vi "mainAuto.vi"() -> ()   [LabVIEW 2018]
uses:
  <vilib>/Analysis/baseanly.llb/Mean (DBL).vi
  #include/Global_1259.vi
  <userlib>/_OpenG.lib/array/array.llb/Filter 1D Array with Scalar (String)__ogtk.vi
  <userlib>/_OpenG.lib/array/array.llb/Filter 1D Array with Scalar (Boolean)__ogtk.vi
  <vilib>/Analysis/NI_AALBase.lvlib
panel:
  out "index 2":i32
  out "random 2":i32
  out "random":i32
  out "index":i32
  out "appended array":i16[](array[numeric])
  out "min(x,y)":i16
  out "max(x,y)":i16
  out "valueResistance":dbl
  out "resLower":dbl
  out "resUpper":dbl
  out "resistanceArray":dbl[](array[numeric])
  out "speedArray":dbl[](array[numeric])
  out "inclineArray":dbl[](array[numeric])
  out "negative incline":dbl
  out "FAN":string
  out "fanType":string
  out "refnum out":refnum<file>
  in  "Tab Control":T1(tab)
  out "Welcome to Console Test":picture
  out "Version":string[](array[string])
  in  "Inspection Point":string(combo)
  in  "PO Line Number":string
  in  "PO Number":string
  in  "Inspector Name":string
  in  "Work Station":string
  in  "Vendor Name":string
  in  "Vendor Number":string
  out "Initialize Test":string
  out "Config and Fixture Setup":string
  out "Firmware Reference":string
  in  "EQF1259 com port":refnum<visa-resource-name>
  out "Console Number":string
  out "Console Name":string
  in  "scanSerial":string
  out "resultSerial":bool
  out "PartNumber":string
  in  "Cos0":bool
  in  "Cos1":bool
  out "COSMETIC-3, 4":string
  in  "Con1":bool
  out "FIXTURE_SETUP-1":string
  out "Connection":picture
  out "Voltage":string
  out "Power On":cluster{dbl, dbl}(graph)
  out "Current":string
  out "POWER_UP-5, 6":string
  in  "Pow0":bool
  in  "Pow1":bool
  out "PowerOn":bool
  out "CurrentOn":bool
  out "CurrentPeak":string
  out "limitON":bool
  out "CurrentMax":string
  out "PowerMode":string="Battery"
  out "BLE_SETUP-2":string
  out "BLE_CONNECT-7":string
  out "BLE PASS":bool
  out "Cal1":bool
  in  "Dis1":bool
  in  "Dis0":bool
  out "MAINTENANCE MODE-8, 9, 10, 11":string
  in  "Enter Firmware":string
  out "Firmware":bool
  in  "Key0":bool
  in  "Key1":bool
  out "SPM AEROBIC":dbl(knob) scale=0.0..200.0
  in  "stopP":bool
  out "SPEED":dbl(knob) scale=0.0..10.1 scale format="%.1g"
  out "MAX":string
  out "PWM_RPM":string
  out "SPEED AEROBIC":dbl(knob) scale=0.0..25.0
  out "RPM AEROBIC":dbl(knob) scale=0.0..200.0
  in  "Tac0":bool
  in  "Tac1":bool
  out "Quickspeed":bool
  out "Minus\nButton":bool
  out "Plus\nButton":bool
  out "ONE\nButton":bool
  out "PWM PASS":bool
  out "PWM hz":string
  out "PWM %":string
  out "Elapsed Time (s)":dbl
  out "Press Next":dbl format="%#_13g"
  out "Decrease":bool
  out "Increase":bool
  out "Least":bool
  out "RESISTANCE-15":string
  out "QuickResistance":bool
  out "RESISTANCE/CURRENT":cluster{dbl, dbl}(graph)
  out "IRun":string
  out "IPeak":string
  out "Press Next":dbl
  out "RESISTANCE PASS":bool
  out "overCurrent":bool
  in  "stopR":bool
  out "currentMaxResistance":string
  out "BLE PULSE":u32(graph)
  out "BLE_BPM":u32
  out "PULSE-17":string
  out "Hand/Thumb Pass":bool
  out "BLE_HRM Pass":bool
  in  "E-stopHRM":bool
  in  "PUL0":bool
  in  "PUL1":bool
  out "BLE Status":u32
  out "FanCurrent":dbl(graph)
  in  "FAN0":bool
  in  "FAN1":bool
  out "Ifan":string
  out "limitFan":bool
  out "currentMaxFan":string
  out "FAN-18":string
  out "fanIPeak":string
  in  "AUD0 2":bool
  in  "AUD1 2":bool
  out "Iaudio":string
  out "AudioCurrent":dbl(graph)
  in  "AUD0":bool
  out "currentMaxAudio":string
  out "AUDIO-19":string
  out "audioIPeak":string
  in  "AUD1":bool
  out "limitAudio":bool
  in  "TV1":bool
  in  "TV0":bool
  out "TVCurrent":dbl(graph)
  out "Itv":string
  out "limitTV":bool
  out "currentMaxTV":string
  out "TV-20":string
  out "tvIPeak":string
  out "limitUSB":bool
  out "Iusb":string
  in  "USB1":bool
  in  "USB0":bool
  out "currentMaxUSB":string
  out "USBCurrent":dbl(graph)
  out "USB-16":string
  out "usbIPeak":string
  in  "stopI":bool
  out "incline":dbl(graph)
  out "INCLINE PASS":bool
  out "INCLINE-14":string
  out "Quickincline":bool
  out "Down":bool
  out "Up":bool
  out "ZERO":bool
  out "MAX":dbl
  out "MIN":dbl
  out "Press Next":dbl
  out "limitCSafe":bool
  out "Icsafe":string
  in  "CSA1":bool
  in  "CSA0":bool
  out "currentMaxCSafe":string
  out "CSafeCurrent":dbl(graph)
  out "CSAFE-21":string
  out "csafeIPeak":string
  out "limitWahoo":bool
  out "Iwahoo":string
  in  "WAH1":bool
  in  "WAH0":bool
  out "currentMaxWahoo":string
  out "WahooCurrent":dbl(graph)
  out "WAHOO-22":string
  out "wahooIPeak":string
  in  "ANO0":bool
  in  "ANO1":bool
  out "Another":picture
  out "# of Samples":i32
  out "# of Failed Samples":i32
  out "# of Passed Samples":i32
  out "Failed":picture
  out "Test Log":string
  out "Goodbye!":picture
  out "standard notepad":string
  out "standard labviewdbupload":string
  in  "FIN0":bool
  out "FINISH-25":string
  # "Does Cosmetic Pass Inspection?"
  # "Scan Console Serial Number"
  # "Is The Harness Connected Correctly?"
  # "Did Console Power ON?"
  # "Calibrate?"
  # "Display?"
  # "Key Code?"
  # "Did The Hand/Thumb Pulse Pass?"
  # "Did The Fan Function Well?"
  # "BLE Audio"
  # "Aux Audio"
  # "NOT USED. SEE BLE CONNECT AND PULSE FOR DATA."
  # "Would You Like To Test Another Console?"
  # "Console Failed Test!"
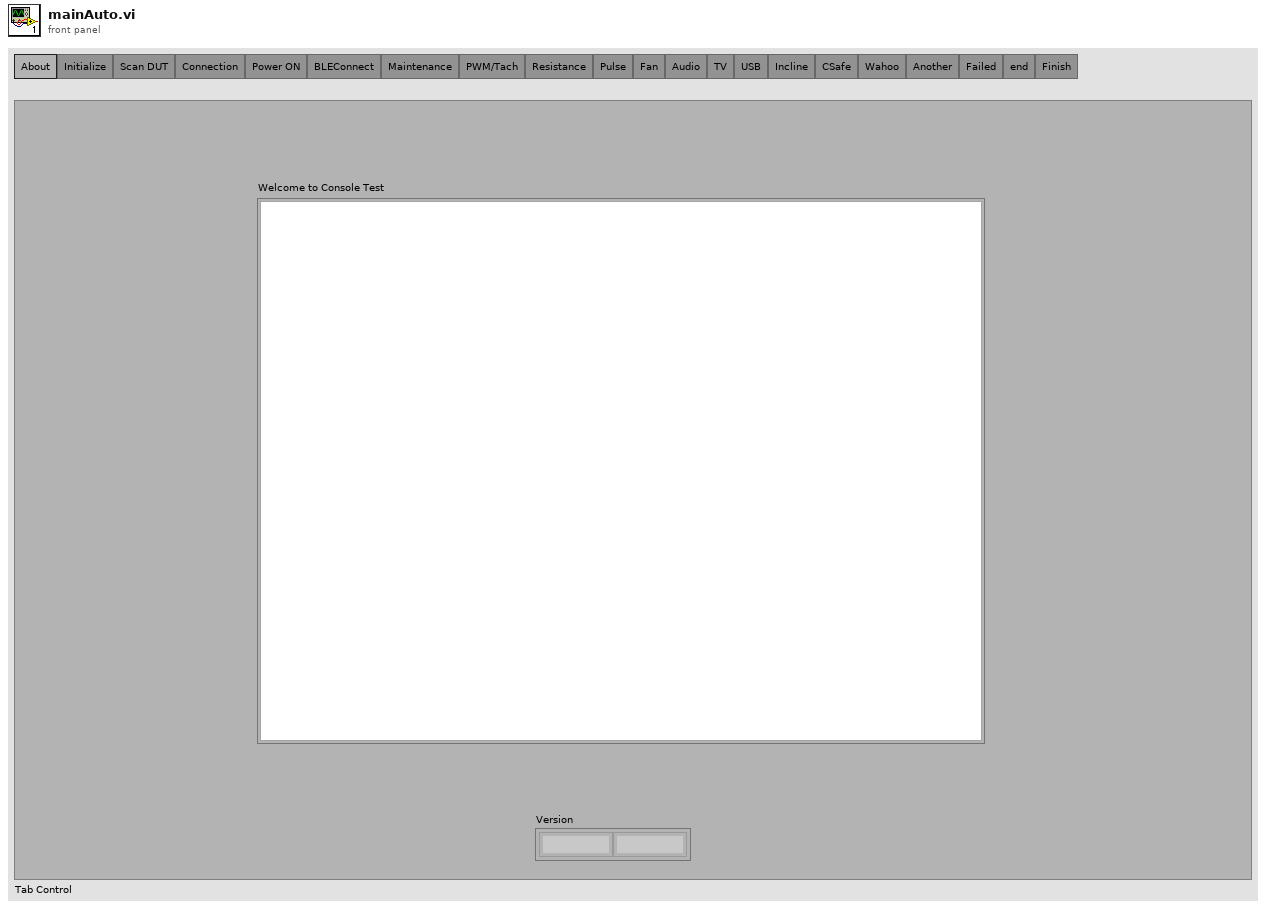
[diagram p1: front panel]
types:
  T1 = enum32{"About", "Initialize", "Scan DUT", "Connection", "Power ON", "BLEConnect", "Maintenance", "PWM/Tach", "Resistance", "Pulse", "Fan", "Audio", "TV", "USB", "Incline", "CSafe", "Wahoo", "Another", "Failed", "end", "Finish"}
  T2 = enum32{"Interactive applications", "Built-in command line utilities", "Executable command line utilities"}
  T3 = enum32{"About", "Initialize", "Scan DUT", "Connection", "Power ON", "BLEConnect", "Maintenance", "PWM/Tach", "Resistance", "Pulse", "Fan", "Audio", "TV", "USB", "Incline", "CSafe", "Wahoo", "Another", "Failed", "end"}
  T4 = enum16{"Flow", "User", "Station", "Vendor", "Number", "PO #", "PO Line#", "Record"}
  T5 = enum16{"name", "number", "device", "firmware", "mcu", "display", "grade", "resistance", "distance", "pulse"}
  T6 = enum16{"verifyHand_Thumb", "startBLE_HRM", "readBLE_HRM", "statusBLE_HRM"}
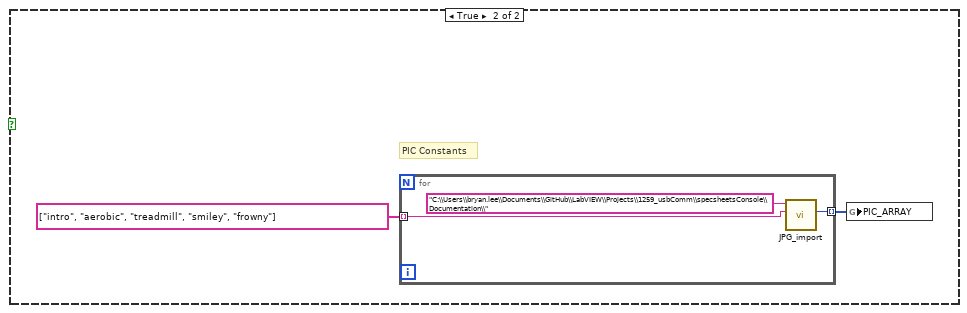
[diagram p3: hidden frame]
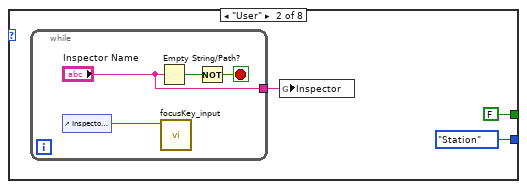
[diagram p5: hidden frame]
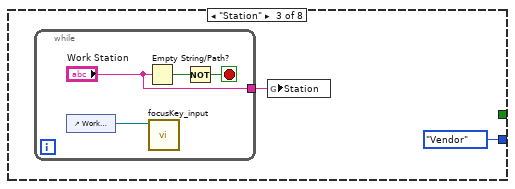
[diagram p6: hidden frame]
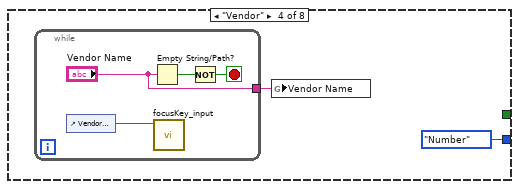
[diagram p7: hidden frame]
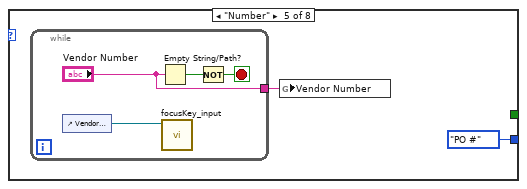
[diagram p8: hidden frame]
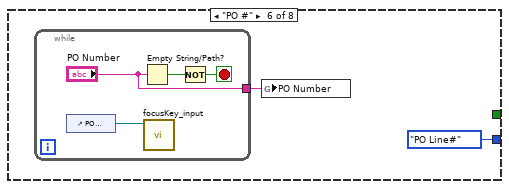
[diagram p9: hidden frame]
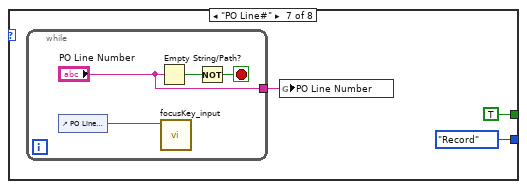
[diagram p10: hidden frame]
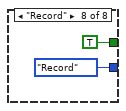
[diagram p11: hidden frame]
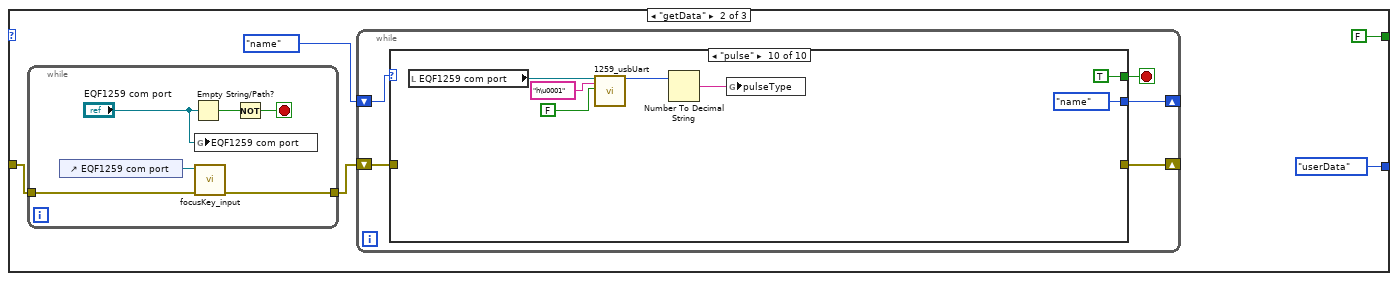
[diagram p12: hidden frame]
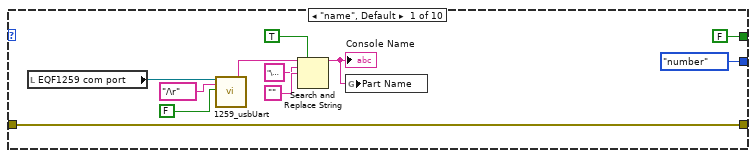
[diagram p13: hidden frame]
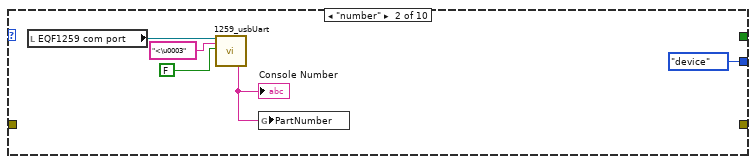
[diagram p14: hidden frame]
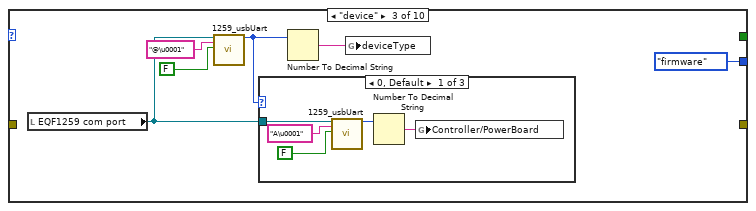
[diagram p15: hidden frame]
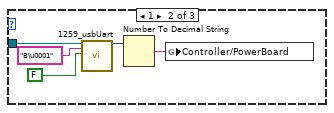
[diagram p16: hidden frame]
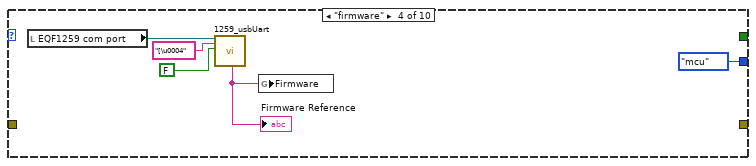
[diagram p18: hidden frame]
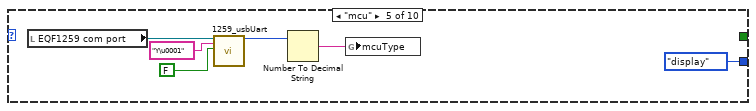
[diagram p19: hidden frame]
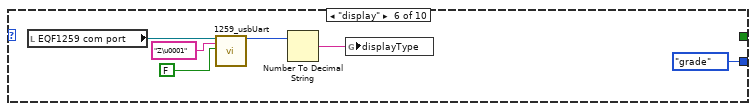
[diagram p20: hidden frame]
diagram:
  w1 = 0
  # "About\nInitialize\nScan DUT\nConnection\nPower On\nMaintenance\nSpeed/Distance\nIncline\nResistance\nFeatures\nExtra Features\nAnother\nFailed\nend"
  n1 = while {
    shift-right: [w3] -> _
    shift-left: "Tab Control" -> [w9]
    shift-right: [w5] -> _
    shift-left: w1 -> [w7]
    shift-right: [w4] -> _
    shift-left: w1 -> [w6]
    stop <- w10 stop-if-true
    n2 = property on="Tab Control" class="TabCtl (strict)"("Value"=w9) -> ("Value"=w8:T1)  [unwired: 2 in, 2 out]
    n3 = case shown="\"PWM/Tach\"" w8 {
      tunnel: [FALSE _ _ _ _ _ _ w533 w914 _ _ _ _ _ _ _ _ _ _ TRUE _] -> w10
      tunnel: [w13 T3."Connection" ("Tab Control") w225 w270 w301 w356 w422 w534 w916 w1357 w2246 w2365 w2473 w2657 w2719 w2764 w2805 w2842 T1."Finish" ("Tab Control") T3."end" ("Tab Control") w2903] -> w3
      tunnel: w7 -> [w12 w50 w218 w273 w296 w353 w419 w530 w911 w1353 w2240 w2352 w2470 w2650 w2713 w2753 w2798 w2833 w2854 w2863 w2905]
      tunnel: w6 -> [w11 w49 w223 w272 w295 w352 w418 w529 w905 w1352 w2239 w2351 w2469 w2649 w2712 w2760 w2797 w2832 w2856 w2862 w2904]
      tunnel: [w12 w50 w224 w273 w296 w353 w419 w530 w911 w1353 w2240 w2352 w2470 w2650 w2713 w2753 w2798 w2833 w2854 w2863 w2905] -> w5
      tunnel: [w11 w49 w223 w272 w295 w352 w418 w529 w905 w1352 w2239 w2351 w2469 w2649 w2712 w2760 w2797 w2832 w2855 w2862 w2904] -> w4
      frame "About", Default {
        n4 = for {
          N: 1 -> [_]
          w17 = FALSE ("Visible")
          w18 = 0
          n5 = global write "Global_1259.vi" "tempNumeric"(0.0 ("tempNumeric")) -> ()
          n6 = global write "Global_1259.vi" "tempBoolean"(FALSE) -> ()
          n7 = global write "Global_1259.vi" "tempString"("" ("tempString")) -> ()
          n8 = local write "# of Samples"(w18) -> ()
          n9 = local write "# of Failed Samples"(w18) -> ()
          n10 = case shown="False" FALSE {
            frame False {
              w32 = "\""
              # "Opens procedure"
              n11 = global read "Global_1259.vi" "PIC_ARRAY"() -> (w29:picture[])
              n12 = global read "Global_1259.vi" "Version"() -> (w22:string[][])
              n13 = Index Array(array=w29, index=0) -> (element=→"Welcome to Console Test":picture)
              n14 = for {
                N: 3 -> [_]
                tunnel: w22 -> [w39]
                tunnel: [w38] -> w25 mode=indexing
                i -> [w37]
                n15 = Index Array(array=w39, index (row)=21 ("disabled index (row)"), index (col)=w37) -> (element=w38:string)
              }
              n16 = Reshape Array(w25, 2 ("dimension size")) -> (→"Version":string[])
              n17 = call <vilib>:"Space Constant.vi"() -> ("String"=w34:string)
              n18 = Concatenate Strings("C:\\Windows\\System32\\notepad.exe" ("Command"), w34, w32, "C:\\specsheetsConsole\\Documentation\\Console(Chinese).txt" ("string"), w32) -> (w35:string)
              n19 = call "exeCLI.vi"("Tab Control"=T2."Interactive applications", "command line (interactive)"=w35) -> ()  [unwired: 11 in, 3 out]
            }
            frame True {
              # "PIC Constants"
              n20 = for {
                tunnel: [w43] -> w41 mode=indexing
                tunnel: string[] ["intro", "aerobic", "treadmill", "smiley", "frowny"] -> [w42] mode=indexing
                n21 = call "JPG_import.vi"("File name"=w42, "File path"="C:\\Users\\bryan.lee\\Documents\\GitHub\\LabVIEW\\Projects\\1259_usbComm\\specsheetsConsole\\Documentation\\") -> ("new picture"=w43:picture)  [unwired: 7 in, 2 out]
              }
              n22 = global write "Global_1259.vi" "PIC_ARRAY"(w41) -> ()
            }
          }
          n23 = property on="speedArray" class="Arr (strict)"("Visible"=w17) -> ()  [unwired: 2 in, 2 out]
          n24 = property on="resistanceArray" class="Arr (strict)"("Visible"=w17) -> ()  [unwired: 2 in, 2 out]
          n25 = property on="inclineArray" class="Arr (strict)"("Visible"=w17) -> ()  [unwired: 2 in, 2 out]
        }
        n26 = while {
          tunnel: [T3."Initialize" ("Tab Control")] -> w13
          stop <- TRUE stop-if-true
          n27 = Wait (ms)(milliseconds to wait=u32 1500) -> ()  [unwired: 1 out]
        }
      }
      frame "Initialize" {
        # "used for debugging"
        n28 = for {
          N: 2 -> [_]
          tunnel: [w56] -> w52
          w54 = ""
          n29 = local write "Work Station"(w54) -> ()
          n30 = global write "Global_1259.vi" "mcuType"(w54) -> ()
          n31 = global write "Global_1259.vi" "Controller/PowerBoard"(w54) -> ()
          n32 = global write "Global_1259.vi" "Firmware"(w54) -> ()
          n33 = global write "Global_1259.vi" "PartNumber"(w54) -> ()
          n34 = local write "Vendor Name"(w54) -> ()
          n35 = local write "Vendor Number"(w54) -> ()
          n36 = local write "PO Number"(w54) -> ()
          n37 = local write "PO Line Number"(w54) -> ()
          n38 = local write "Console Name"(w54) -> ()
          n39 = local write "Console Number"(w54) -> ()
          n40 = local write "Firmware Reference"(w54) -> ()
          n41 = global write "Global_1259.vi" "Part Name"(w54) -> ()
          n42 = global write "Global_1259.vi" "deviceType"(w54) -> ()
          n43 = local write "Inspector Name"(w54) -> ()
          n44 = local write "Inspection Point"(w54) -> ()
          n45 = local write "EQF1259 com port"(refnum<visa-resource-name> refnum ("VISA resource name")) -> ()
          n46 = call <vilib>:"Simple Error Handler.vi"() -> ("error out"=w56:errorcluster)  [unwired: 5 in, 4 out]
          "Initialize Test" <- "\u0006\\&^\tgMneöNvm\u0000i\u0000c\u0000r\u0000o\u0000S\u0000D\u0000ÒceQE\u0000Q\u0000F\u00001\u00002\u00005\u00009\u0000\u00020\n\u0000\u0000_/TE\u0000Q\u0000F\u00001\u00002\u00005\u00009\u0000\u00020\n\u0000(WE\u0000Q\u0000F\u00001\u00002\u00005\u00009\u0000\nN\fÿ\tébv^ R}cknxvMneöN\u00020\n\u0000(W\u000bNbvh<h\nNkXQáOo`\u00020\n\u0000\tébE\u0000Q\u0000F\u00001\u00002\u00005\u00009\u0000\u001a¯ïzãS\u00020\n\u0000I\u0000n\u0000s\u0000e\u0000r\u0000t\u0000 \u0000m\u0000i\u0000c\u0000r\u0000o\u0000S\u0000D\u0000 \u0000w\u0000i\u0000t\u0000h\u0000 \u0000p\u0000r\u0000o\u0000f\u0000i\u0000l\u0000e\u0000 \u0000i\u0000n\u0000t\u0000o\u0000 \u0000E\u0000Q\u0000F\u00001\u00002\u00005\u00009\u0000.\u0000\n\u0000T\u0000u\u0000r\u0000n\u0000 \u0000o\u0000n\u0000 \u0000E\u0000Q\u0000F\u00001\u00002\u00005\u00009\u0000.\u0000\n\u0000O\u0000n\u0000 \u0000t\u0000h\u0000e\u0000 \u0000E\u0000Q\u0000F\u00001\u00002\u00005\u00009\u0000,\u0000 \u0000s\u0000e\u0000l\u0000e\u0000c\u0000t\u0000 \u0000a\u0000n\u0000d\u0000 \u0000l\u0000o\u0000a\u0000d\u0000 \u0000t\u0000h\u0000e\u0000 \u0000c\u0000o\u0000r\u0000r\u0000e\u0000c\u0000t\u0000 \u0000c\u0000o\u0000n\u0000f\u0000i\u0000g\u0000u\u0000r\u0000a\u0000t\u0000i\u0000o\u0000n\u0000 \u0000f\u0000i\u0000l\u0000e\u0000.\u0000\n\u0000F\u0000i\u0000l\u0000l\u0000 \u0000o\u0000u\u0000t\u0000 \u0000t\u0000h\u0000e\u0000 \u0000i\u0000n\u0000f\u0000o\u0000r\u0000m\u0000a\u0000t\u0000i\u0000o\u0000n\u0000 \u0000o\u0000n\u0000 \u0000t\u0000h\u0000e\u0000 \u0000f\u0000o\u0000r\u0000m\u0000 \u0000b\u0000e\u0000l\u0000o\u0000w\u0000.\u0000\n\u0000S\u0000e\u0000l\u0000e\u0000c\u0000t\u0000 \u0000t\u0000h\u0000e\u0000 \u0000E\u0000Q\u0000F\u00001\u00002\u00005\u00009\u0000 \u0000c\u0000o\u0000m\u0000m\u0000u\u0000n\u0000i\u0000c\u0000a\u0000t\u0000i\u0000o\u0000n\u0000 \u0000p\u0000o\u0000r\u0000t\u0000.\u0000"
          "Config and Fixture Setup" <- "\u0006\\5un¿~Þ¥c0RE\u0000Q\u0000F\u00001\u00002\u00005\u00009\u0000\u00020\n\u0000¾nopwQMn\u001aÿ\n\u0000O(uP\u0000C\u0000\u0006\\.\u0000x\u0000m\u0000l\u0000MneöN R}0Rm\u0000i\u0000c\u0000r\u0000o\u0000S\u0000D\u0000aS-N\fÿåeöN(WR\u0000N\u0000D\u0000f\u0000t\u0000p\u0000-Nv§c6RðS\rTðy\u000bN~b0R\bÿOY\u001aÿ& R\u0000N\u0000D\u0000F\u0000t\u0000p\u0000 \u0000\\\u0000 \u0000E\u0000B\u0000N\u0000T\u00000\u00002\u00001\u00001\u00007\u0000 \u0000\\\u0000 \u0000P\u0000r\u0000o\u0000c\u0000e\u0000d\u0000u\u0000r\u0000e\u0000\tÿ\u00020\n\u0000\u0006\\m\u0000i\u0000c\u0000r\u0000o\u0000S\u0000D\u0000aSb\u001dg\nNÒceQm\u0000i\u0000c\u0000r\u0000o\u0000S\u0000D\u0000aSÒcýi-N\u00020\n\u0000Sb\u0000_opwQÌbvR\u0000E\u0000S\u0000E\u0000T\u0000\tc®\u00020\n\u0000O(u\u0011T\nNT\u0011T\u000bN\tc®~b0RcknxvMneöN\u00020\n\u0000\tcE\u0000N\u0000T\u0000E\u0000R\u0000\tébMneöN\bÿO\\U^1\u0000\tÿ\u00020\n\u0000S_O\\U^3z[öe\fÿ÷I{_5\u0000Òy\fÿY\u000bN@b:y\u00020\n\u0000¾n9YwQ\t²Q\u001aÿ\n\u0000\tcE\u0000Q\u0000F\u00001\u00002\u00005\u00009\u0000 \u00002\u0000x\u0000\nNvD\u0000i\u0000s\u0000p\u0000l\u0000a\u0000y\u0000\u00020\n\u0000(WdkopwQ\nN\tc\u0000_ËY\n\u0000O(u\u0011T\nNT\u0011T\u000bN\tc®¾n:g\t²Q\u00020\n\u0000(WopwQ\nN\tc\u0000_ËY\u00020\n\u0000\tc\u0000N!k>f:y\u00020\n\u0000C\u0000o\u0000n\u0000n\u0000e\u0000c\u0000t\u0000 \u0000t\u0000h\u0000e\u0000 \u0000p\u0000o\u0000w\u0000e\u0000r\u0000 \u0000..."
        }
        n47 = while {
          shift-right: [w60] -> _
          shift-left: enum16{"getData", "userData", "recordData"}."getData" -> [w62]
          tunnel: w52 -> [w59]
          stop <- w61 stop-if-true
          n48 = case shown="\"userData\", Default" w62 {
            tunnel: [FALSE FALSE TRUE] -> w61
            tunnel: [enum16{"getData", "userData", "recordData"}."recordData" enum16{"getData", "userData", "recordData"}."userData" enum16{"getData", "userData", "recordData"}."recordData"] -> w60
            tunnel: w59 -> [_ w117 _]
            frame "userData", Default {
              n49 = while {
                shift-right: [w66] -> _
                shift-left: T4."Flow" -> [w67]
                stop <- w68 stop-if-true
                n50 = case shown="\"Flow\", Default" w67 {
                  tunnel: [_ FALSE _ _ _ _ TRUE TRUE] -> w68
                  tunnel: [T4."User" T4."Station" T4."Vendor" T4."Number" T4."PO #" T4."PO Line#" T4."Record" T4."Record"] -> w66
                  frame "Flow", Default {
                    n51 = while {
                      tunnel: ["Inspection Point"] -> w70
                      stop <- w72 stop-if-true
                      n52 = control-ref of="Inspection Point"() -> (w74:refnum<vi>)
                      n53 = Empty String/Path?(string/path="Inspection Point") -> (empty?=w73:bool)
                      n54 = call "focusKey_input.vi"("reference"=w74) -> ()  [unwired: 10 in, 1 out]
                      n55 = Not(x=w73) -> (.not. x?=w72:bool)
                    }
                    n56 = global write "Global_1259.vi" "Inspection Point"(w70) -> ()
                  }
                  frame "User" {
                    n57 = while {
                      tunnel: ["Inspector Name"] -> w76
                      stop <- w80 stop-if-true
                      n58 = control-ref of="Inspector Name"() -> (w79:refnum<vi>)
                      n59 = Empty String/Path?(string/path="Inspector Name") -> (empty?=w81:bool)
                      n60 = call "focusKey_input.vi"("reference"=w79) -> ()  [unwired: 10 in, 1 out]
                      n61 = Not(x=w81) -> (.not. x?=w80:bool)
                    }
                    n62 = global write "Global_1259.vi" "Inspector"(w76) -> ()
                  }
                  frame "Station" {
                    n63 = while {
                      tunnel: ["Work Station"] -> w83
                      stop <- w86 stop-if-true
                      n64 = control-ref of="Work Station"() -> (w85:refnum<vi>)
                      n65 = Empty String/Path?(string/path="Work Station") -> (empty?=w87:bool)
                      n66 = call "focusKey_input.vi"("reference"=w85) -> ()  [unwired: 10 in, 1 out]
                      n67 = Not(x=w87) -> (.not. x?=w86:bool)
                    }
                    n68 = global write "Global_1259.vi" "Station"(w83) -> ()
                  }
                  frame "Vendor" {
                    n69 = while {
                      tunnel: ["Vendor Name"] -> w89
                      stop <- w92 stop-if-true
                      n70 = control-ref of="Vendor Name"() -> (w91:refnum<vi>)
                      n71 = Empty String/Path?(string/path="Vendor Name") -> (empty?=w93:bool)
                      n72 = call "focusKey_input.vi"("reference"=w91) -> ()  [unwired: 10 in, 1 out]
                      n73 = Not(x=w93) -> (.not. x?=w92:bool)
                    }
                    n74 = global write "Global_1259.vi" "Vendor Name"(w89) -> ()
                  }
                  frame "Number" {
                    n75 = while {
                      tunnel: ["Vendor Number"] -> w95
                      stop <- w98 stop-if-true
                      n76 = control-ref of="Vendor Number"() -> (w97:refnum<vi>)
                      n77 = Empty String/Path?(string/path="Vendor Number") -> (empty?=w99:bool)
                      n78 = call "focusKey_input.vi"("reference"=w97) -> ()  [unwired: 10 in, 1 out]
                      n79 = Not(x=w99) -> (.not. x?=w98:bool)
                    }
                    n80 = global write "Global_1259.vi" "Vendor Number"(w95) -> ()
                  }
                  frame "PO #" {
                    n81 = while {
                      tunnel: ["PO Number"] -> w101
                      stop <- w104 stop-if-true
                      n82 = control-ref of="PO Number"() -> (w103:refnum<vi>)
                      n83 = Empty String/Path?(string/path="PO Number") -> (empty?=w105:bool)
                      n84 = call "focusKey_input.vi"("reference"=w103) -> ()  [unwired: 10 in, 1 out]
                      n85 = Not(x=w105) -> (.not. x?=w104:bool)
                    }
                    n86 = global write "Global_1259.vi" "PO Number"(w101) -> ()
                  }
                  frame "PO Line#" {
                    n87 = while {
                      tunnel: ["PO Line Number"] -> w107
                      stop <- w110 stop-if-true
                      n88 = control-ref of="PO Line Number"() -> (w112:refnum<vi>)
                      n89 = Empty String/Path?(string/path="PO Line Number") -> (empty?=w111:bool)
                      n90 = call "focusKey_input.vi"("reference"=w112) -> ()  [unwired: 10 in, 1 out]
                      n91 = Not(x=w111) -> (.not. x?=w110:bool)
                    }
                    n92 = global write "Global_1259.vi" "PO Line Number"(w107) -> ()
                  }
                  frame "Record" {
                  }
                }
              }
            }
            frame "getData" {
              n93 = while {
                tunnel: [w122] -> w118
                tunnel: w117 -> [w121]
                stop <- w123 stop-if-true
                n94 = control-ref of="EQF1259 com port"() -> (w125:refnum<vi>)
                n95 = Empty String/Path?(string/path="EQF1259 com port") -> (empty?=w124:bool)
                n96 = global write "Global_1259.vi" "EQF1259 com port"("EQF1259 com port") -> ()
                n97 = call "focusKey_input.vi"("error in (no error)"=w121, "reference"=w125) -> ("error out"=w122:errorcluster)  [unwired: 9 in]
                n98 = Not(x=w124) -> (.not. x?=w123:bool)
              }
              n99 = while {
                shift-right: [w126] -> _
                shift-left: T5."name" -> [w127]
                shift-right: [w128] -> _
                shift-left: w118 -> [w129]
                stop <- w130 stop-if-true
                n100 = case shown="\"pulse\"" w127 {
                  tunnel: [FALSE _ _ _ _ _ _ _ _ TRUE] -> w130
                  tunnel: w129 -> [w138 _ _ _ _ _ _ _ _ _]
                  tunnel: [T5."number" T5."device" T5."firmware" T5."mcu" T5."display" T5."grade" T5."resistance" T5."distance" T5."pulse" T5."name"] -> w126
                  tunnel: [w138 _ _ _ _ _ _ _ _ _] -> w128
                  frame "name", Default {
                    n101 = local read "EQF1259 com port"() -> (w139:refnum<visa-resource-name>)
                    n102 = call "1259_usbUart.vi"("VISA resource name"=w139, "write buffer"="/\r" ("write buffer buffer"), "sdFeature"=FALSE) -> ("valid byte"=w137:string)  [unwired: 1 in, 15 out]
                    n103 = Search and Replace String(replace all?=TRUE ("replace all? (F)"), input string=w137, search string="\u0000", replace string="") -> (result string=w134:string)  [unwired: 4 in, 3 out]
                    "Console Name" <- w134
                    n104 = global write "Global_1259.vi" "Part Name"(w134) -> ()
                  }
                  frame "number" {
                    n105 = local read "EQF1259 com port"() -> (w145:refnum<visa-resource-name>)
                    n106 = call "1259_usbUart.vi"("VISA resource name"=w145, "write buffer"="<\u0003" ("write buffer buffer"), "sdFeature"=FALSE) -> ("PartNumber"=w144:string)  [unwired: 1 in, 15 out]
                    "Console Number" <- w144
                    n107 = global write "Global_1259.vi" "PartNumber"(w144) -> ()
                  }
                  frame "device" {
                    n108 = local read "EQF1259 com port"() -> (w148:refnum<visa-resource-name>)
                    n109 = call "1259_usbUart.vi"("VISA resource name"=w148, "write buffer"="@\u0001" ("write buffer buffer"), "sdFeature"=FALSE) -> ("number[0]"=w149:u32)  [unwired: 1 in, 15 out]
                    n110 = case shown="0, Default" w149 {
                      tunnel: w148 -> [w154 w161 _]
                      frame 0, Default {
                        n111 = call "1259_usbUart.vi"("VISA resource name"=w154, "write buffer"="A\u0001" ("write buffer buffer"), "sdFeature"=FALSE) -> ("number[0]"=w157:u32)  [unwired: 1 in, 15 out]
                        n112 = Number To Decimal String(number=w157) -> (decimal integer string=w156:string)  [unwired: 1 in]
                        n113 = global write "Global_1259.vi" "Controller/PowerBoard"(w156) -> ()
                      }
                      frame 1 {
                        n114 = call "1259_usbUart.vi"("VISA resource name"=w161, "write buffer"="B\u0001", "sdFeature"=FALSE) -> ("number[0]"=w159:u32)  [unwired: 1 in, 15 out]
                        n115 = Number To Decimal String(number=w159) -> (decimal integer string=w160:string)  [unwired: 1 in]
                        n116 = global write "Global_1259.vi" "Controller/PowerBoard"(w160) -> ()
                      }
                      frame 3 {
                        # "Rower_Basic"
                      }
                    }
                    n117 = Number To Decimal String(number=w149) -> (decimal integer string=w152:string)  [unwired: 1 in]
                    n118 = global write "Global_1259.vi" "deviceType"(w152) -> ()
                  }
                  frame "firmware" {
                    n119 = local read "EQF1259 com port"() -> (w167:refnum<visa-resource-name>)
                    n120 = call "1259_usbUart.vi"("VISA resource name"=w167, "write buffer"="[\u0004", "sdFeature"=FALSE) -> ("BB FW"=w163:string)  [unwired: 1 in, 15 out]
                    "Firmware Reference" <- w163
                    n121 = global write "Global_1259.vi" "Firmware"(w163) -> ()
                  }
                  frame "mcu" {
                    n122 = local read "EQF1259 com port"() -> (w171:refnum<visa-resource-name>)
                    n123 = call "1259_usbUart.vi"("VISA resource name"=w171, "write buffer"="Y\u0001", "sdFeature"=FALSE) -> ("number[0]"=w173:u32)  [unwired: 1 in, 15 out]
                    n124 = Number To Decimal String(number=w173) -> (decimal integer string=w170:string)  [unwired: 1 in]
                    n125 = global write "Global_1259.vi" "mcuType"(w170) -> ()
                  }
                  frame "display" {
                    n126 = local read "EQF1259 com port"() -> (w176:refnum<visa-resource-name>)
                    n127 = call "1259_usbUart.vi"("VISA resource name"=w176, "write buffer"="Z\u0001", "sdFeature"=FALSE) -> ("number[0]"=w179:u32)  [unwired: 1 in, 15 out]
                    n128 = Number To Decimal String(number=w179) -> (decimal integer string=w177:string)  [unwired: 1 in]
                    n129 = global write "Global_1259.vi" "displayType"(w177) -> ()
                  }
                  frame "grade" {
                    n130 = local read "EQF1259 com port"() -> (w181:refnum<visa-resource-name>)
                    n131 = call "1259_usbUart.vi"("VISA resource name"=w181, "write buffer"=" \u0001", "sdFeature"=FALSE) -> ("number[0]"=w185:u32)  [unwired: 1 in, 15 out]
                    n132 = Number To Decimal String(number=w185) -> (decimal integer string=w183:string)  [unwired: 1 in]
                    n133 = global write "Global_1259.vi" "gradeType"(w183) -> ()
                  }
                  frame "resistance" {
                    n134 = local read "EQF1259 com port"() -> (w187:refnum<visa-resource-name>)
                    n135 = call "1259_usbUart.vi"("VISA resource name"=w187, "write buffer"="¡\u0001", "sdFeature"=FALSE) -> ("number[0]"=w190:u32)  [unwired: 1 in, 15 out]
                    n136 = Number To Decimal String(number=w190) -> (decimal integer string=w191:string)  [unwired: 1 in]
                    n137 = global write "Global_1259.vi" "resistanceType"(w191) -> ()
                  }
                  frame "distance" {
                    n138 = local read "EQF1259 com port"() -> (w193:refnum<visa-resource-name>)
                    n139 = call "1259_usbUart.vi"("VISA resource name"=w193, "write buffer"="›\u0001", "sdFeature"=FALSE) -> ("number[0]"=w197:u32)  [unwired: 1 in, 15 out]
                    n140 = Number To Decimal String(number=w197) -> (decimal integer string=w195:string)  [unwired: 1 in]
                    n141 = global write "Global_1259.vi" "distanceType"(w195) -> ()
                  }
                  frame "pulse" {
                    n142 = local read "EQF1259 com port"() -> (w200:refnum<visa-resource-name>)
                    n143 = call "1259_usbUart.vi"("VISA resource name"=w200, "write buffer"="h\u0001", "sdFeature"=FALSE) -> ("number[0]"=w204:u32)  [unwired: 1 in, 15 out]
                    n144 = Number To Decimal String(number=w204) -> (decimal integer string=w202:string)  [unwired: 1 in]
                    n145 = global write "Global_1259.vi" "pulseType"(w202) -> ()
                  }
                }
              }
            }
            frame "recordData" {
              # "loads the feature array"
              n146 = local read "EQF1259 com port"() -> (w212:refnum<visa-resource-name>)
              n147 = call "1259_usbUart.vi"("VISA resource name"=w212, "write buffer"="P\u0002", "sdFeature"=TRUE) -> ("error out"=w206:errorcluster)  [unwired: 1 in, 15 out]
              n148 = global read "Global_1259.vi" "Part Name"() -> (w208:string)
              n149 = call "Header data_Cnsl.vi"("base path"=path "C:/", "prompt (Create Folder)"="logsConsole", "file name"=w208, "Error In"=w206) -> ("refnum out"=→"refnum out":refnum<file>)  [unwired: 10 in, 1 out]
            }
          }
        }
      }
      frame "Scan DUT" {
        w221 = FALSE
        w228 = ""
        n150 = Increment(x=w218) -> (x+1=w224:i32)
        "# of Samples" <- w224
        n151 = local write "scanSerial"(w228) -> ()
        n152 = local write "PartNumber"(w228) -> ()
        n153 = local write "Cos0"(w221) -> ()
        n154 = local write "Cos1"(w221) -> ()
        n155 = local write "resultSerial"(w221) -> ()
        n156 = local read "refnum out"() -> (w219:refnum<file>)
        n157 = call "User data_Cnsl.vi"("refnum in"=w219) -> ("error out"=w220:errorcluster)  [unwired: 7 in, 1 out]
        n158 = call "cosmeticPIP.vi"("error in (no error)"=w220) -> ("error out"=w216:errorcluster)  [unwired: 9 in, 1 out]
        n159 = flat-sequence {
          tunnel: w216 -> [w233]
          tunnel: [w233] -> w215
          frame #0 {
            n160 = global read "Global_1259.vi" "COSMETIC-3, 4"() -> (w230:string)
            n161 = Concatenate Strings(w230, "kbÏcïSeRagb_\u0001x\u0007h~{\u00020\n\u0000S\u0000c\u0000a\u0000n\u0000 \u0000t\u0000h\u0000e\u0000 \u0000p\u0000e\u0000e\u0000l\u0000a\u0000b\u0000l\u0000e\u0000 \u0000b\u0000a\u0000r\u0000c\u0000o\u0000d\u0000e\u0000 \u0000l\u0000a\u0000b\u0000e\u0000l\u0000.\u0000\n\u0000") -> (→"COSMETIC-3, 4":string)
          }
        }
        n162 = while {
          tunnel: [w267] -> w229
          tunnel: [w261] -> w222
          tunnel: w215 -> [w260]
          stop <- w268 stop-if-true
          n163 = control-ref of="scanSerial"() -> (w266:refnum<vi>)
          n164 = Empty String/Path?(string/path="scanSerial") -> (empty?=w269:bool)
          n165 = Search/Split String(string="scanSerial", offset (0)=6) -> (substring before match=w265:string)  [unwired: 1 in, 2 out]
          n166 = call "focusKey_input.vi"("error in (no error)"=w260, "reference"=w266) -> ("error out"=w267:errorcluster)  [unwired: 9 in]
          n167 = global read "Global_1259.vi" "PartNumber"() -> (w264:string)
          "PartNumber" <- w264
          n168 = Not(x=w269) -> (.not. x?=w268:bool)
          n169 = Equal?(x=w265, y=w264) -> (x = y?=w261:bool)
          "resultSerial" <- w261
        }
        n170 = case shown="True" w222 {
          tunnel: w229 -> [_ w240]
          tunnel: [FALSE w237] -> w217
          frame False {
          }
          frame True {
            n171 = flat-sequence {
              tunnel: w240 -> [w243]
              tunnel: [w242] -> w239
              tunnel: [w241] -> w238
              tunnel: w239 -> [_]
              tunnel: w238 -> [w251]
              tunnel: [w249] -> w235
              frame #0 {
                n172 = local read "scanSerial"() -> (w245:string)
                n173 = Reverse String(1:w245) -> (0:w247:string)
                n174 = Search/Split String(string=w247, offset (0)=11) -> (substring before match=w248:string)  [unwired: 1 in, 2 out]
                n175 = local read "refnum out"() -> (w241:refnum<file>)
                n176 = Reverse String(1:w248) -> (0:w244:string)
                n177 = call "Serial data.vi"("error in"=w243, "Serial Number"=w244, "refnum in"=w241) -> ("error out"=w242:errorcluster)  [unwired: 7 in, 1 out]
              }
              frame #1 {
                n178 = while {
                  tunnel: [w255] -> w250
                  stop <- w258 stop-if-true
                  n179 = Not(x="Cos0") -> (.not. x?=w259:bool)
                  n180 = Or(x="Cos1", y="Cos0") -> (x .or. y?=w258:bool)
                  n181 = And(x="Cos1", y=w259) -> (x .and. y?=w255:bool)
                }
                n182 = case shown="True" w250 {
                  selector: w250 -> [w252 w253]
                  tunnel: w251 -> [_ w254]
                  tunnel: [w252 w253] -> w249
                  frame False {
                  }
                  frame True {
                    n183 = call "Pass_Fail.vi"("OK"=w253, "Byte Stream File in"=w254) -> ()  [unwired: 8 in, 2 out]
                  }
                }
              }
            }
            n184 = And(x=TRUE, y=w235) -> (x .and. y?=w237:bool)
          }
        }
        n185 = Select(t=T3."Power ON" ("Tab Control"), s=w217, f=T3."Failed" ("Tab Control")) -> (s? t:f=w225:T3)
      }
      frame "Connection" {
        n186 = call "controllerVoltage.vi"() -> ("error out"=w271:errorcluster)  [unwired: 11 in]
        n187 = local write "Con1"(FALSE) -> ()
        n188 = call "controllerPIP.vi"("error in (no error)"=w271) -> ("error out"=w274:errorcluster)  [unwired: 10 in, 4 out]
        n189 = global read "Global_1259.vi" "deviceType"() -> (w275:string)
        n190 = case shown="\"1\"" w275 {
          tunnel: w274 -> [_ _ _]
          frame "0", Default {
            n191 = global read "Global_1259.vi" "PIC_ARRAY"() -> (w277:picture[])
            n192 = global read "Global_1259.vi" "FIXTURE_SETUP-1"() -> (→"FIXTURE_SETUP-1":string)
            n193 = Index Array(array=w277, index=2) -> (element=→"Connection":picture)
          }
          frame "1" {
            n194 = global read "Global_1259.vi" "PIC_ARRAY"() -> (w283:picture[])
            n195 = global read "Global_1259.vi" "FIXTURE_SETUP-1"() -> (w284:string)
            n196 = Index Array(array=w283, index=1) -> (element=w281:picture)
            n197 = local write "FIXTURE_SETUP-1"(w284) -> ()
            n198 = local write "Connection"(w281) -> ()
          }
          frame "2" {
            n199 = global read "Global_1259.vi" "PIC_ARRAY"() -> (w287:picture[])
            n200 = global read "Global_1259.vi" "FIXTURE_SETUP-1"() -> (w288:string)
            n201 = Index Array(array=w287, index=1) -> (element=w285:picture)
            n202 = local write "FIXTURE_SETUP-1"(w288) -> ()
            n203 = local write "Connection"(w285) -> ()
          }
        }
        n204 = while {
          tunnel: [T3."Scan DUT" ("Tab Control")] -> w270
          stop <- "Con1" stop-if-true
        }
      }
      frame "Power ON" {
        w293 = "0.00" ("Voltage")
        w294 = FALSE
        # "current cannot be used as a stop due to battery option"
        n205 = local write "Voltage"(w293) -> ()
        n206 = local write "Current"(w293) -> ()
        n207 = local write "CurrentPeak"(w293) -> ()
        n208 = global write "Global_1259.vi" "runCurrent"(w293) -> ()
        n209 = local write "CurrentMax"(w293) -> ()
        n210 = local write "Pow1"(w294) -> ()
        n211 = local write "Pow0"(w294) -> ()
        n212 = property on="Power On" class="WFChart (strict)"("History Data"=cluster{dbl, dbl}[] []) -> ()  [unwired: 2 in, 2 out]
        n213 = local write "PowerMode"("Off" ("runCurrent")) -> ()
        n214 = global read "Global_1259.vi" "POWER_UP-5, 6"() -> (→"POWER_UP-5, 6":string)
        n215 = local write "CurrentOn"(w294) -> ()
        n216 = local write "limitON"(w294) -> ()
        n217 = local write "PowerOn"(w294) -> ()
        n218 = stacked-sequence {
          tunnel: [_ w309] -> w291
          frame #0 {
            n219 = global read "Global_1259.vi" "EQF1259 com port"() -> (w302:refnum<visa-resource-name>)
            n220 = call "currentMax.vi"("VISA Refnum in"=w302) -> ("stringCurrentMax"=w303:string)  [unwired: 8 in, 2 out]
            n221 = global write "Global_1259.vi" "maxCurrent"(w303) -> ()
          }
          frame #1 {
            n222 = while {
              tunnel: [w336] -> w309
              tunnel: [w335] -> w306
              tunnel: [w334] -> w305
              stop <- w337 stop-if-true
              n223 = global read "Global_1259.vi" "EQF1259 com port"() -> (w312:refnum<visa-resource-name>)
              n224 = call "1259_usbUart.vi"("VISA resource name"=w312, "write buffer"="j\u0001", "sdFeature"=FALSE) -> ("number[0]"=w313:u32)  [unwired: 1 in, 15 out]
              n225 = case shown="1" w313 {
                frame 0, Default {
                  w338 = "Off" ("USB")
                  n226 = local write "PowerMode"(w338) -> ()
                  n227 = global write "Global_1259.vi" "PowerMode"(w338) -> ()
                }
                frame 1 {
                  w339 = "On" ("USB")
                  # "On"
                  n228 = local read "limitON"() -> (w344:bool)
                  n229 = local read "CurrentOn"() -> (w343:bool)
                  n230 = local read "PowerOn"() -> (w342:bool)
                  n231 = Not(x=w344) -> (.not. x?=w345:bool)
                  n232 = Compound Arithmetic op=OR(TRUE, w342, w343, w345) -> (w340:bool)
                  n233 = local write "PowerMode"(w339) -> ()
                  n234 = global write "Global_1259.vi" "PowerMode"(w339) -> ()
                  n235 = local write "Pow1"(w340) -> ()
                }
                frame 2 {
                  w346 = "Battery" ("USB")
                  # "Battery"
                  n236 = global write "Global_1259.vi" "PowerMode"(w346) -> ()
                  "PowerMode" <- w346
                }
              }
              n237 = global read "Global_1259.vi" "EQF1259 com port"() -> (w315:refnum<visa-resource-name>)
              n238 = global read "Global_1259.vi" "ConsoleVoltage"() -> (w317:string)
              n239 = global read "Global_1259.vi" "maxCurrent"() -> (w314:string)
              "CurrentMax" <- w314
              n240 = Fract/Exp String To Number(string=w317) -> (number=w316:dbl)  [unwired: 3 in, 1 out]
              n241 = call "voltageScan.vi"("VISA Refnum in"=w315) -> ("error out"=w329:errorcluster, "stringVoltage"=w334:string, "numberVoltage"=w324:dbl)  [unwired: 8 in]
              "Voltage" <- w334
              n242 = Greater?(x=w324, y=w316) -> (0:→"PowerOn":bool)
              n243 = call "currentScan.vi"("error in (no error)"=w329, "Imax"=w314, "VISA resource name"=w315) -> ("error out"=w328:errorcluster, "max"=w325:bool, "Istring"=w319:string, "Ichart"=w322:dbl)  [unwired: 5 in]
              "limitON" <- w325
              n244 = Compound Arithmetic op=OR("Pow1", "Pow0", w325) -> (w337:bool)
              n245 = Not(x="Pow0") -> (.not. x?=w332:bool)
              n246 = Not(x=w325) -> (.not. x?=w326:bool)
              n247 = call "currentPeak.vi"("error in (no error)"=w328, "Istring# change"=w319, "Istring# scan"=w319) -> ("Ipeak"=w335:string, "Irun"=→"Current":string)  [unwired: 6 in, 1 out]
              "CurrentPeak" <- w335
              n248 = Bundle("numberVoltage"=w324, "Ichart"=w322) -> (→"Power On":cluster{"\nnumberVoltage":dbl, "Ichart":dbl})  [unwired: 1 in]
              n249 = Greater?(x=w322, y=0.0) -> (0:→"CurrentOn":bool)
              n250 = Compound Arithmetic op=AND(TRUE ("value"), w326, "Pow1", w332) -> (w336:bool)
            }
            n251 = local read "refnum out"() -> (w307:refnum<file>)
            n252 = call "dataSampled.vi"("Data"=w305, "refnum in"=w307) -> ("error out"=w304:errorcluster, "refnum out"=w308:refnum<file>)  [unwired: 8 in]
            n253 = call "dataSampled.vi"("Error In"=w304, "Data"=w306, "refnum in"=w308) -> ()  [unwired: 7 in, 2 out]
          }
        }
        n254 = Select(t=T3."Maintenance" ("Tab Control"), s=w291, f=T3."Failed" ("Tab Control")) -> (s? t:f=w301:T3)
      }
      frame "BLEConnect" {
        n255 = local write "BLE PASS"(FALSE ("BLE PASS")) -> ()
        n256 = global read "Global_1259.vi" "Inspection Point"() -> (w349:string)
        n257 = Equal?(x=w349, y="SubAssembly") -> (x = y?=w347:bool)
        n258 = case shown="False" w347 {
          tunnel: [TRUE w362] -> w351
          frame True {
            n259 = local read "refnum out"() -> (w357:refnum<file>)
            n260 = call "dataSampled.vi"("refnum in"=w357) -> ()  [unwired: 9 in, 2 out]
          }
          frame False {
            n261 = global read "Global_1259.vi" "WAHOO"() -> (w361:string)
            n262 = Not Equal?(x=w361, y="1") -> (x != y?=w359:bool)
            n263 = case shown="True" w359 {
              tunnel: [w363 w388] -> w362
              frame False {
                w367 = 2 ("index (row)")
                # "ANT+ SamplerApp"
                n264 = global read "Global_1259.vi" "PIP_Instruction"() -> (w370:string[][])
                n265 = global write "Global_1259.vi" "pulseType"("16" ("pulseType")) -> ()
                n266 = Index Array(array=w370, index (row) #1=w367, index (col) #1=w367, index (row) #2=w367, index (col) #2=7 ("disabled index (col)")) -> (element #1=w365:string, element #2=w366:string)
                n267 = global write "Global_1259.vi" "BLE_SETUP-2"(w365) -> ()
                n268 = local write "BLE_SETUP-2"(w365) -> ()
                n269 = global write "Global_1259.vi" "BLE_CONNECT-7"(w366) -> ()
                n270 = local write "BLE_CONNECT-7"(w366) -> ()
                n271 = while {
                  tunnel: [w382] -> w364
                  stop <- w380 stop-if-true
                  n272 = local read "EQF1259 com port"() -> (w375:refnum<visa-resource-name>)
                  n273 = call "1259_usbUart.vi"("VISA resource name"=w375, "write buffer"="†\u0001") -> ("number[0]"=w377:u32)  [unwired: 2 in, 15 out]
                  n274 = Number To Decimal String(number=w377, width (-)=i16 0) -> (decimal integer string=w374:string)
                  n275 = Not Equal?(x=w374, y="0") -> (x != y?=w382:bool)
                  n276 = feedback #1() -> (w379:bool)  [unwired: 1 in]
                  n277 = call "Elapsed Time3"("Reset"=w379) -> ("Time has Elapsed"=w381:bool)  [unwired: 11 in, 7 out]
                  n278 = Or(x=w382, y=w381) -> (x .or. y?=w380:bool)
                  n279 = feedback-in #1(w380) -> ()
                }
                n280 = local write "BLE PASS"(w364) -> ()
                n281 = case shown="True" w364 {
                  selector: w364 -> [w371 w372]
                  tunnel: [w371 w372] -> w363
                  frame False {
                  }
                  frame True {
                    n282 = local read "refnum out"() -> (w373:refnum<file>)
                    n283 = call "Pass_Fail.vi"("OK"=w372, "Byte Stream File in"=w373) -> ()  [unwired: 8 in, 2 out]
                  }
                }
              }
              frame True {
                n284 = global read "Global_1259.vi" "TABLET"() -> (w386:string)
                n285 = Equal?(x=w386, y="0") -> (x = y?=w384:bool)
                n286 = case shown="True" w384 {
                  tunnel: [FALSE w390] -> w387
                  frame False {
                  }
                  frame True {
                    n287 = global read "Global_1259.vi" "BLE"() -> (w392:string)
                    n288 = Equal?(x=w392, y="1") -> (x = y?=w390:bool)
                  }
                }
                n289 = case shown="True" w387 {
                  tunnel: [TRUE w395] -> w388
                  frame False {
                    n290 = local read "refnum out"() -> (w394:refnum<file>)
                    n291 = call "dataSampled.vi"("refnum in"=w394) -> ()  [unwired: 9 in, 2 out]
                  }
                  frame True {
                    w397 = 1 ("index (row)")
                    # "BLE_CardioApp"
                    n292 = global read "Global_1259.vi" "PIP_Instruction"() -> (w402:string[][])
                    n293 = while {
                      tunnel: [w411] -> w396
                      stop <- w412 stop-if-true
                      n294 = local read "EQF1259 com port"() -> (w408:refnum<visa-resource-name>)
                      n295 = call "1259_usbUart.vi"("VISA resource name"=w408, "write buffer"="†\u0001") -> ("binary[0] String"=w406:string)  [unwired: 2 in, 15 out]
                      n296 = Not Equal?(x="0" ("y"), y=w406) -> (x != y?=w411:bool)
                      n297 = feedback #2() -> (w410:bool)  [unwired: 1 in]
                      n298 = call "Elapsed Time2"("Reset"=w410) -> ("Time has Elapsed"=w413:bool)  [unwired: 11 in, 7 out]
                      n299 = Or(x=w411, y=w413) -> (x .or. y?=w412:bool)
                      n300 = feedback-in #2(w412) -> ()
                    }
                    "BLE PASS" <- w396
                    n301 = Index Array(array=w402, index (row) #1=w397, index (col) #1=2 ("disabled index (col)"), index (row) #2=w397, index (col) #2=7 ("disabled index (col)")) -> (element #1=w401:string, element #2=w400:string)
                    "BLE_SETUP-2" <- w401
                    "BLE_CONNECT-7" <- w400
                    n302 = global write "Global_1259.vi" "BLE_SETUP-2"(w401) -> ()
                    n303 = global write "Global_1259.vi" "BLE_CONNECT-7"(w400) -> ()
                    n304 = case shown="True" w396 {
                      selector: w396 -> [w403 w404]
                      tunnel: [w403 w404] -> w395
                      frame False {
                      }
                      frame True {
                        n305 = local read "refnum out"() -> (w405:refnum<file>)
                        n306 = call "Pass_Fail.vi"("OK"=w404, "Byte Stream File in"=w405) -> ()  [unwired: 8 in, 2 out]
                      }
                    }
                  }
                }
              }
            }
          }
        }
        n307 = Select(t=T3."PWM/Tach" ("Tab Control"), s=w351, f=T3."Failed" ("Tab Control")) -> (s? t:f=w356:T3)
      }
      frame "Maintenance" {
        w414 = ""
        w417 = FALSE
        (unwired) FALSE
        n308 = local write "Enter Firmware"(w414) -> ()
        n309 = global write "Global_1259.vi" "BaseCurrent"(w414) -> ()
        n310 = local write "Cal1"(w417) -> ()
        n311 = local write "Dis1"(w417) -> ()
        n312 = local write "Key0"(w417) -> ()
        n313 = local write "Key1"(w417) -> ()
        n314 = local write "Dis0"(w417) -> ()
        n315 = local write "Firmware"(w417) -> ()
        n316 = while {
          shift-right: [w425] -> _
          shift-left: 0 -> [w426]
          tunnel: [w423] -> w420
          stop <- w424 stop-if-true
          n317 = case shown="3" w426 {
            tunnel: [1 2 3 4 5 6 _] -> w425
            tunnel: [FALSE FALSE FALSE w455 w484 w498 w512] -> w424
            tunnel: [FALSE FALSE FALSE w456 w485 w499 w513] -> w423
            frame 0, Default {
              n318 = local read "EQF1259 com port"() -> (w428:refnum<visa-resource-name>)
              n319 = call "1259_usbUart.vi"("VISA resource name"=w428, "write buffer"="\u0001", "sdFeature"=FALSE) -> ("PartNumber"=w437:string, "error out"=w427:errorcluster)  [unwired: 1 in, 14 out]
              n320 = global write "Global_1259.vi" "buttonType"(w437) -> ()
              n321 = call "1259_usbUart.vi"("VISA resource name"=w428, "write buffer"="š\u0001", "sdFeature"=FALSE, "error in (no error)"=w427) -> ("PartNumber"=w431:string)  [unwired: 15 out]
              n322 = global write "Global_1259.vi" "tabletType"(w431) -> ()
            }
            frame 1 {
              n323 = global read "Global_1259.vi" "GRADE"() -> (w441:string)
              n324 = case shown="\"0\"" w441 {
                frame "1", Default {
                  n325 = property on="Cal1" class="Bool (strict)"("Visible"=TRUE) -> ()  [unwired: 2 in, 2 out]
                }
                frame "0" {
                  n326 = local write "Cal1"(TRUE) -> ()
                  n327 = property on="Cal1" class="Bool (strict)"("Visible"=FALSE) -> ()  [unwired: 2 in, 2 out]
                }
              }
              n328 = call "maintenancePIP.vi"() -> ("MAINTENANCE MODE-8, 9, 10, 11"=→"MAINTENANCE MODE-8, 9, 10, 11":string)  [unwired: 10 in, 1 out]
            }
            frame 2 {
              n329 = while {
                tunnel: ["Enter Firmware"] -> w448
                stop <- w453 stop-if-true
                n330 = control-ref of="Enter Firmware"() -> (w452:refnum<vi>)
                n331 = Empty String/Path?(string/path="Enter Firmware") -> (empty?=w454:bool)
                n332 = call "focusKey_input.vi"("reference"=w452) -> ()  [unwired: 10 in, 1 out]
                n333 = Not(x=w454) -> (.not. x?=w453:bool)
                "Firmware" <- w453
              }
              n334 = local read "refnum out"() -> (w449:refnum<file>)
              n335 = call "dataSampled.vi"("Data"=w448, "refnum in"=w449) -> ()  [unwired: 8 in, 2 out]
            }
            frame 3 {
              n336 = local read "Cal1"() -> (w457:bool)
              n337 = case shown="False" w457 {
                tunnel: [FALSE w472] -> w456
                tunnel: [FALSE w471] -> w455
                frame True {
                  # "This is 1 second / per 10 samples"
                  n338 = while {
                    tunnel: [w470] -> w462 mode=indexing
                    i -> [w468]
                    stop <- w469 stop-if-true
                    n339 = local read "EQF1259 com port"() -> (w466:refnum<visa-resource-name>)
                    n340 = Equal?(x=25, y=w468) -> (x = y?=w469:bool)
                    n341 = call "currentScan.vi"("VISA resource name"=w466) -> ("Ichart"=w470:dbl)  [unwired: 7 in, 3 out]
                  }
                  n342 = local read "refnum out"() -> (w465:refnum<file>)
                  n343 = call-poly <vilib>:"Mean.vi"("X"=w462) -> ("mean"=w461:dbl)  [unwired: 1 out]
                  n344 = call "dataSampled.vi"("refnum in"=w465) -> ()  [unwired: 9 in, 2 out]
                  n345 = Number To Fractional String(number=w461, precision (6)=i16 2) -> (F-format string=w460:string)  [unwired: 2 in]
                  n346 = global write "Global_1259.vi" "BaseCurrent"(w460) -> ()
                }
                frame False {
                  n347 = flat-sequence {
                    tunnel: [w474] -> w473
                    tunnel: w473 -> [w478]
                    tunnel: [w477] -> w472
                    tunnel: [w476] -> w471
                    frame #0 {
                      # "engineer mode on fixture"
                      n348 = local read "EQF1259 com port"() -> (w475:refnum<visa-resource-name>)
                      n349 = call "inclineCalibrate.vi"("VISA Refnum in"=w475) -> ("Complete"=w474:bool)  [unwired: 8 in, 2 out]
                    }
                    frame #1 {
                      n350 = case shown="False" w478 {
                        selector: w478 -> [w480 w482]
                        tunnel: [w480 w482] -> w477
                        tunnel: [w479 w481] -> w476
                        frame False {
                          n351 = Not(x=w480) -> (.not. x?=w479:bool)
                        }
                        frame True {
                          n352 = Not(x=w482) -> (.not. x?=w481:bool)
                          n353 = local read "refnum out"() -> (w483:refnum<file>)
                          n354 = call "Pass_Fail.vi"("OK"=w482, "Byte Stream File in"=w483) -> ()  [unwired: 8 in, 2 out]
                        }
                      }
                      "Cal1" <- w478
                    }
                  }
                }
              }
            }
            frame 4 {
              n355 = while {
                tunnel: [w496] -> w486
                stop <- w495 stop-if-true
                n356 = Not(x="Dis0") -> (.not. x?=w497:bool)
                n357 = Or(x="Dis1", y="Dis0") -> (x .or. y?=w495:bool)
                n358 = And(x="Dis1", y=w497) -> (x .and. y?=w496:bool)
              }
              n359 = case shown="True" w486 {
                selector: w486 -> [w488 w491]
                tunnel: [w488 w491] -> w485
                tunnel: [w489 w490] -> w484
                frame False {
                  n360 = Not(x=w488) -> (.not. x?=w489:bool)
                }
                frame True {
                  n361 = Not(x=w491) -> (.not. x?=w490:bool)
                  n362 = local read "refnum out"() -> (w492:refnum<file>)
                  n363 = call "Pass_Fail.vi"("OK"=w491, "Byte Stream File in"=w492) -> ()  [unwired: 8 in, 2 out]
                }
              }
            }
            frame 5 {
              n364 = while {
                tunnel: [w510] -> w500
                stop <- w509 stop-if-true
                n365 = Not(x="Key0") -> (.not. x?=w511:bool)
                n366 = Or(x="Key1", y="Key0") -> (x .or. y?=w509:bool)
                n367 = And(x="Key1", y=w511) -> (x .and. y?=w510:bool)
              }
              n368 = case shown="True" w500 {
                selector: w500 -> [w503 w505]
                tunnel: [w503 w505] -> w499
                tunnel: [w502 w504] -> w498
                frame False {
                  n369 = Not(x=w503) -> (.not. x?=w502:bool)
                }
                frame True {
                  n370 = Not(x=w505) -> (.not. x?=w504:bool)
                  n371 = local read "refnum out"() -> (w506:refnum<file>)
                  n372 = call "Pass_Fail.vi"("OK"=w505, "Byte Stream File in"=w506) -> ()  [unwired: 8 in, 2 out]
                }
              }
            }
            frame 6 {
              n373 = while {
                tunnel: [w518] -> w513
                tunnel: [w517] -> w512
                stop <- w517 stop-if-true
                n374 = local read "Key1"() -> (w516:bool)
                n375 = local read "Cal1"() -> (w515:bool)
                n376 = local read "Dis1"() -> (w520:bool)
                n377 = Compound Arithmetic op=AND(TRUE ("value"), w515, w520, w516) -> (w518:bool)
                n378 = Not(x=w518) -> (.not. x?=w519:bool)
                n379 = Or(x=w518, y=w519) -> (x .or. y?=w517:bool)
              }
            }
          }
        }
        n380 = Select(t=T3."BLEConnect" ("Tab Control"), s=w420, f=T3."Failed" ("Tab Control")) -> (s? t:f=w422:T3)
      }
      frame "PWM/Tach" {
        w525 = 0.0 ("Press Next")
        w527 = FALSE ("stop")
        n381 = local write "SPEED"(w525) -> ()
        n382 = local write "Plus\nButton"(w527) -> ()
        n383 = local write "Minus\nButton"(w527) -> ()
        n384 = local write "Quickspeed"(w527) -> ()
        n385 = local write "ONE\nButton"(w527) -> ()
        n386 = local write "PWM PASS"(w527) -> ()
        n387 = local write "speedArray"(dbl[] [0.0] ("Array")) -> ()
        n388 = local write "Press Next"(w525) -> ()
        n389 = global read "Global_1259.vi" "deviceType"() -> (w523:string)
        n390 = Decimal String To Number(string=w523) -> (number=w524:i32)  [unwired: 2 in, 1 out]
        n391 = Not Equal To 0?(x=w524) -> (x != 0?=w522:bool)
        n392 = case shown="True" w522 {
          tunnel: ["0" "1"] -> w521
          frame False {
            # "Treadmill"
          }
          frame True {
            # "Aerobic"
          }
        }
        n393 = case shown="\"0\", Default" w521 {
          tunnel: [w552 w610] -> w528
          tunnel: [w551 FALSE ("E-Stop")] -> w533
          frame "1" {
            w546 = 0.0 ("SPEED AEROBIC")
            w547 = FALSE ("Visible")
            w545 = TRUE
            w553 = FALSE ("Visible")
            # "Aerobic"
            # "Quick_Keys"
            n394 = property on="MAX" class="Str"("Visible"=w547) -> ()  [unwired: 2 in, 2 out]
            n395 = property on="speedArray" class="Arr (strict)"("Visible"=w547) -> ()  [unwired: 2 in, 2 out]
            n396 = property on="Quickspeed" class="Bool (strict)"("Visible"=w547) -> ()  [unwired: 2 in, 2 out]
            n397 = property on="ONE\nButton" class="Bool (strict)"("Visible"=w547) -> ()  [unwired: 2 in, 2 out]
            n398 = property on="PWM PASS" class="Bool (strict)"("Visible"=w547) -> ()  [unwired: 2 in, 2 out]
            n399 = property on="Plus\nButton" class="Bool (strict)"("Visible"=w547) -> ()  [unwired: 2 in, 2 out]
            n400 = property on="Press Next" class="DigNum (strict)"("Visible"=w547) -> ()  [unwired: 2 in, 2 out]
            n401 = property on="Minus\nButton" class="Bool (strict)"("Visible"=w547) -> ()  [unwired: 2 in, 2 out]
            n402 = property on="PWM hz" class="Str"("Visible"=w547) -> ()  [unwired: 2 in, 2 out]
            n403 = property on="PWM %" class="Str"("Visible"=w547) -> ()  [unwired: 2 in, 2 out]
            n404 = property on="SPEED" class="Knob (strict)"("Visible"=FALSE) -> ()  [unwired: 2 in, 2 out]
            n405 = property on="RPM AEROBIC" class="Knob (strict)"("Visible"=w545) -> ()  [unwired: 2 in, 2 out]
            n406 = property on="SPEED AEROBIC" class="Knob (strict)"("Visible"=w545) -> ()  [unwired: 2 in, 2 out]
            n407 = property on="Tac1" class="Bool (strict)"("Visible"=w545) -> ()  [unwired: 2 in, 2 out]
            n408 = property on="Tac0" class="Bool (strict)"("Visible"=w545) -> ()  [unwired: 2 in, 2 out]
            n409 = local write "Tac1"(w553) -> ()
            n410 = local write "Tac0"(w553) -> ()
            n411 = for {
              N: 1 -> [_]
              tunnel: [w562] -> w539
              tunnel: [w559] -> w538
              n412 = call "pwm_rpmPIP.vi"() -> ("error out"=w560:errorcluster, "PWM_RPM"=w563:string)  [unwired: 10 in]
              n413 = local read "EQF1259 com port"() -> (w561:refnum<visa-resource-name>)
              n414 = local write "PWM_RPM"(w563) -> ()
              n415 = Wait (ms)(milliseconds to wait=u32 250) -> ()  [unwired: 1 out]
              n416 = call "speedSet.vi"("error in (no error)"=w560, "VISA resource name"=w561) -> ("error out (no error)"=w559:errorcluster, "Running"=w562:bool)  [unwired: 2 in, 6 out]
            }
            n417 = property on="SPM AEROBIC" class="Knob (strict)"("Visible"=w545) -> ()  [unwired: 2 in, 2 out]
            n418 = local write "RPM AEROBIC"(w546) -> ()
            n419 = local write "SPEED AEROBIC"(w546) -> ()
            n420 = local write "SPM AEROBIC"(w546) -> ()
            n421 = while {
              tunnel: [w572] -> w549
              tunnel: [w571] -> w550
              tunnel: [w568] -> w552
              tunnel: [w567] -> w551
              shift-right: [w565] -> _
              shift-left: w539 -> [w566]
              tunnel: w538 -> [_]
              tunnel: [w564] -> w540
              stop <- w570 stop-if-true
              n422 = feedback #3() -> (w569:bool)  [unwired: 1 in]
              n423 = case shown="True" w566 {
                tunnel: [w575 w590] -> w570
                tunnel: [w573 w593] -> w572
                tunnel: [w573 w592] -> w571
                tunnel: w569 -> [_ w591]
                tunnel: [w575 w585] -> w568
                tunnel: [w575 FALSE ("E-Stop")] -> w567
                tunnel: [TRUE TRUE] -> w565
                tunnel: [w573 w579] -> w564
                frame False {
                  w573 = ""
                  w575 = FALSE
                  n424 = local read "EQF1259 com port"() -> (w578:refnum<visa-resource-name>)
                  n425 = call "1259_usbCommand.vi"("write buffer"="\u0005\u0004", "VISA resource name in"=w578) -> ()  [unwired: 8 in, 2 out]
                  n426 = Wait (ms)(milliseconds to wait=u32 250) -> ()  [unwired: 1 out]
                }
                frame True {
                  n427 = call "Elapsed Time"("Reset"=w591) -> ("Elapsed Time (s)"=→"Elapsed Time (s)":dbl, "Time has Elapsed"=w584:bool)  [unwired: 11 in, 6 out]
                  n428 = local read "EQF1259 com port"() -> (w596:refnum<visa-resource-name>)
                  n429 = call "speedSet.vi"("VISA resource name"=w596) -> ("spm"=w579:string, "rpm"=w592:string, "speed"=w593:string, "RPM"=→"RPM AEROBIC":dbl, "SPEED"=→"SPEED AEROBIC":dbl, "SPM"=→"SPM AEROBIC":dbl)  [unwired: 3 in, 2 out]
                  n430 = Or(x="Tac1", y="Tac0") -> (x .or. y?=w586:bool)
                  n431 = Not(x="Tac0") -> (.not. x?=w589:bool)
                  n432 = And(x="Tac1", y=w589) -> (x .and. y?=w585:bool)
                  n433 = Compound Arithmetic op=OR(w586, w584) -> (w590:bool)
                }
              }
              n434 = feedback-in #3(w570) -> ()
            }
            n435 = local read "refnum out"() -> (w556:refnum<file>)
            n436 = call "dataSampled.vi"("Data"=w549, "refnum in"=w556) -> ("error out"=w555:errorcluster, "refnum out"=w557:refnum<file>)  [unwired: 8 in]
            n437 = call "dataSampled.vi"("Error In"=w555, "Data"=w550, "refnum in"=w557) -> ("error out"=w542:errorcluster, "refnum out"=w541:refnum<file>)  [unwired: 7 in]
            n438 = call "dataSampled.vi"("Error In"=w542, "Data"=w540, "refnum in"=w541) -> ("error out"=w543:errorcluster, "refnum out"=w544:refnum<file>)  [unwired: 7 in]
            n439 = for {
              N: 7 -> [_]
              tunnel: w544 -> [w598]
              tunnel: w543 -> [w597]
              n440 = call "dataSampled.vi"("Error In"=w597, "refnum in"=w598) -> ()  [unwired: 8 in, 2 out]
            }
          }
          frame "0", Default {
            w600 = FALSE
            w606 = TRUE ("Visible")
            # "Treadmill"
            # "No E-STOP"
            n441 = property on="RPM AEROBIC" class="Knob (strict)"("Visible"=w600) -> ()  [unwired: 2 in, 2 out]
            n442 = property on="Tac1" class="Bool (strict)"("Visible"=w600) -> ()  [unwired: 2 in, 2 out]
            n443 = property on="Tac0" class="Bool (strict)"("Visible"=w600) -> ()  [unwired: 2 in, 2 out]
            n444 = property on="Elapsed Time (s)" class="DigNum (strict)"("Visible"=w600) -> ()  [unwired: 2 in, 2 out]
            n445 = property on="SPEED AEROBIC" class="Knob (strict)"("Visible"=w600) -> ()  [unwired: 2 in, 2 out]
            n446 = property on="MAX" class="Str"("Visible"=w606) -> ()  [unwired: 2 in, 2 out]
            n447 = property on="PWM PASS" class="Bool (strict)"("Visible"=w606) -> ()  [unwired: 2 in, 2 out]
            n448 = property on="Press Next" class="DigNum (strict)"("Visible"=w606) -> ()  [unwired: 2 in, 2 out]
            n449 = property on="Plus\nButton" class="Bool (strict)"("Visible"=w606) -> ()  [unwired: 2 in, 2 out]
            n450 = property on="Quickspeed" class="Bool (strict)"("Visible"=w606) -> ()  [unwired: 2 in, 2 out]
            n451 = property on="ONE\nButton" class="Bool (strict)"("Visible"=w606) -> ()  [unwired: 2 in, 2 out]
            n452 = property on="SPEED" class="Knob (strict)"("Visible"=w606) -> ()  [unwired: 2 in, 2 out]
            n453 = property on="Minus\nButton" class="Bool (strict)"("Visible"=w606) -> ()  [unwired: 2 in, 2 out]
            n454 = property on="PWM hz" class="Str"("Visible"=w606) -> ()  [unwired: 2 in, 2 out]
            n455 = property on="PWM %" class="Str"("Visible"=w606) -> ()  [unwired: 2 in, 2 out]
            n456 = property on="SPM AEROBIC" class="Knob (strict)"("Visible"=w600) -> ()  [unwired: 2 in, 2 out]
            n457 = for {
              N: 2 -> [_]
              tunnel: [w856] -> w608
              tunnel: [w855] -> w609
              tunnel: [w852] -> w601
              n458 = flat-sequence {
                tunnel: [w859] -> w850
                tunnel: [w858] -> w849
                tunnel: [w866] -> w851
                tunnel: w850 -> [w867]
                tunnel: w849 -> [w866]
                tunnel: [w863] -> w848
                tunnel: [w862] -> w847
                tunnel: [w874] -> w854
                tunnel: [w873] -> w853
                tunnel: w851 -> [w872]
                tunnel: w848 -> [w871]
                tunnel: w847 -> [w870]
                tunnel: [w898] -> w856
                tunnel: [w894] -> w855
                tunnel: w854 -> [w894]
                tunnel: w853 -> [w893]
                tunnel: [w893] -> w852
                frame #0 {
                  n459 = local read "EQF1259 com port"() -> (w859:refnum<visa-resource-name>)
                  n460 = call "1259_usbUart.vi"("VISA resource name"=w859, "write buffer"="E\u0001", "sdFeature"=FALSE) -> ("PartNumber"=w858:string)  [unwired: 1 in, 15 out]
                  n461 = global write "Global_1259.vi" "unitType"(w858) -> ()
                  n462 = Wait (ms)(milliseconds to wait=u32 250) -> ()  [unwired: 1 out]
                }
                frame #1 {
                  n463 = call "1259_usbUart.vi"("VISA resource name"=w867, "write buffer"="v\u0002", "sdFeature"=FALSE) -> ("maxSpeed"=w862:string)  [unwired: 1 in, 15 out]
                  n464 = Fract/Exp String To Number(string=w862) -> (number=w863:dbl)  [unwired: 3 in, 1 out]
                  n465 = Wait (ms)(milliseconds to wait=u32 250) -> ()  [unwired: 1 out]
                }
                frame #2 {
                  n466 = case shown="\"1\", Default" w872 {
                    tunnel: w871 -> [w884 _]
                    tunnel: w870 -> [_ w892]
                    tunnel: [w878 w889] -> w874
                    tunnel: [w877 w888] -> w873
                    frame "1", Default {
                      # "euro"
                      n467 = local read "EQF1259 com port"() -> (w880:refnum<visa-resource-name>)
                      n468 = Multiply(x=w884, y=1.60934) -> (x*y=w882:dbl)
                      n469 = Number To Fractional String(number=w882, precision (6)=i16 1) -> (F-format string=w881:string)  [unwired: 2 in]
                      "MAX" <- w881
                      n470 = global write "Global_1259.vi" "MaxSpeed"(w881) -> ()
                      n471 = call "parseQuickKey.vi"("VISA resource name"=w880, "write buffer"="«\u0003", "y"=1, "x"=0) -> ("lengthString"=w878:i32, "KeyCodeName"=w877:string[])  [unwired: 11 in, 3 out]
                    }
                    frame "2" {
                      # "dom"
                      n472 = global write "Global_1259.vi" "MaxSpeed"(w892) -> ()
                      n473 = local write "MAX"(w892) -> ()
                      n474 = local read "EQF1259 com port"() -> (w891:refnum<visa-resource-name>)
                      n475 = call "parseQuickKey.vi"("VISA resource name"=w891, "write buffer"="©\u0002", "y"=0, "x"=0) -> ("lengthString"=w889:i32, "KeyCodeName"=w888:string[])  [unwired: 11 in, 3 out]
                    }
                  }
                  n476 = Wait (ms)(milliseconds to wait=u32 250) -> ()  [unwired: 1 out]
                }
                frame #3 {
                  n477 = global read "Global_1259.vi" "MaxSpeed"() -> (w896:string)
                  n478 = Fract/Exp String To Number(string=w896) -> (number=w895:dbl)  [unwired: 3 in, 1 out]
                  n479 = property on="SPEED" class="Knob (strict)"("Scale.Maximum"=w895) -> ()  [unwired: 2 in, 2 out]
                  n480 = call "pwm_rpmPIP.vi"() -> ("error out"=w898:errorcluster, "PWM_RPM"=→"PWM_RPM":string)  [unwired: 10 in]
                }
              }
            }
            n481 = for {
              N: 3 -> [_]
              tunnel: w608 -> [w846]
              tunnel: [w845] -> w599
              # "Speed, RPM, and SPM"
              n482 = local read "refnum out"() -> (w844:refnum<file>)
              n483 = call "dataSampled.vi"("Error In"=w846, "refnum in"=w844) -> ("error out"=w845:errorcluster)  [unwired: 8 in, 1 out]
            }
            n484 = global read "Global_1259.vi" "Inspection Point"() -> (w605:string)
            n485 = Equal?(x=w605, y="SubAssembly") -> (x = y?=w602:bool)
            n486 = case shown="False" w602 {
              tunnel: w599 -> [_ w739]
              tunnel: [w616 w738] -> w610
              tunnel: w609 -> [_ w737]
              tunnel: w601 -> [w614 w736]
              frame True {
                # "sub assembly"
                n487 = local write "PWM_RPM"("(W§c6RðS\nN\fÿYg*gÐL\fÿ÷\tcS\u0000T\u0000A\u0000R\u0000T\u0000\n\u0000(W§c6RðS\nN\fÿ\tc\tN\u000bN\u0000N*NvQ\u0000u\u0000i\u0000c\u0000k\u0000 \u0000s\u0000p\u0000e\u0000e\u0000d\u0000\bÿë_\u001f\u001f¦^\tÿ\tc®\fÿ6q\u000eTI{_Ó~gôv0R\u0007c:yopÝO\u0001c¹p®N\u00020\n\u0000(W§c6RðS\nN\fÿ\tc\u0000gNOv\u001c ë_\u001f\u001f¦^\u001d \tc®\u00020\n\u0000\n\u0000O\u0000n\u0000 \u0000t\u0000h\u0000e\u0000 \u0000c\u0000o\u0000n\u0000s\u0000o\u0000l\u0000e\u0000,\u0000 \u0000p\u0000r\u0000e\u0000s\u0000s\u0000 \u0000S\u0000T\u0000A\u0000R\u0000T\u0000 \u0000i\u0000f\u0000 \u0000n\u0000o\u0000t\u0000 \u0000r\u0000u\u0000n\u0000n\u0000i\u0000n\u0000g\u0000\n\u0000O\u0000n\u0000 \u0000t\u0000h\u0000e\u0000 \u0000c\u0000o\u0000n\u0000s\u0000o\u0000l\u0000e\u0000,\u0000 \u0000p\u0000r\u0000e\u0000s\u0000s\u0000 \u0000n\u0000e\u0000x\u0000t\u0000 \u0000Q\u0000u\u0000i\u0000c\u0000k\u0000 \u0000s\u0000p\u0000e\u0000e\u0000d\u0000 \u0000b\u0000u\u0000t\u0000t\u0000o\u0000n\u0000 \u0000o\u0000f\u0000 \u0000t\u0000h\u0000r\u0000e\u0000e\u0000 \u0000a\u0000n\u0000d\u0000 \u0000w\u0000a\u0000i\u0000t\u0000 \u0000f\u0000o\u0000r\u0000 \u0000r\u0000e\u0000s\u0000u\u0000l\u0000t\u0000s\u0000 \u0000t\u0000i\u0000l\u0000l\u0000 \u0000i\u0000n\u0000d\u0000i\u0000c\u0000a\u0000t\u0000o\u0000r\u0000 \u0000r\u0000e\u0000m\u0000a\u0000i\u0000n\u0000s\u0000 \u0000l\u0000i\u0000t\u0000.\u0000\n\u0000O\u0000n\u0000 \u0000t\u0000h\u0000e\u0000 \u0000c\u0000o\u0000n\u0000s\u0000o\u0000l\u0000e\u0000,\u0000 \u0000p\u0000r\u0000e\u0000s\u0000s\u0000 \u0000t\u0000h\u0000e\u0000 \u0000l\u0000o\u0000w\u0000e\u0000s\u0000t\u0000 \u0000Q\u0000u\u0000i\u0000c\u0000k\u0000 \u0000s\u0000p\u0000e\u0000e\u0000d\u0000 \u0000b\u0000u\u0000t\u0000t\u0000o\u0000n\u0000.\u0000") -> ()
                n488 = call-poly <userlib>:"Filter 1D Array__ogtk.vi"("items to filter"="", "array"=w614) -> ("filtered array"=w612:string[])  [unwired: 4 in, 1 out]
                n489 = flat-sequence {
                  tunnel: w612 -> [w617]
                  tunnel: [w732] -> w616
                  frame #0 {
                    n490 = while {
                      shift-right: [w621] -> _
                      shift-left: 0 -> [w622]
                      tunnel: w617 -> [w619]
                      stop <- w620 stop-if-true
                      n491 = case shown="1" w622 {
                        tunnel: [1 _] -> w621
                        tunnel: [FALSE TRUE] -> w620
                        tunnel: w619 -> [w623 _]
                        frame 0, Default {
                          n492 = while {
                            shift-right: [w628] -> _
                            shift-left: 0 -> [w629]
                            tunnel: w623 -> [w627]
                            stop <- w630 stop-if-true
                            n493 = case shown="0, Default" w629 {
                              tunnel: [FALSE FALSE TRUE] -> w630
                              tunnel: [w631 w655 2 ("f")] -> w628
                              tunnel: w627 -> [_ w654 _]
                              frame 0, Default {
                                n494 = for {
                                N: 2 -> [_]
                                tunnel: [w650] -> w649 mode=indexing
                                n495 = Random Number (0-1)() -> (number: 0 to 1=w653:dbl)
                                n496 = Multiply(x=w653, y=10.0) -> (x*y=w651:dbl)
                                n497 = To Word Integer(number=w651) -> (16bit integer=w650:i16)
                                }
                                n498 = Index Array(array=w649, index #1=0 ("index"), index #2=1 ("index")) -> (element #1=w647:i16, element #2=w648:i16)
                                n499 = Max & Min(x=w647, y=w648) -> (max(x,y)=w637:i16, min(x,y)=w643:i16)
                                "max(x,y)" <- w637
                                "min(x,y)" <- w643
                                n500 = Not Equal?(x=w637, y=w643) -> (x != y?=w641:bool)
                                n501 = Greater Or Equal?(x=i16 8 ("y"), y=w637) -> (x >= y?=w639:bool)
                                n502 = Greater Or Equal?(x=w643, y=i16 3) -> (x >= y?=w640:bool)
                                n503 = Compound Arithmetic op=AND(TRUE ("value"), w639, w641, w640) -> (w632:bool)
                                n504 = Select(t=1, s=w632, f=0) -> (s? t:f=w631:i32)
                              }
                              frame 1 {
                                n505 = for {
                                tunnel: w654 -> [w680] mode=indexing
                                tunnel: [w677] -> w667 mode=indexing
                                n506 = local read "max(x,y)"() -> (w676:i16)
                                n507 = Number To Decimal String(number=w676, width (-)=i16 0) -> (decimal integer string=w678:string)
                                n508 = Equal?(x=w680, y=w678) -> (x = y?=w677:bool)
                                }
                                n509 = for {
                                tunnel: w654 -> [w675] mode=indexing
                                tunnel: [w672] -> w664 mode=indexing
                                n510 = local read "min(x,y)"() -> (w671:i16)
                                n511 = Number To Decimal String(number=w671, width (-)=i16 0) -> (decimal integer string=w673:string)
                                n512 = Equal?(x=w675, y=w673) -> (x = y?=w672:bool)
                                }
                                n513 = call-poly <userlib>:"Filter 1D Array__ogtk.vi"("items to filter"=FALSE, "array"=w667) -> ("filtered array"=w666:bool[])  [unwired: 4 in, 1 out]
                                n514 = call-poly <userlib>:"Filter 1D Array__ogtk.vi"("items to filter"=FALSE, "array"=w664) -> ("filtered array"=w665:bool[])  [unwired: 4 in, 1 out]
                                n515 = Index Array(array=w666, index=0) -> (element=w668:bool)
                                n516 = Index Array(array=w665, index=0) -> (element=w669:bool)
                                n517 = Compound Arithmetic op=AND(TRUE ("value"), w668, w669) -> (w670:bool)
                                n518 = Select(t=2, s=w670, f=0) -> (s? t:f=w655:i32)
                              }
                              frame 2 {
                                n519 = local read "max(x,y)"() -> (w685:i16)
                                n520 = local read "min(x,y)"() -> (w684:i16)
                                n521 = Build Array(w685, w684, i16 1) -> (→"appended array":i16[])
                              }
                            }
                          }
                        }
                        frame 1 {
                          n522 = local read "appended array"() -> (w687:i16[])
                          n523 = for {
                            N: 3 -> [_]
                            tunnel: w687 -> [w692]
                            i -> [w691]
                            n524 = while {
                              tunnel: w692 -> [w708]
                              tunnel: w691 -> [w707]
                              tunnel: [w702] -> w690
                              i -> [w703]
                              stop <- w702 stop-if-true
                              n525 = Index Array(array=w708, index=w707) -> (element=w706:i16)
                              n526 = To Double Precision Float(number=w706) -> (double precision float=w705:dbl)
                              n527 = local write "Press Next"(w705) -> ()
                              n528 = Equal?(x=w703, y=1) -> (x = y?=w702:bool)
                            }
                            n529 = case shown="True" w690 {
                              frame False {
                              }
                              frame True {
                                n530 = while {
                                stop <- w698 stop-if-true
                                w701 = 0.5
                                n531 = local read "EQF1259 com port"() -> (w693:refnum<visa-resource-name>)
                                n532 = local read "Press Next"() -> (w695:dbl)
                                n533 = Add(x=w695, y=w701) -> (x+y=w700:dbl)
                                n534 = Subtract(x=w695, y=w701) -> (x-y=w699:dbl)
                                n535 = call "speedAquire.vi"("VISA resource name"=w693) -> ("SPEED"=w694:dbl)  [unwired: 6 in, 4 out]
                                n536 = local write "SPEED"(w694) -> ()
                                n537 = local read "stopP"() -> (w697:bool)
                                n538 = In Range and Coerce(upper limit=w700, x=w694, lower limit=w699) -> (In Range?=w696:bool)  [unwired: 1 out]
                                n539 = Or(x=w696, y=w697) -> (x .or. y?=w698:bool)
                                n540 = local write "Quickspeed"(w696) -> ()
                                }
                              }
                            }
                          }
                        }
                      }
                      n541 = local write "ONE\nButton"(w620) -> ()
                    }
                  }
                  frame #1 {
                    n542 = local read "refnum out"() -> (w726:refnum<file>)
                    n543 = global read "Global_1259.vi" "MaxSpeed"() -> (w725:string)
                    n544 = local read "EQF1259 com port"() -> (w721:refnum<visa-resource-name>)
                    n545 = call "dataSampled.vi"("Data"=w725, "refnum in"=w726) -> ("error out"=w722:errorcluster, "refnum out"=w727:refnum<file>)  [unwired: 8 in]
                    n546 = call "1259_usbUart.vi"("VISA resource name"=w721, "write buffer"="t\u0002", "sdFeature"=FALSE, "error in (no error)"=w722) -> ("BB FW"=w717:string, "error out"=w719:errorcluster)  [unwired: 14 out]
                    n547 = local read "Quickspeed"() -> (w724:bool)
                    n548 = call "decimalAdd.vi"("Error In"=w719, "Frequency/PWM%"=w717, "refnum in"=w727) -> ("error out"=w718:errorcluster, "concatenated string"=w723:string, "refnum out"=w720:refnum<file>)  [unwired: 6 in]
                    n549 = local write "PWM hz"(w723) -> ()
                    n550 = call "Pass_Fail.vi"("error in (no error)"=w718, "OK"=w724, "Byte Stream File in"=w720) -> ("error out"=w716:errorcluster, "Byte Stream File out"=w711:refnum<file>)  [unwired: 7 in]
                    n551 = local read "ONE\nButton"() -> (w709:bool)
                    n552 = for {
                      N: 3 -> [_]
                      tunnel: w716 -> [w731]
                      tunnel: [w730] -> w712
                      tunnel: w711 -> [w729]
                      tunnel: [w728] -> w710
                      n553 = call "dataSampled.vi"("Error In"=w731, "refnum in"=w729) -> ("error out"=w728:errorcluster, "refnum out"=w730:refnum<file>)  [unwired: 8 in]
                    }
                    n554 = call "Pass_Fail.vi"("error in (no error)"=w710, "OK"=w709, "Byte Stream File in"=w712) -> ()  [unwired: 7 in, 2 out]
                  }
                  frame #2 {
                    n555 = local read "Quickspeed"() -> (w733:bool)
                    n556 = local read "ONE\nButton"() -> (w734:bool)
                    n557 = Compound Arithmetic op=AND(w733, w734, TRUE) -> (w732:bool)
                    n558 = local write "PWM PASS"(w732) -> ()
                  }
                }
              }
              frame False {
                # "vendor assembly"
                n559 = flat-sequence {
                  tunnel: w737 -> [w741]
                  tunnel: w739 -> [_]
                  tunnel: w736 -> [w742]
                  tunnel: [w841] -> w738
                  frame #0 {
                    n560 = for {
                      N: w741 -> [_]
                      tunnel: w742 -> [w749]
                      tunnel: [w745] -> w740 mode=indexing
                      i -> [w748]
                      n561 = Index Array(array=w749, index=w748) -> (element=w743:string)
                      n562 = Empty String/Path?(string/path=w743) -> (empty?=w747:bool)
                      n563 = Not(x=w747) -> (.not. x?=w746:bool)
                      n564 = case shown="True" w746 {
                        tunnel: [FALSE TRUE] -> w744
                        tunnel: w743 -> [_ w753]
                        frame False {
                        }
                        frame True {
                          n565 = Fract/Exp String To Number(string=w753) -> (number=→"Press Next":dbl)  [unwired: 3 in, 1 out]
                          n566 = Wait (ms)(milliseconds to wait=u32 1250) -> ()  [unwired: 1 out]
                        }
                      }
                      n567 = case shown="True" w744 {
                        tunnel: [_ w755] -> w745
                        frame False {
                        }
                        frame True {
                          n568 = while {
                            tunnel: [w760] -> w755
                            stop <- w758 stop-if-true
                            w761 = 0.5 ("x")
                            n569 = local read "EQF1259 com port"() -> (w762:refnum<visa-resource-name>)
                            n570 = local read "Press Next"() -> (w759:dbl)
                            n571 = Add(x=w761, y=w759) -> (x+y=w764:dbl)
                            n572 = Subtract(x=w759, y=w761) -> (x-y=w763:dbl)
                            n573 = call "speedAquire.vi"("VISA resource name"=w762) -> ("SPEED"=w760:dbl)  [unwired: 6 in, 4 out]
                            "SPEED" <- w760
                            n574 = In Range and Coerce(upper limit=w764, x=w760, lower limit=w763) -> (In Range?=w756:bool)  [unwired: 1 out]
                            "Quickspeed" <- w756
                            n575 = Or(x=w756, y="stopP") -> (x .or. y?=w758:bool)
                          }
                        }
                      }
                    }
                    "speedArray" <- w740
                  }
                  frame #1 {
                    n576 = flat-sequence {
                      tunnel: [w774] -> w769
                      tunnel: [w775] -> w768
                      tunnel: [w773] -> w765
                      tunnel: [w787] -> w770
                      tunnel: w769 -> [w787]
                      tunnel: w768 -> [w786]
                      tunnel: [w786] -> w767
                      tunnel: [w785] -> w766
                      tunnel: w765 -> [w785]
                      tunnel: w770 -> [w792]
                      tunnel: w767 -> [w791]
                      tunnel: w766 -> [w790]
                      frame #0 {
                        n577 = local read "EQF1259 com port"() -> (w773:refnum<visa-resource-name>)
                        n578 = local read "refnum out"() -> (w780:refnum<file>)
                        n579 = global read "Global_1259.vi" "MaxSpeed"() -> (w779:string)
                        n580 = call "dataSampled.vi"("Data"=w779, "refnum in"=w780) -> ("error out"=w778:errorcluster)  [unwired: 8 in, 1 out]
                        n581 = call "1259_usbUart.vi"("VISA resource name"=w773, "write buffer"="t\u0002", "sdFeature"=FALSE, "error in (no error)"=w778) -> ("BB FW"=w783:string, "error out"=w777:errorcluster)  [unwired: 14 out]
                        n582 = call "decimalAdd.vi"("Error In"=w777, "Frequency/PWM%"=w783, "refnum in"=w780) -> ("error out"=w782:errorcluster, "concatenated string"=→"PWM hz":string, "refnum out"=w776:refnum<file>)  [unwired: 6 in]
                        n583 = local read "Quickspeed"() -> (w772:bool)
                        n584 = call "Pass_Fail.vi"("error in (no error)"=w782, "OK"=w772, "Byte Stream File in"=w776) -> ("error out"=w775:errorcluster, "Byte Stream File out"=w774:refnum<file>)  [unwired: 7 in]
                      }
                      frame #1 {
                        n585 = Wait (ms)(milliseconds to wait=u32 1000) -> ()  [unwired: 1 out]
                      }
                      frame #2 {
                        n586 = call "1259_usbUart.vi"("VISA resource name"=w790, "write buffer"="r\u0002", "sdFeature"=FALSE, "error in (no error)"=w791) -> ("BB FW"=w794:string, "error out"=w796:errorcluster)  [unwired: 14 out]
                        n587 = call "decimalAdd.vi"("Error In"=w796, "Frequency/PWM%"=w794, "refnum in"=w792) -> ("concatenated string"=→"PWM %":string)  [unwired: 6 in, 2 out]
                      }
                    }
                  }
                  frame #2 {
                    n588 = local read "EQF1259 com port"() -> (w797:refnum<visa-resource-name>)
                    n589 = while {
                      tunnel: [w804] -> w798
                      tunnel: w797 -> [w800]
                      stop <- w805 stop-if-true
                      n590 = global read "Global_1259.vi" "MaxSpeed"() -> (w809:string)
                      n591 = call "speedAquire.vi"("VISA resource name"=w800) -> ("KPH/MPH"=w811:string)  [unwired: 6 in, 4 out]
                      n592 = Fract/Exp String To Number(string=w809) -> (number=w808:dbl)  [unwired: 3 in, 1 out]
                      n593 = Fract/Exp String To Number(string=w811) -> (number=w810:dbl)  [unwired: 3 in, 1 out]
                      n594 = Subtract(x=w808, y=1.0) -> (x-y=w806:dbl)
                      n595 = local write "SPEED"(w810) -> ()
                      n596 = local read "stopP"() -> (w801:bool)
                      n597 = Less?(x=w810, y=w806) -> (x < y?=w803:bool)
                      n598 = Or(x=w801, y=w803) -> (x .or. y?=w805:bool)
                      n599 = Not(x=w801) -> (.not. x?=w802:bool)
                      n600 = And(x=w803, y=w802) -> (x .and. y?=w804:bool)
                    }
                    "Minus\nButton" <- w798
                    n601 = local read "refnum out"() -> (w799:refnum<file>)
                    n602 = call "Pass_Fail.vi"("OK"=w798, "Byte Stream File in"=w799) -> ()  [unwired: 8 in, 2 out]
                  }
                  frame #3 {
                    n603 = local read "EQF1259 com port"() -> (w812:refnum<visa-resource-name>)
                    n604 = while {
                      tunnel: [w818] -> w813
                      tunnel: w812 -> [w815]
                      stop <- w819 stop-if-true
                      n605 = global read "Global_1259.vi" "MaxSpeed"() -> (w824:string)
                      n606 = call "speedAquire.vi"("VISA resource name"=w815) -> ("KPH/MPH"=w826:string)  [unwired: 6 in, 4 out]
                      n607 = Fract/Exp String To Number(string=w824) -> (number=w822:dbl)  [unwired: 3 in, 1 out]
                      n608 = Fract/Exp String To Number(string=w826) -> (number=w825:dbl)  [unwired: 3 in, 1 out]
                      n609 = Subtract(x=w822, y=0.5) -> (x-y=w823:dbl)
                      n610 = local write "SPEED"(w825) -> ()
                      n611 = local read "stopP"() -> (w817:bool)
                      n612 = Greater?(x=w825, y=w823) -> (0:w816:bool)
                      n613 = Or(x=w816, y=w817) -> (x .or. y?=w819:bool)
                      n614 = Not(x=w817) -> (.not. x?=w820:bool)
                      n615 = And(x=w816, y=w820) -> (x .and. y?=w818:bool)
                    }
                    "Plus\nButton" <- w813
                    n616 = local read "refnum out"() -> (w814:refnum<file>)
                    n617 = call "Pass_Fail.vi"("OK"=w813, "Byte Stream File in"=w814) -> ()  [unwired: 8 in, 2 out]
                  }
                  frame #4 {
                    n618 = local read "EQF1259 com port"() -> (w827:refnum<visa-resource-name>)
                    n619 = while {
                      tunnel: [w831] -> w828
                      tunnel: w827 -> [w837]
                      stop <- w832 stop-if-true
                      n620 = call "speedAquire.vi"("VISA resource name"=w837) -> ("KPH/MPH"=w838:string)  [unwired: 6 in, 4 out]
                      n621 = Fract/Exp String To Number(string=w838) -> (number=w835:dbl)  [unwired: 3 in, 1 out]
                      n622 = local write "SPEED"(w835) -> ()
                      n623 = local read "stopP"() -> (w834:bool)
                      n624 = Less?(x=w835, y=2.0) -> (x < y?=w830:bool)
                      n625 = Not(x=w834) -> (.not. x?=w833:bool)
                      n626 = Or(x=w834, y=w830) -> (x .or. y?=w832:bool)
                      n627 = And(x=w830, y=w833) -> (x .and. y?=w831:bool)
                    }
                    "ONE\nButton" <- w828
                    n628 = local read "refnum out"() -> (w829:refnum<file>)
                    n629 = call "Pass_Fail.vi"("OK"=w828, "Byte Stream File in"=w829) -> ()  [unwired: 8 in, 2 out]
                  }
                  frame #5 {
                    n630 = local read "Minus\nButton"() -> (w842:bool)
                    n631 = local read "ONE\nButton"() -> (w839:bool)
                    n632 = local read "Plus\nButton"() -> (w843:bool)
                    n633 = Compound Arithmetic op=AND(w842, w843, w839, TRUE ("value")) -> (w841:bool)
                    "PWM PASS" <- w841
                  }
                }
              }
            }
          }
        }
        n634 = Select(t=T3."Pulse" ("Tab Control"), s=w528, f=T3."Failed" ("Tab Control")) -> (s? t:f=w534:T3)
      }
      frame "Incline" {
        w904 = FALSE ("Visible")
        n635 = local write "negative incline"(0.0 ("negative incline")) -> ()
        n636 = local write "Up"(w904) -> ()
        n637 = local write "Down"(w904) -> ()
        n638 = local write "ZERO"(w904) -> ()
        n639 = local write "stopI"(w904) -> ()
        n640 = local write "inclineArray"(dbl[] []) -> ()
        n641 = property on="incline" class="WFChart (strict)"("History Data"=dbl[] []) -> ()  [unwired: 2 in, 2 out]
        n642 = local write "INCLINE PASS"(w904) -> ()
        n643 = local write "Quickincline"(w904) -> ()
        n644 = global read "Global_1259.vi" "gradeType"() -> (w910:string)
        n645 = Equal?(x=w910, y="0") -> (x = y?=w902:bool)
        n646 = case shown="False" w902 {
          tunnel: [FALSE w1338] -> w903
          frame True {
          }
          frame False {
            n647 = global read "Global_1259.vi" "gradeType"() -> (w1341:string)
            n648 = Decimal String To Number(string=w1341) -> (number=w1340:i32)  [unwired: 2 in, 1 out]
            n649 = Greater Or Equal?(x=w1340, y=2) -> (x >= y?=w1338:bool)
          }
        }
        n650 = global read "Global_1259.vi" "Inspection Point"() -> (w900:string)
        n651 = Equal?(x=w900, y="SubAssembly") -> (x = y?=w899:bool)
        n652 = case shown="False" w899 {
          tunnel: [w918 w1066] -> w915
          tunnel: [FALSE w1065] -> w914
          tunnel: w903 -> [w917 w1064]
          frame True {
            # "Quick"
            n653 = case shown="True" w917 {
              tunnel: [TRUE w939] -> w918
              frame False {
                n654 = local read "refnum out"() -> (w931:refnum<file>)
                n655 = call "dataSampled.vi"("refnum in"=w931) -> ("error out"=w925:errorcluster, "refnum out"=w930:refnum<file>)  [unwired: 9 in]
                n656 = call "dataSampled.vi"("Error In"=w925, "refnum in"=w930) -> ("error out"=w924:errorcluster, "refnum out"=w929:refnum<file>)  [unwired: 8 in]
                n657 = call "dataSampled.vi"("Error In"=w924, "refnum in"=w929) -> ("error out"=w923:errorcluster, "refnum out"=w928:refnum<file>)  [unwired: 8 in]
                n658 = call "dataSampled.vi"("Error In"=w923, "refnum in"=w928) -> ("error out"=w922:errorcluster, "refnum out"=w927:refnum<file>)  [unwired: 8 in]
                n659 = call "dataSampled.vi"("Error In"=w922, "refnum in"=w927) -> ("error out"=w921:errorcluster, "refnum out"=w926:refnum<file>)  [unwired: 8 in]
                n660 = call "dataSampled.vi"("Error In"=w921, "refnum in"=w926) -> ()  [unwired: 8 in, 2 out]
              }
              frame True {
                n661 = local write "INCLINE-14"("(W§c6RðS\nN\fÿ\tc\u000bN\u0000N*N\u001c ë_\u001f>Pe\u001d \tc®\fÿ6q\u000eTI{_Ó~gôv0R\u0007c:yopÝO\u0001c¹p®N\u00020\n\u0000(W§c6RðS\nN\fÿ\tc\u0000gNOv\u001c ë_\u001f>Pe\u001d \tc®\u00020\n\u0000\n\u0000O\u0000n\u0000 \u0000t\u0000h\u0000e\u0000 \u0000c\u0000o\u0000n\u0000s\u0000o\u0000l\u0000e\u0000,\u0000 \u0000p\u0000r\u0000e\u0000s\u0000s\u0000 \u0000n\u0000e\u0000x\u0000t\u0000 \u0000Q\u0000u\u0000i\u0000c\u0000k\u0000 \u0000i\u0000n\u0000c\u0000l\u0000i\u0000n\u0000e\u0000 \u0000b\u0000u\u0000t\u0000t\u0000o\u0000n\u0000 \u0000a\u0000n\u0000d\u0000 \u0000w\u0000a\u0000i\u0000t\u0000 \u0000f\u0000o\u0000r\u0000 \u0000r\u0000e\u0000s\u0000u\u0000l\u0000t\u0000s\u0000 \u0000t\u0000i\u0000l\u0000l\u0000 \u0000i\u0000n\u0000d\u0000i\u0000c\u0000a\u0000t\u0000o\u0000r\u0000 \u0000r\u0000e\u0000m\u0000a\u0000i\u0000n\u0000s\u0000 \u0000l\u0000i\u0000t\u0000.\u0000\n\u0000O\u0000n\u0000 \u0000t\u0000h\u0000e\u0000 \u0000c\u0000o\u0000n\u0000s\u0000o\u0000l\u0000e\u0000,\u0000 \u0000p\u0000r\u0000e\u0000s\u0000s\u0000 \u0000t\u0000h\u0000e\u0000 \u0000l\u0000o\u0000w\u0000e\u0000s\u0000t\u0000 \u0000Q\u0000u\u0000i\u0000c\u0000k\u0000 \u0000i\u0000n\u0000c\u0000l\u0000i\u0000n\u0000e\u0000 \u0000b\u0000u\u0000t\u0000t\u0000o\u0000n\u0000.\u0000\u0000\u0000o\u0000n\u0000.\u0000") -> ()
                n662 = local read "EQF1259 com port"() -> (w938:refnum<visa-resource-name>)
                n663 = call "parseQuickKey.vi"("VISA resource name"=w938, "write buffer"="®\b", "y"=2, "x"=0) -> ("KeyCodeName"=w934:string[])  [unwired: 11 in, 4 out]
                n664 = call-poly <userlib>:"Filter 1D Array__ogtk.vi"("items to filter"="", "array"=w934) -> ("filtered array"=w932:string[])  [unwired: 4 in, 1 out]
                n665 = flat-sequence {
                  tunnel: w932 -> [w941]
                  tunnel: [w1060] -> w939
                  frame #0 {
                    n666 = while {
                      shift-right: [w945] -> _
                      shift-left: 0 -> [w946]
                      tunnel: w941 -> [w944]
                      stop <- w943 stop-if-true
                      n667 = case shown="1" w946 {
                        tunnel: [1 _] -> w945
                        tunnel: [FALSE TRUE] -> w943
                        tunnel: w944 -> [w947 _]
                        frame 0, Default {
                          n668 = while {
                            shift-right: [w953] -> _
                            shift-left: 0 -> [w954]
                            tunnel: w947 -> [w951]
                            stop <- w952 stop-if-true
                            n669 = case shown="0, Default" w954 {
                              tunnel: [w959 w980 2] -> w953
                              tunnel: [FALSE FALSE TRUE] -> w952
                              tunnel: w951 -> [_ w978 _]
                              frame 0, Default {
                                n670 = for {
                                N: 2 -> [_]
                                tunnel: [w974] -> w973 mode=indexing
                                n671 = Random Number (0-1)() -> (number: 0 to 1=w977:dbl)
                                n672 = Multiply(x=w977, y=10.0) -> (x*y=w975:dbl)
                                n673 = To Word Integer(number=w975) -> (16bit integer=w974:i16)
                                }
                                n674 = Index Array(array=w973, index #1=0 ("index"), index #2=1 ("index")) -> (element #1=w971:i16, element #2=w972:i16)
                                n675 = Max & Min(x=w971, y=w972) -> (max(x,y)=w960:i16, min(x,y)=w961:i16)
                                n676 = local write "max(x,y)"(w960) -> ()
                                n677 = local write "min(x,y)"(w961) -> ()
                                n678 = Not Equal?(x=w960, y=w961) -> (x != y?=w966:bool)
                                n679 = Greater Or Equal?(x=i16 8 ("y"), y=w960) -> (x >= y?=w964:bool)
                                n680 = Greater Or Equal?(x=w961, y=i16 3) -> (x >= y?=w965:bool)
                                n681 = Compound Arithmetic op=AND(TRUE ("value"), w964, w966, w965) -> (w956:bool)
                                n682 = Select(t=1, s=w956, f=0) -> (s? t:f=w959:i32)
                              }
                              frame 1 {
                                n683 = for {
                                tunnel: w978 -> [w1004] mode=indexing
                                tunnel: [w1001] -> w991 mode=indexing
                                n684 = local read "max(x,y)"() -> (w1000:i16)
                                n685 = Number To Decimal String(number=w1000, width (-)=i16 0) -> (decimal integer string=w1002:string)
                                n686 = Equal?(x=w1004, y=w1002) -> (x = y?=w1001:bool)
                                }
                                n687 = for {
                                tunnel: w978 -> [w999] mode=indexing
                                tunnel: [w996] -> w988 mode=indexing
                                n688 = local read "min(x,y)"() -> (w995:i16)
                                n689 = Number To Decimal String(number=w995, width (-)=i16 0) -> (decimal integer string=w997:string)
                                n690 = Equal?(x=w999, y=w997) -> (x = y?=w996:bool)
                                }
                                n691 = call-poly <userlib>:"Filter 1D Array__ogtk.vi"("items to filter"=FALSE, "array"=w991) -> ("filtered array"=w990:bool[])  [unwired: 4 in, 1 out]
                                n692 = call-poly <userlib>:"Filter 1D Array__ogtk.vi"("items to filter"=FALSE, "array"=w988) -> ("filtered array"=w989:bool[])  [unwired: 4 in, 1 out]
                                n693 = Index Array(array=w990, index=0) -> (element=w992:bool)
                                n694 = Index Array(array=w989, index=0) -> (element=w993:bool)
                                n695 = Compound Arithmetic op=AND(TRUE ("value"), w992, w993) -> (w994:bool)
                                n696 = Select(t=2, s=w994, f=0) -> (s? t:f=w980:i32)
                              }
                              frame 2 {
                                n697 = local read "max(x,y)"() -> (w1010:i16)
                                n698 = local read "min(x,y)"() -> (w1009:i16)
                                n699 = Build Array(w1010, w1009, i16 0) -> (w1008:i16[])
                                n700 = local write "appended array"(w1008) -> ()
                              }
                            }
                          }
                        }
                        frame 1 {
                          n701 = local read "appended array"() -> (w1013:i16[])
                          n702 = for {
                            N: 3 -> [_]
                            tunnel: w1013 -> [w1016]
                            i -> [w1015]
                            n703 = while {
                              tunnel: w1016 -> [w1033]
                              tunnel: w1015 -> [w1031]
                              tunnel: [w1028] -> w1014
                              i -> [w1030]
                              stop <- w1028 stop-if-true
                              n704 = Index Array(array=w1033, index=w1031) -> (element=w1032:i16)
                              n705 = To Double Precision Float(number=w1032) -> (double precision float=w1027:dbl)
                              n706 = local write "Press Next"(w1027) -> ()
                              n707 = Equal?(x=w1030, y=1) -> (x = y?=w1028:bool)
                            }
                            n708 = case shown="True" w1014 {
                              frame False {
                              }
                              frame True {
                                n709 = while {
                                stop <- w1022 stop-if-true
                                w1026 = 0.3
                                n710 = local read "EQF1259 com port"() -> (w1019:refnum<visa-resource-name>)
                                n711 = local read "Press Next"() -> (w1021:dbl)
                                n712 = Add(x=w1021, y=w1026) -> (x+y=w1025:dbl)
                                n713 = Subtract(x=w1021, y=w1026) -> (x-y=w1024:dbl)
                                n714 = call "inclineAquire.vi"("Negative Incline"=0.0, "VISA Refnum in"=w1019) -> ("Incline Out"=w1020:dbl)  [unwired: 8 in, 1 out]
                                n715 = local write "incline"(w1020) -> ()
                                n716 = local read "stopI"() -> (w1023:bool)
                                n717 = In Range and Coerce(upper limit=w1025, x=w1020, lower limit=w1024) -> (In Range?=w1017:bool)  [unwired: 1 out]
                                n718 = Or(x=w1017, y=w1023) -> (x .or. y?=w1022:bool)
                                n719 = local write "Quickincline"(w1017) -> ()
                                }
                              }
                            }
                          }
                        }
                      }
                      n720 = local write "ZERO"(w943) -> ()
                    }
                  }
                  frame #1 {
                    n721 = for {
                      N: 2 -> [_]
                      tunnel: [w1058] -> w1041
                      tunnel: [w1057] -> w1038
                      n722 = local read "refnum out"() -> (w1059:refnum<file>)
                      n723 = call "dataSampled.vi"("refnum in"=w1059) -> ("error out"=w1058:errorcluster, "refnum out"=w1057:refnum<file>)  [unwired: 9 in]
                    }
                    n724 = case shown="True" TRUE {
                      tunnel: w1041 -> [w1051 w1055]
                      tunnel: [w1050 w1054] -> w1040
                      tunnel: [w1049 w1053] -> w1037
                      tunnel: w1038 -> [w1048 w1052]
                      frame False {
                        n725 = call "dataSampled.vi"("Error In"=w1051, "refnum in"=w1048) -> ("error out"=w1050:errorcluster, "refnum out"=w1049:refnum<file>)  [unwired: 8 in]
                      }
                      frame True {
                        n726 = local read "Quickincline"() -> (w1056:bool)
                        n727 = call "Pass_Fail.vi"("error in (no error)"=w1055, "OK"=w1056, "Byte Stream File in"=w1052) -> ("error out"=w1054:errorcluster, "Byte Stream File out"=w1053:refnum<file>)  [unwired: 7 in]
                      }
                    }
                    n728 = for {
                      N: 2 -> [_]
                      tunnel: [w1047] -> w1034
                      tunnel: w1040 -> [w1046]
                      tunnel: w1037 -> [w1045]
                      tunnel: [w1044] -> w1036
                      n729 = call "dataSampled.vi"("Error In"=w1046, "refnum in"=w1045) -> ("error out"=w1047:errorcluster, "refnum out"=w1044:refnum<file>)  [unwired: 8 in]
                    }
                    n730 = local read "ZERO"() -> (w1035:bool)
                    n731 = call "Pass_Fail.vi"("error in (no error)"=w1034, "OK"=w1035, "Byte Stream File in"=w1036) -> ()  [unwired: 7 in, 2 out]
                  }
                  frame #2 {
                    n732 = local read "Quickincline"() -> (w1062:bool)
                    n733 = local read "ZERO"() -> (w1061:bool)
                    n734 = Compound Arithmetic op=AND(TRUE, w1062, w1061) -> (w1060:bool)
                    n735 = local write "INCLINE PASS"(w1060) -> ()
                  }
                }
              }
            }
          }
          frame False {
            # "Standard"
            n736 = case shown="True" w1064 {
              tunnel: [TRUE w1093] -> w1066
              tunnel: [FALSE ("E-Stop/Incline") FALSE ("E-Stop/Incline")] -> w1065
              frame False {
                n737 = local read "refnum out"() -> (w1078:refnum<file>)
                n738 = call "dataSampled.vi"("refnum in"=w1078) -> ("error out"=w1074:errorcluster, "refnum out"=w1077:refnum<file>)  [unwired: 9 in]
                n739 = call "dataSampled.vi"("Error In"=w1074, "refnum in"=w1077) -> ("error out"=w1073:errorcluster, "refnum out"=w1076:refnum<file>)  [unwired: 8 in]
                n740 = call "dataSampled.vi"("Error In"=w1073, "refnum in"=w1076) -> ("error out"=w1072:errorcluster, "refnum out"=w1067:refnum<file>)  [unwired: 8 in]
                n741 = call "dataSampled.vi"("Error In"=w1072, "refnum in"=w1067) -> ("error out"=w1071:errorcluster, "refnum out"=w1068:refnum<file>)  [unwired: 8 in]
                n742 = call "dataSampled.vi"("Error In"=w1071, "refnum in"=w1068) -> ("error out"=w1070:errorcluster, "refnum out"=w1069:refnum<file>)  [unwired: 8 in]
                n743 = call "dataSampled.vi"("Error In"=w1070, "refnum in"=w1069) -> ()  [unwired: 8 in, 2 out]
              }
              frame True {
                n744 = flat-sequence {
                  tunnel: [w1101] -> w1082
                  tunnel: [w1098] -> w1081
                  tunnel: [w1100] -> w1080
                  tunnel: [w1104] -> w1091
                  tunnel: [w1113] -> w1086
                  tunnel: w1082 -> [w1106]
                  tunnel: w1081 -> [w1104]
                  tunnel: w1080 -> [w1105]
                  tunnel: [w1128] -> w1096
                  tunnel: [w1129] -> w1095
                  tunnel: [w1127] -> w1092
                  tunnel: w1091 -> [w1126]
                  tunnel: w1086 -> [w1124]
                  tunnel: [w1122] -> w1085
                  tunnel: [w1121] -> w1084
                  tunnel: w1096 -> [w1147]
                  tunnel: w1095 -> [w1149]
                  tunnel: w1092 -> [w1148]
                  tunnel: [w1133] -> w1090
                  tunnel: w1085 -> [w1146]
                  tunnel: w1084 -> [w1143]
                  tunnel: w1090 -> [w1244]
                  tunnel: [w1244] -> w1089
                  tunnel: w1089 -> [w1259]
                  tunnel: [w1259] -> w1088
                  tunnel: w1088 -> [w1284]
                  tunnel: [w1284] -> w1087
                  tunnel: w1087 -> [w1309]
                  tunnel: [w1309] -> w1083
                  tunnel: [w1326] -> w1093
                  tunnel: w1083 -> [w1325]
                  frame #0 {
                    w1101 = FALSE ("sdFeature")
                    n745 = global read "Global_1259.vi" "EQF1259 com port"() -> (w1097:refnum<visa-resource-name>)
                    n746 = Wait (ms)(milliseconds to wait=u32 250) -> ()  [unwired: 1 out]
                    n747 = call "1259_usbUart.vi"("VISA resource name"=w1097, "write buffer"="€\u0002", "sdFeature"=w1101) -> ("double precision float"=w1098:dbl, "error out"=w1100:errorcluster)  [unwired: 1 in, 14 out]
                  }
                  frame #1 {
                    n748 = global read "Global_1259.vi" "EQF1259 com port"() -> (w1103:refnum<visa-resource-name>)
                    n749 = Wait (ms)(milliseconds to wait=u32 250) -> ()  [unwired: 1 out]
                    n750 = call "1259_usbUart.vi"("VISA resource name"=w1103, "write buffer"="‚\u0002", "sdFeature"=w1106, "error in (no error)"=w1105) -> ("number[0]"=w1108:u32, "negative incline"=w1107:dbl, "error out"=w1113:errorcluster)  [unwired: 13 out]
                    n751 = Equal?(x=w1108, y=u32 0) -> (x = y?=w1109:bool)
                    n752 = case shown="False" w1109 {
                      tunnel: w1108 -> [_ w1116]
                      tunnel: w1107 -> [w1114 _]
                      frame False {
                        "negative incline" <- w1114
                      }
                      frame True {
                        n753 = To Double Precision Float(number=w1116) -> (double precision float=w1115:dbl)
                        n754 = local write "negative incline"(w1115) -> ()
                      }
                    }
                  }
                  frame #2 {
                    n755 = global read "Global_1259.vi" "EQF1259 com port"() -> (w1117:refnum<visa-resource-name>)
                    n756 = Wait (ms)(milliseconds to wait=u32 250) -> ()  [unwired: 1 out]
                    n757 = local read "negative incline"() -> (w1119:dbl)
                    n758 = local write "Press Next"(w1119) -> ()
                    n759 = call "1259_usbUart.vi"("VISA resource name"=w1117, "write buffer"="Å\u0002", "sdFeature"=FALSE, "error in (no error)"=w1124) -> ("double precision float"=w1122:dbl, "error out"=w1125:errorcluster)  [unwired: 14 out]
                    n760 = call "inclineCount.vi"("error in (no error)"=w1125, "negative incline"=w1119, "max incline"=w1126) -> ("error out"=w1121:errorcluster, "press start"=w1128:dbl, "max incline"=w1127:dbl)  [unwired: 5 in, 1 out]
                    n761 = Not Equal?(x=w1119, y=0.0) -> (x != y?=w1129:bool)
                  }
                  frame #3 {
                    # "Note: changed incline compare from .6 to .1 on negative and from .5 to .1 on positive to eliminate false presses at the low end. need more data. 06-04-20"
                    n762 = global read "Global_1259.vi" "EQF1259 com port"() -> (w1131:refnum<visa-resource-name>)
                    n763 = Increment(x=w1148) -> (x+1=w1137:dbl)
                    n764 = Decrement(x=w1147) -> (x-1=w1136:dbl)
                    n765 = call "parseQuickKey.vi"("VISA resource name"=w1131, "write buffer"="®\b", "y"=2, "x"=0, "error in (no error)"=w1143) -> ("lengthString"=w1138:i32, "KeyCodeName"=w1150:string[], "No Keys"=w1133:bool, "error out"=w1144:errorcluster)  [unwired: 10 in, 1 out]
                    n766 = property on="incline" class="WFChart (strict)"("YScale.Maximum"=w1137) -> ()  [unwired: 2 in, 2 out]
                    n767 = property on="incline" class="WFChart (strict)"("YScale.Minimum"=w1136) -> ()  [unwired: 2 in, 2 out]
                    n768 = Decrement(x=w1138) -> (x-1=w1142:i32)
                    n769 = call "delayTransmax.vi"("error in (no error)"=w1144, "Tmax"=w1146, "Bcount"=w1142) -> ("error out"=w1134:errorcluster, "Tdelay"=w1145:dbl)  [unwired: 7 in]
                    n770 = case shown="True" w1149 {
                      tunnel: w1142 -> [w1154 w1197]
                      tunnel: w1131 -> [w1156 w1199]
                      tunnel: w1150 -> [w1155 w1198]
                      tunnel: w1145 -> [w1153 w1196]
                      tunnel: w1133 -> [w1151 w1194]
                      frame False {
                        n771 = for {
                          N: w1154 -> [_]
                          tunnel: w1156 -> [w1169]
                          tunnel: w1155 -> [w1167]
                          tunnel: w1153 -> [w1158]
                          tunnel: [w1159] -> w1152 mode=indexing
                          tunnel: w1151 -> [w1157]
                          i -> [w1168]
                          n772 = Index Array(array=w1167, index=w1168) -> (element=w1161:string)
                          n773 = Empty String/Path?(string/path=w1161) -> (empty?=w1163:bool)
                          n774 = Equal?(x=w1161, y="0") -> (x = y?=w1162:bool)
                          n775 = Or(x=w1162, y=w1163) -> (x .or. y?=w1164:bool)
                          n776 = Not(x=w1164) -> (.not. x?=w1166:bool)
                          n777 = case shown="True" w1166 {
                            tunnel: [w1172 TRUE] -> w1160
                            tunnel: w1161 -> [_ w1180]
                            tunnel: w1158 -> [_ w1176]
                            frame False {
                              n778 = local read "Press Next"() -> (w1171:dbl)
                              n779 = local read "MAX"() -> (w1170:dbl)
                              n780 = Equal?(x=w1171, y=w1170) -> (x = y?=w1175:bool)
                              n781 = Select(t=TRUE, s=w1175, f=FALSE) -> (s? t:f=w1172:bool)
                            }
                            frame True {
                              n782 = To Unsigned Long Integer(number=w1176) -> (unsigned 32bit integer=w1177:u32)
                              n783 = Fract/Exp String To Number(string=w1180) -> (number=w1179:dbl)  [unwired: 3 in, 1 out]
                              n784 = Wait (ms)(milliseconds to wait=w1177) -> ()  [unwired: 1 out]
                              n785 = local write "Press Next"(w1179) -> ()
                            }
                          }
                          n786 = case shown="True" w1160 {
                            tunnel: w1169 -> [_ w1183]
                            tunnel: [_ w1182] -> w1159
                            tunnel: w1157 -> [w1181 _]
                            frame False {
                              n787 = local write "Quickincline"(w1181) -> ()
                            }
                            frame True {
                              n788 = while {
                                tunnel: w1183 -> [w1192]
                                tunnel: [w1187] -> w1182
                                stop <- w1186 stop-if-true
                                w1189 = 0.5 ("y")
                                n789 = local read "negative incline"() -> (w1193:dbl)
                                n790 = local read "Press Next"() -> (w1188:dbl)
                                n791 = Add(x=w1188, y=w1189) -> (x+y=w1190:dbl)
                                n792 = Subtract(x=w1188, y=w1189) -> (x-y=w1191:dbl)
                                n793 = call "inclineAquire.vi"("Negative Incline"=w1193, "VISA Refnum in"=w1192) -> ("Incline Out"=w1187:dbl)  [unwired: 8 in, 1 out]
                                n794 = local write "incline"(w1187) -> ()
                                n795 = In Range and Coerce(upper limit=w1190, x=w1187, lower limit=w1191) -> (In Range?=w1184:bool)  [unwired: 1 out]
                                n796 = Or(x=w1184, y="stopI") -> (x .or. y?=w1186:bool)
                                n797 = local write "Quickincline"(w1184) -> ()
                              }
                            }
                          }
                        }
                        n798 = local write "inclineArray"(w1152) -> ()
                      }
                      frame True {
                        n799 = for {
                          N: w1197 -> [_]
                          tunnel: w1199 -> [_]
                          tunnel: w1198 -> [w1210]
                          tunnel: w1196 -> [w1201]
                          tunnel: [w1209] -> w1195 mode=indexing
                          tunnel: w1194 -> [w1200]
                          i -> [w1211]
                          n800 = Index Array(array=w1210, index=w1211) -> (element=w1205:string)
                          n801 = Empty String/Path?(string/path=w1205) -> (empty?=w1207:bool)
                          n802 = Equal?(x=w1205, y="0") -> (x = y?=w1206:bool)
                          n803 = Or(x=w1206, y=w1207) -> (x .or. y?=w1208:bool)
                          n804 = Not(x=w1208) -> (.not. x?=w1202:bool)
                          n805 = case shown="True" w1202 {
                            tunnel: w1205 -> [_ w1222]
                            tunnel: [w1212 TRUE] -> w1203
                            tunnel: w1201 -> [_ w1218]
                            frame False {
                              n806 = local read "Press Next"() -> (w1217:dbl)
                              n807 = local read "MAX"() -> (w1216:dbl)
                              n808 = Equal?(x=w1217, y=w1216) -> (x = y?=w1215:bool)
                              n809 = Select(t=TRUE, s=w1215, f=FALSE) -> (s? t:f=w1212:bool)
                            }
                            frame True {
                              n810 = To Unsigned Long Integer(number=w1218) -> (unsigned 32bit integer=w1219:u32)
                              n811 = Fract/Exp String To Number(string=w1222) -> (number=→"Press Next":dbl)  [unwired: 3 in, 1 out]
                              n812 = Wait (ms)(milliseconds to wait=w1219) -> ()  [unwired: 1 out]
                            }
                          }
                          n813 = case shown="True" w1203 {
                            tunnel: [_ w1224] -> w1209
                            tunnel: w1200 -> [w1223 _]
                            frame False {
                              n814 = local write "Quickincline"(w1223) -> ()
                            }
                            frame True {
                              n815 = while {
                                tunnel: [w1226] -> w1224
                                stop <- w1231 stop-if-true
                                n816 = global read "Global_1259.vi" "EQF1259 com port"() -> (w1225:refnum<visa-resource-name>)
                                n817 = local read "negative incline"() -> (w1233:dbl)
                                n818 = call "inclineAquire.vi"("Negative Incline"=w1233, "VISA Refnum in"=w1225) -> ("Incline Out"=w1226:dbl)  [unwired: 8 in, 1 out]
                                "incline" <- w1226
                                n819 = local read "Press Next"() -> (w1232:dbl)
                                n820 = Greater Or Equal?(x=w1226, y=0.0) -> (x >= y?=w1235:bool)
                                n821 = case shown="False" w1235 {
                                tunnel: w1232 -> [w1238 w1243]
                                tunnel: [w1237 w1241] -> w1228
                                tunnel: [w1236 w1240] -> w1227
                                frame False {
                                w1239 = 0.5 ("x")
                                # "Positive"
                                n822 = Subtract(x=w1238, y=w1239) -> (x-y=w1237:dbl)
                                n823 = Add(x=w1239, y=w1238) -> (x+y=w1236:dbl)
                                }
                                frame True {
                                w1242 = 0.6
                                # "negative"
                                n824 = Subtract(x=w1243, y=w1242) -> (x-y=w1241:dbl)
                                n825 = Add(x=w1242, y=w1243) -> (x+y=w1240:dbl)
                                }
                                }
                                n826 = local read "stopI"() -> (w1230:bool)
                                n827 = In Range and Coerce(upper limit=w1227, x=w1226, lower limit=w1228) -> (In Range?=w1229:bool)  [unwired: 1 out]
                                "Quickincline" <- w1229
                                n828 = Or(x=w1229, y=w1230) -> (x .or. y?=w1231:bool)
                              }
                            }
                          }
                        }
                        "inclineArray" <- w1195
                      }
                    }
                    n829 = call "inclinePIP.vi"("error in (no error)"=w1134, "QUICK_KEYS"=w1133, "INCLINE"=TRUE) -> ("INCLINE-14"=→"INCLINE-14":string)  [unwired: 7 in, 1 out]
                    "MAX" <- w1148
                    "MIN" <- w1147
                  }
                  frame #4 {
                    n830 = local read "MIN"() -> (w1252:dbl)
                    n831 = Number To Fractional String(number=w1252) -> (F-format string=w1251:string)  [unwired: 3 in]
                    n832 = local read "refnum out"() -> (w1249:refnum<file>)
                    n833 = local read "MAX"() -> (w1253:dbl)
                    n834 = call "dataSampled.vi"("Data"=w1251, "refnum in"=w1249) -> ("error out"=w1247:errorcluster, "refnum out"=w1248:refnum<file>)  [unwired: 8 in]
                    n835 = Number To Fractional String(number=w1253) -> (F-format string=w1250:string)  [unwired: 3 in]
                    n836 = call "dataSampled.vi"("Error In"=w1247, "Data"=w1250, "refnum in"=w1248) -> ("error out"=w1245:errorcluster, "refnum out"=w1246:refnum<file>)  [unwired: 7 in]
                    n837 = case shown="True" w1244 {
                      tunnel: w1246 -> [w1255 w1258]
                      tunnel: w1245 -> [w1254 w1257]
                      frame False {
                        n838 = local read "Quickincline"() -> (w1256:bool)
                        n839 = call "Pass_Fail.vi"("error in (no error)"=w1254, "OK"=w1256, "Byte Stream File in"=w1255) -> ()  [unwired: 7 in, 2 out]
                      }
                      frame True {
                        n840 = call "dataSampled.vi"("Error In"=w1257, "refnum in"=w1258) -> ()  [unwired: 8 in, 2 out]
                      }
                    }
                  }
                  frame #5 {
                    n841 = case shown="False" w1259 {
                      tunnel: [w1262 w1274] -> w1260
                      frame False {
                        n842 = while {
                          tunnel: [w1266] -> w1262
                          stop <- w1265 stop-if-true
                          n843 = global read "Global_1259.vi" "EQF1259 com port"() -> (w1263:refnum<visa-resource-name>)
                          n844 = local read "negative incline"() -> (w1273:dbl)
                          n845 = local read "MAX"() -> (w1272:dbl)
                          n846 = call "inclineAquire.vi"("Negative Incline"=w1273, "VISA Refnum in"=w1263) -> ("Incline Out"=w1269:dbl)  [unwired: 8 in, 1 out]
                          n847 = Subtract(x=w1272, y=2.0) -> (x-y=w1270:dbl)
                          n848 = local write "incline"(w1269) -> ()
                          n849 = local read "stopI"() -> (w1267:bool)
                          n850 = Equal?(x=w1269, y=w1270) -> (x = y?=w1264:bool)
                          n851 = Or(x=w1267, y=w1264) -> (x .or. y?=w1265:bool)
                          n852 = Not(x=w1267) -> (.not. x?=w1268:bool)
                          n853 = And(x=w1264, y=w1268) -> (x .and. y?=w1266:bool)
                        }
                        "Down" <- w1262
                      }
                      frame True {
                        n854 = while {
                          tunnel: [w1281] -> w1274
                          stop <- w1279 stop-if-true
                          n855 = global read "Global_1259.vi" "EQF1259 com port"() -> (w1275:refnum<visa-resource-name>)
                          n856 = local read "negative incline"() -> (w1283:dbl)
                          n857 = call "inclineAquire.vi"("Negative Incline"=w1283, "VISA Refnum in"=w1275) -> ("Incline Out"=w1276:dbl)  [unwired: 8 in, 1 out]
                          n858 = local write "incline"(w1276) -> ()
                          n859 = local read "stopI"() -> (w1278:bool)
                          n860 = Equal?(x=w1276, y=2.0) -> (x = y?=w1277:bool)
                          n861 = Or(x=w1277, y=w1278) -> (x .or. y?=w1279:bool)
                          n862 = Not(x=w1278) -> (.not. x?=w1280:bool)
                          n863 = And(x=w1277, y=w1280) -> (x .and. y?=w1281:bool)
                        }
                        n864 = local write "Up"(w1274) -> ()
                      }
                    }
                    n865 = local read "refnum out"() -> (w1261:refnum<file>)
                    n866 = call "Pass_Fail.vi"("OK"=w1260, "Byte Stream File in"=w1261) -> ()  [unwired: 8 in, 2 out]
                  }
                  frame #6 {
                    n867 = case shown="False" w1284 {
                      tunnel: [w1287 w1299] -> w1285
                      frame False {
                        n868 = while {
                          tunnel: [w1292] -> w1287
                          stop <- w1293 stop-if-true
                          n869 = global read "Global_1259.vi" "EQF1259 com port"() -> (w1288:refnum<visa-resource-name>)
                          n870 = local read "negative incline"() -> (w1298:dbl)
                          n871 = local read "MAX"() -> (w1297:dbl)
                          n872 = call "inclineAquire.vi"("Negative Incline"=w1298, "VISA Refnum in"=w1288) -> ("Incline Out"=w1294:dbl)  [unwired: 8 in, 1 out]
                          n873 = Subtract(x=w1297, y=1.0) -> (x-y=w1295:dbl)
                          n874 = local write "incline"(w1294) -> ()
                          n875 = local read "stopI"() -> (w1290:bool)
                          n876 = Equal?(x=w1294, y=w1295) -> (x = y?=w1289:bool)
                          n877 = Or(x=w1290, y=w1289) -> (x .or. y?=w1293:bool)
                          n878 = Not(x=w1290) -> (.not. x?=w1291:bool)
                          n879 = And(x=w1289, y=w1291) -> (x .and. y?=w1292:bool)
                        }
                        "Up" <- w1287
                      }
                      frame True {
                        n880 = while {
                          tunnel: [w1306] -> w1299
                          stop <- w1303 stop-if-true
                          n881 = global read "Global_1259.vi" "EQF1259 com port"() -> (w1300:refnum<visa-resource-name>)
                          n882 = local read "negative incline"() -> (w1308:dbl)
                          n883 = call "inclineAquire.vi"("Negative Incline"=w1308, "VISA Refnum in"=w1300) -> ("Incline Out"=w1301:dbl)  [unwired: 8 in, 1 out]
                          n884 = local write "incline"(w1301) -> ()
                          n885 = local read "stopI"() -> (w1304:bool)
                          n886 = Equal?(x=w1301, y=1.0) -> (x = y?=w1302:bool)
                          n887 = Or(x=w1304, y=w1302) -> (x .or. y?=w1303:bool)
                          n888 = Not(x=w1304) -> (.not. x?=w1305:bool)
                          n889 = And(x=w1302, y=w1305) -> (x .and. y?=w1306:bool)
                        }
                        n890 = local write "Down"(w1299) -> ()
                      }
                    }
                    n891 = local read "refnum out"() -> (w1286:refnum<file>)
                    n892 = call "Pass_Fail.vi"("OK"=w1285, "Byte Stream File in"=w1286) -> ()  [unwired: 8 in, 2 out]
                  }
                  frame #7 {
                    n893 = case shown="True" w1309 {
                      tunnel: [w1311 TRUE] -> w1310
                      frame False {
                        n894 = while {
                          tunnel: [w1320] -> w1311
                          stop <- w1319 stop-if-true
                          n895 = global read "Global_1259.vi" "EQF1259 com port"() -> (w1313:refnum<visa-resource-name>)
                          n896 = local read "negative incline"() -> (w1322:dbl)
                          n897 = call "inclineAquire.vi"("Negative Incline"=w1322, "VISA Refnum in"=w1313) -> ("Incline Out"=w1315:dbl)  [unwired: 8 in, 1 out]
                          n898 = local write "incline"(w1315) -> ()
                          n899 = In Range and Coerce(upper limit=1.0, x=w1315, lower limit=-0.1 ("y")) -> (In Range?=w1316:bool)  [unwired: 1 out]
                          n900 = local read "stopI"() -> (w1317:bool)
                          n901 = Or(x=w1317, y=w1316) -> (x .or. y?=w1319:bool)
                          n902 = Not(x=w1317) -> (.not. x?=w1318:bool)
                          n903 = And(x=w1316, y=w1318) -> (x .and. y?=w1320:bool)
                        }
                        n904 = local read "refnum out"() -> (w1312:refnum<file>)
                        n905 = call "Pass_Fail.vi"("OK"=w1311, "Byte Stream File in"=w1312) -> ()  [unwired: 8 in, 2 out]
                      }
                      frame True {
                        n906 = local read "refnum out"() -> (w1323:refnum<file>)
                        n907 = call "dataSampled.vi"("refnum in"=w1323) -> ()  [unwired: 9 in, 2 out]
                      }
                    }
                    "ZERO" <- w1310
                  }
                  frame #8 {
                    n908 = case shown="True" w1325 {
                      tunnel: [w1327 w1333] -> w1326
                      frame False {
                        n909 = local read "Quickincline"() -> (w1332:bool)
                        n910 = local read "Down"() -> (w1331:bool)
                        n911 = local read "ZERO"() -> (w1329:bool)
                        n912 = local read "Up"() -> (w1330:bool)
                        n913 = Compound Arithmetic op=AND(TRUE ("value"), w1329, w1330, w1331, w1332) -> (w1327:bool)
                      }
                      frame True {
                        n914 = local read "Down"() -> (w1334:bool)
                        n915 = local read "Up"() -> (w1335:bool)
                        n916 = Compound Arithmetic op=AND(TRUE, w1335, w1334) -> (w1333:bool)
                      }
                    }
                    "INCLINE PASS" <- w1326
                  }
                }
              }
            }
          }
        }
        n917 = Select(t=T3."CSafe" ("Tab Control"), s=w915, f=T3."Failed" ("Tab Control")) -> (s? t:f=w916:T3)
      }
      frame "Resistance" {
        w1350 = ""
        w1348 = FALSE
        # "#define RESISTNACE_PROTOCOL         0xA1\n//    #define TAG_RESISTANCE_DRIVER_NONE  1\n//    #define TAG_RESISTANCE_DRIVER_ADC   2\n//    #define TAG_RESISTANCE_DRIVER_RS485 3"
        # "protocolResistance"
        n918 = local write "resistanceArray"(dbl[] [0.0] ("resistanceArray")) -> ()
        n919 = local write "Least"(w1348) -> ()
        n920 = property on="resLower" class="DigNum (strict)"("Visible"=w1348) -> ()  [unwired: 2 in, 2 out]
        n921 = local write "stopR"(w1348) -> ()
        n922 = property on="resUpper" class="DigNum (strict)"("Visible"=w1348) -> ()  [unwired: 2 in, 2 out]
        n923 = property on="RESISTANCE/CURRENT" class="WFChart (strict)"("History Data"=cluster{dbl, dbl}[] []) -> ()  [unwired: 2 in, 2 out]
        n924 = local write "IRun"(w1350) -> ()
        n925 = local write "IPeak"(w1350) -> ()
        n926 = local write "Decrease"(w1348) -> ()
        n927 = local write "QuickResistance"(w1348) -> ()
        n928 = local write "RESISTANCE PASS"(w1348) -> ()
        n929 = local write "overCurrent"(w1348) -> ()
        n930 = local write "Increase"(w1348) -> ()
        n931 = global write "Global_1259.vi" "runCurrent"(w1350) -> ()
        n932 = global read "Global_1259.vi" "maxCurrent"() -> (→"currentMaxResistance":string)
        n933 = global read "Global_1259.vi" "resistanceType"() -> (w1343:string)
        n934 = global read "Global_1259.vi" "RESISTANCE"() -> (w1344:string)
        n935 = Decimal String To Number(string=w1343) -> (number=w1346:i32)  [unwired: 2 in, 1 out]
        n936 = Equal?(x=w1344, y="1") -> (x = y?=w1347:bool)
        n937 = case shown="True" w1347 {
          selector: w1347 -> [_ w1370]
          tunnel: [TRUE w1379] -> w1354
          tunnel: w1346 -> [_ w1378]
          frame False {
            n938 = local read "refnum out"() -> (w1369:refnum<file>)
            n939 = call "dataSampled.vi"("refnum in"=w1369) -> ("error out"=w1362:errorcluster, "refnum out"=w1368:refnum<file>)  [unwired: 9 in]
            n940 = call "dataSampled.vi"("Error In"=w1362, "refnum in"=w1368) -> ("error out"=w1361:errorcluster, "refnum out"=w1367:refnum<file>)  [unwired: 8 in]
            n941 = call "dataSampled.vi"("Error In"=w1361, "refnum in"=w1367) -> ("error out"=w1360:errorcluster, "refnum out"=w1365:refnum<file>)  [unwired: 8 in]
            n942 = call "dataSampled.vi"("Error In"=w1360, "refnum in"=w1365) -> ("error out"=w1359:errorcluster, "refnum out"=w1364:refnum<file>)  [unwired: 8 in]
            n943 = call "dataSampled.vi"("Error In"=w1359, "refnum in"=w1364) -> ("error out"=w1358:errorcluster, "refnum out"=w1363:refnum<file>)  [unwired: 8 in]
            n944 = call "dataSampled.vi"("Error In"=w1358, "refnum in"=w1363) -> ()  [unwired: 8 in, 2 out]
          }
          frame True {
            # "have resistance?"
            n945 = local read "EQF1259 com port"() -> (w1376:refnum<visa-resource-name>)
            n946 = local read "refnum out"() -> (w1374:refnum<file>)
            n947 = call "resistanceScan.vi"("VISA Refnum in"=w1376) -> ("error out"=w1377:errorcluster, "Istring#"=w1375:string)  [unwired: 6 in, 3 out]
            n948 = global write "Global_1259.vi" "runCurrent"(w1375) -> ()
            n949 = global read "Global_1259.vi" "Inspection Point"() -> (w1372:string)
            n950 = call "dataSampled.vi"("Data"=w1375, "refnum in"=w1374) -> ()  [unwired: 8 in, 2 out]
            n951 = Equal?(x=w1372, y="SubAssembly") -> (x = y?=w1371:bool)
            n952 = case shown="False" w1371 {
              tunnel: [w1380 w1753] -> w1379
              tunnel: w1378 -> [w1381 w1752]
              tunnel: w1377 -> [_ w1747]
              tunnel: w1376 -> [_ w1750]
              tunnel: w1370 -> [_ w1751]
              frame True {
                # "quick"
                n953 = case shown="3" w1381 {
                  tunnel: [TRUE w1385 w1567] -> w1380
                  frame 1, Default {
                  }
                  frame 2 {
                    n954 = local read "EQF1259 com port"() -> (w1389:refnum<visa-resource-name>)
                    n955 = call "resistanceCalculator.vi"("VISA Refnum in"=w1389) -> ("steps/button Array"=w1387:dbl[][], "cycle"=w1386:dbl, "No Keys"=w1384:bool)  [unwired: 6 in, 6 out]
                    n956 = for {
                      N: w1386 -> [_]
                      tunnel: w1387 -> [w1564]
                      tunnel: [w1563] -> w1388 mode=indexing
                      i -> [w1561]
                      n957 = Index Array(array=w1564, index (row)=w1561, index (col)=0) -> (element=w1563:dbl)
                    }
                    n958 = Not(x=w1384) -> (.not. x?=w1383:bool)
                    n959 = case shown="False" w1383 {
                      tunnel: w1388 -> [_ w1435]
                      tunnel: w1387 -> [_ w1434]
                      tunnel: w1386 -> [_ w1433]
                      tunnel: [TRUE w1432] -> w1385
                      frame False {
                        n960 = flat-sequence {
                          frame #0 {
                            n961 = for {
                              N: 2 -> [_]
                              n962 = local read "refnum out"() -> (w1392:refnum<file>)
                              n963 = call "dataSampled.vi"("refnum in"=w1392) -> ()  [unwired: 9 in, 2 out]
                            }
                          }
                          frame #1 {
                            n964 = while {
                              shift-right: [w1406] -> _
                              shift-left: _ -> [w1405]
                              tunnel: [w1397] -> w1394
                              stop <- w1402 stop-if-true
                              n965 = local read "currentMaxResistance"() -> (w1409:string)
                              n966 = local read "EQF1259 com port"() -> (w1396:refnum<visa-resource-name>)
                              n967 = call "resistanceScan.vi"("Imax"=w1409, "VISA Refnum in"=w1396) -> ("error out"=w1408:errorcluster, "RESISTANCE/CURRENT"=w1395:cluster{dbl, dbl}, "ADC value"=w1399:dbl, "Istring#"=w1404:string)  [unwired: 5 in, 1 out]
                              n968 = local read "overCurrent"() -> (w1400:bool)
                              n969 = local write "IRun"(w1404) -> ()
                              n970 = local read "stopR"() -> (w1401:bool)
                              n971 = call "currentPeak.vi"("error in (no error)"=w1408, "Istring# change"=w1405, "Istring# scan"=w1404) -> ("Ipeak"=w1407:string, "Irun"=w1406:string)  [unwired: 6 in, 1 out]
                              n972 = local write "RESISTANCE/CURRENT"(w1395) -> ()
                              n973 = Equal?(x=w1399, y=1000.0) -> (x = y?=w1398:bool)
                              n974 = local write "IPeak"(w1407) -> ()
                              n975 = Compound Arithmetic op=OR(w1398, w1401, w1400) -> (w1402:bool)
                              n976 = Not(x=w1401) -> (.not. x?=w1410:bool)
                              n977 = Not(x=w1400) -> (.not. x?=w1411:bool)
                              n978 = Compound Arithmetic op=AND(w1398, w1411, w1410) -> (w1397:bool)
                            }
                            n979 = local read "refnum out"() -> (w1393:refnum<file>)
                            n980 = local write "Increase"(w1394) -> ()
                            n981 = call "Pass_Fail.vi"("OK"=w1394, "Byte Stream File in"=w1393) -> ()  [unwired: 8 in, 2 out]
                          }
                          frame #2 {
                            n982 = while {
                              shift-right: [w1425] -> _
                              shift-left: _ -> [w1424]
                              tunnel: [w1416] -> w1412
                              stop <- w1421 stop-if-true
                              n983 = local read "currentMaxResistance"() -> (w1428:string)
                              n984 = local read "EQF1259 com port"() -> (w1415:refnum<visa-resource-name>)
                              n985 = call "resistanceScan.vi"("Imax"=w1428, "VISA Refnum in"=w1415) -> ("error out"=w1427:errorcluster, "RESISTANCE/CURRENT"=w1414:cluster{dbl, dbl}, "ADC value"=w1418:dbl, "Istring#"=w1423:string)  [unwired: 5 in, 1 out]
                              n986 = local read "overCurrent"() -> (w1419:bool)
                              n987 = local write "IRun"(w1423) -> ()
                              n988 = local read "stopR"() -> (w1420:bool)
                              n989 = local write "RESISTANCE/CURRENT"(w1414) -> ()
                              n990 = call "currentPeak.vi"("error in (no error)"=w1427, "Istring# change"=w1424, "Istring# scan"=w1423) -> ("Ipeak"=w1426:string, "Irun"=w1425:string)  [unwired: 6 in, 1 out]
                              n991 = Equal?(x=w1418, y=500.0) -> (x = y?=w1417:bool)
                              n992 = local write "IPeak"(w1426) -> ()
                              n993 = Compound Arithmetic op=OR(w1417, w1420, w1419) -> (w1421:bool)
                              n994 = Not(x=w1420) -> (.not. x?=w1429:bool)
                              n995 = Not(x=w1419) -> (.not. x?=w1430:bool)
                              n996 = Compound Arithmetic op=AND(w1417, w1430, w1429) -> (w1416:bool)
                            }
                            n997 = local read "refnum out"() -> (w1413:refnum<file>)
                            n998 = local write "Decrease"(w1412) -> ()
                            n999 = call "Pass_Fail.vi"("OK"=w1412, "Byte Stream File in"=w1413) -> ()  [unwired: 8 in, 2 out]
                          }
                          frame #3 {
                            n1000 = local read "refnum out"() -> (w1431:refnum<file>)
                            n1001 = call "dataSampled.vi"("refnum in"=w1431) -> ()  [unwired: 9 in, 2 out]
                          }
                        }
                      }
                      frame True {
                        n1002 = flat-sequence {
                          tunnel: w1435 -> [w1439]
                          tunnel: w1434 -> [w1438]
                          tunnel: w1433 -> [w1437]
                          tunnel: [w1557] -> w1432
                          frame #0 {
                            w1436 = 0
                            n1003 = while {
                              tunnel: w1439 -> [w1442]
                              tunnel: w1438 -> [w1441]
                              tunnel: w1437 -> [w1443]
                              shift-right: [w1444] -> _
                              shift-left: w1436 -> [w1447]
                              shift-right: [w1445] -> _
                              shift-left: w1436 -> [w1446]
                              stop <- w1440 stop-if-true
                              n1004 = case shown="0, Default" w1447 {
                                tunnel: w1446 -> [w1458 w1468 w1492 w1500 w1523]
                                tunnel: [w1458 w1468 w1492 w1499 w1523] -> w1445
                                tunnel: [w1451 w1460 3 ("f") w1494 4 ("f")] -> w1444
                                tunnel: w1443 -> [w1450 w1462 _ _ _]
                                tunnel: w1442 -> [_ w1461 _ _ _]
                                tunnel: w1441 -> [_ _ w1487 _ w1516]
                                tunnel: [FALSE FALSE FALSE FALSE w1515] -> w1440
                                frame 0, Default {
                                n1005 = Random Number (0-1)() -> (number: 0 to 1=w1457:dbl)
                                n1006 = Multiply(x=w1457, y=w1450) -> (x*y=w1456:dbl)
                                n1007 = To Long Integer(number=w1456) -> (32bit integer=w1449:i32)
                                "random" <- w1449
                                n1008 = Greater?(x=w1449, y=3) -> (0:w1453:bool)
                                n1009 = Select(t=1, s=w1453, f=0) -> (s? t:f=w1451:i32)
                                }
                                frame 1 {
                                n1010 = Increment(x=w1462) -> (x+1=w1467:dbl)
                                n1011 = while {
                                tunnel: [w1473] -> w1466
                                tunnel: w1461 -> [w1472]
                                tunnel: w1467 -> [w1469]
                                i -> [w1473]
                                stop <- w1474 stop-if-true
                                n1012 = local read "random"() -> (w1471:i32)
                                n1013 = Equal?(x=w1469, y=w1473) -> (x = y?=w1475:bool)
                                n1014 = Index Array(array=w1472, index=w1473) -> (element=w1470:dbl)
                                n1015 = Equal?(x=w1470, y=w1471) -> (x = y?=w1476:bool)
                                n1016 = Or(x=w1476, y=w1475) -> (x .or. y?=w1474:bool)
                                }
                                "index" <- w1466
                                n1017 = Equal?(x=w1466, y=w1467) -> (x = y?=w1463:bool)
                                n1018 = Select(t=0, s=w1463, f=2) -> (s? t:f=w1460:i32)
                                }
                                frame 2 {
                                n1019 = local read "index"() -> (w1486:i32)
                                n1020 = Index Array(array=w1487, index (row)=w1486) -> (element=w1488:dbl[])  [unwired: 1 in]
                                n1021 = Index Array(array=w1488, index #1=0 ("index"), index #2=1 ("index"), index #3=2 ("index")) -> (element #1=w1483:dbl, element #2=w1481:dbl, element #3=w1482:dbl)
                                n1022 = local write "Press Next"(w1483) -> ()
                                n1023 = Subtract(x=w1481, y=40.0) -> (x-y=w1480:dbl)
                                n1024 = Add(x=w1482, y=110.0) -> (x+y=w1479:dbl)
                                n1025 = local write "max(x,y)"(w1479) -> ()
                                n1026 = local write "min(x,y)"(w1480) -> ()
                                }
                                frame 3 {
                                n1027 = while {
                                shift-right: [w1502] -> _
                                shift-left: _ -> [w1503]
                                stop <- w1512 stop-if-true
                                n1028 = local read "currentMaxResistance"() -> (w1505:string)
                                n1029 = local read "EQF1259 com port"() -> (w1511:refnum<visa-resource-name>)
                                n1030 = local read "max(x,y)"() -> (w1510:i16)
                                n1031 = local read "min(x,y)"() -> (w1509:i16)
                                n1032 = call "resistanceScan.vi"("Imax"=w1505, "VISA Refnum in"=w1511) -> ("RESISTANCE/CURRENT"=w1506:cluster{dbl, dbl}, "ADC value"=w1513:dbl, "overCurrent"=w1508:bool, "Istring#"=w1501:string)  [unwired: 5 in, 1 out]
                                n1033 = local write "IRun"(w1501) -> ()
                                n1034 = local write "RESISTANCE/CURRENT"(w1506) -> ()
                                n1035 = local write "overCurrent"(w1508) -> ()
                                n1036 = In Range and Coerce(upper limit=w1510, x=w1513, lower limit=w1509) -> (In Range?=w1507:bool)  [unwired: 1 out]
                                n1037 = call "currentPeak.vi"("Istring# change"=w1503, "Istring# scan"=w1501) -> ("Ipeak"=w1504:string, "Irun"=w1502:string)  [unwired: 7 in, 1 out]
                                n1038 = local write "IPeak"(w1504) -> ()
                                n1039 = local write "QuickResistance"(w1507) -> ()
                                n1040 = Or(x=w1507, y=w1508) -> (x .or. y?=w1512:bool)
                                }
                                n1041 = Increment(x=w1500) -> (x+1=w1499:i32)
                                n1042 = Equal?(x=w1499, y=2) -> (x = y?=w1497:bool)
                                n1043 = Select(t=4, s=w1497, f=0) -> (s? t:f=w1494:i32)
                                }
                                frame 4 {
                                n1044 = Index Array(array=w1516, index (row) #1=1 ("index (row)"), index (col) #1=2 ("disabled index (col)"), index (row) #2=0 ("disabled index (row)"), index (col) #2=1 ("disabled index (col)")) -> (element #1=w1522:dbl, element #2=w1521:dbl)
                                n1045 = while {
                                tunnel: w1522 -> [w1534]
                                tunnel: w1521 -> [w1533]
                                tunnel: [w1527] -> w1515
                                shift-right: [w1525] -> _
                                shift-left: _ -> [w1526]
                                stop <- w1527 stop-if-true
                                n1046 = local read "currentMaxResistance"() -> (w1524:string)
                                n1047 = local read "EQF1259 com port"() -> (w1532:refnum<visa-resource-name>)
                                n1048 = call "resistanceScan.vi"("Imax"=w1524, "VISA Refnum in"=w1532) -> ("RESISTANCE/CURRENT"=w1530:cluster{dbl, dbl}, "ADC value"=w1535:dbl, "overCurrent"=w1531:bool, "Istring#"=w1528:string)  [unwired: 5 in, 1 out]
                                n1049 = local write "IRun"(w1528) -> ()
                                n1050 = local write "RESISTANCE/CURRENT"(w1530) -> ()
                                n1051 = local write "overCurrent"(w1531) -> ()
                                n1052 = call "currentPeak.vi"("Istring# change"=w1526, "Istring# scan"=w1528) -> ("Ipeak"=w1529:string, "Irun"=w1525:string)  [unwired: 7 in, 1 out]
                                n1053 = In Range and Coerce(upper limit=w1534, x=w1535, lower limit=w1533) -> (In Range?=w1527:bool)  [unwired: 1 out]
                                n1054 = local write "IPeak"(w1529) -> ()
                                n1055 = local write "Least"(w1527) -> ()
                                }
                                }
                              }
                            }
                          }
                          frame #1 {
                            # "least"
                            # "current peak"
                            n1056 = local read "IPeak"() -> (w1537:string)
                            n1057 = local read "refnum out"() -> (w1547:refnum<file>)
                            n1058 = call "dataSampled.vi"("Data"=w1537, "refnum in"=w1547) -> ("error out"=w1545:errorcluster, "refnum out"=w1546:refnum<file>)  [unwired: 8 in]
                            n1059 = case shown="False" FALSE {
                              tunnel: w1545 -> [w1551 w1556]
                              tunnel: w1546 -> [w1550 w1555]
                              tunnel: [w1549 w1553] -> w1543
                              tunnel: [w1548 w1552] -> w1540
                              frame True {
                                n1060 = call "dataSampled.vi"("Error In"=w1551, "refnum in"=w1550) -> ("error out"=w1548:errorcluster, "refnum out"=w1549:refnum<file>)  [unwired: 8 in]
                              }
                              frame False {
                                n1061 = local read "QuickResistance"() -> (w1554:bool)
                                n1062 = call "Pass_Fail.vi"("error in (no error)"=w1556, "OK"=w1554, "Byte Stream File in"=w1555) -> ("error out"=w1552:errorcluster, "Byte Stream File out"=w1553:refnum<file>)  [unwired: 7 in]
                              }
                            }
                            n1063 = call "dataSampled.vi"("Error In"=w1540, "refnum in"=w1543) -> ("error out"=w1539:errorcluster, "refnum out"=w1542:refnum<file>)  [unwired: 8 in]
                            n1064 = call "dataSampled.vi"("Error In"=w1539, "refnum in"=w1542) -> ("error out"=w1538:errorcluster, "refnum out"=w1541:refnum<file>)  [unwired: 8 in]
                            n1065 = local read "Least"() -> (w1544:bool)
                            n1066 = call "Pass_Fail.vi"("error in (no error)"=w1538, "OK"=w1544, "Byte Stream File in"=w1541) -> ()  [unwired: 7 in, 2 out]
                          }
                          frame #2 {
                            n1067 = local read "QuickResistance"() -> (w1559:bool)
                            n1068 = local read "Least"() -> (w1560:bool)
                            n1069 = Compound Arithmetic op=AND(w1559, TRUE, w1560) -> (w1557:bool)
                            n1070 = local write "RESISTANCE PASS"(w1557) -> ()
                          }
                        }
                      }
                    }
                  }
                  frame 3 {
                    n1071 = local read "EQF1259 com port"() -> (w1571:refnum<visa-resource-name>)
                    n1072 = call "gearCalculator.vi"("VISA Refnum in"=w1571) -> ("steps/button Array"=w1569:dbl[][], "No Keys"=w1565:bool, "cycle"=w1568:dbl)  [unwired: 10 in, 2 out]
                    n1073 = for {
                      N: w1568 -> [_]
                      tunnel: w1569 -> [w1741]
                      tunnel: [w1740] -> w1570 mode=indexing
                      i -> [w1738]
                      n1074 = Index Array(array=w1741, index (row)=w1738, index (col)=0) -> (element=w1740:dbl)
                    }
                    n1075 = Not(x=w1565) -> (.not. x?=w1566:bool)
                    n1076 = case shown="False" w1566 {
                      tunnel: w1570 -> [_ w1617]
                      tunnel: w1569 -> [_ w1616]
                      tunnel: w1568 -> [_ w1615]
                      tunnel: [TRUE w1614] -> w1567
                      frame False {
                        n1077 = flat-sequence {
                          frame #0 {
                            n1078 = for {
                              N: 2 -> [_]
                              n1079 = local read "refnum out"() -> (w1574:refnum<file>)
                              n1080 = call "dataSampled.vi"("refnum in"=w1574) -> ()  [unwired: 9 in, 2 out]
                            }
                          }
                          frame #1 {
                            n1081 = while {
                              shift-right: [w1588] -> _
                              shift-left: _ -> [w1587]
                              tunnel: [w1579] -> w1576
                              stop <- w1584 stop-if-true
                              n1082 = local read "currentMaxResistance"() -> (w1591:string)
                              n1083 = local read "EQF1259 com port"() -> (w1578:refnum<visa-resource-name>)
                              n1084 = call "resistanceScan.vi"("Imax"=w1591, "VISA Refnum in"=w1578) -> ("error out"=w1590:errorcluster, "RESISTANCE/CURRENT"=w1577:cluster{dbl, dbl}, "ADC value"=w1581:dbl, "Istring#"=w1586:string)  [unwired: 5 in, 1 out]
                              n1085 = local read "overCurrent"() -> (w1582:bool)
                              n1086 = local write "IRun"(w1586) -> ()
                              n1087 = local read "stopR"() -> (w1583:bool)
                              n1088 = call "currentPeak.vi"("error in (no error)"=w1590, "Istring# change"=w1587, "Istring# scan"=w1586) -> ("Ipeak"=w1589:string, "Irun"=w1588:string)  [unwired: 6 in, 1 out]
                              n1089 = local write "RESISTANCE/CURRENT"(w1577) -> ()
                              n1090 = Equal?(x=w1581, y=1000.0) -> (x = y?=w1580:bool)
                              n1091 = local write "IPeak"(w1589) -> ()
                              n1092 = Compound Arithmetic op=OR(w1580, w1583, w1582) -> (w1584:bool)
                              n1093 = Not(x=w1583) -> (.not. x?=w1592:bool)
                              n1094 = Not(x=w1582) -> (.not. x?=w1593:bool)
                              n1095 = Compound Arithmetic op=AND(w1580, w1593, w1592) -> (w1579:bool)
                            }
                            n1096 = local read "refnum out"() -> (w1575:refnum<file>)
                            n1097 = local write "Increase"(w1576) -> ()
                            n1098 = call "Pass_Fail.vi"("OK"=w1576, "Byte Stream File in"=w1575) -> ()  [unwired: 8 in, 2 out]
                          }
                          frame #2 {
                            n1099 = while {
                              shift-right: [w1607] -> _
                              shift-left: _ -> [w1606]
                              tunnel: [w1598] -> w1594
                              stop <- w1603 stop-if-true
                              n1100 = local read "currentMaxResistance"() -> (w1610:string)
                              n1101 = local read "EQF1259 com port"() -> (w1597:refnum<visa-resource-name>)
                              n1102 = call "resistanceScan.vi"("Imax"=w1610, "VISA Refnum in"=w1597) -> ("error out"=w1609:errorcluster, "RESISTANCE/CURRENT"=w1596:cluster{dbl, dbl}, "ADC value"=w1600:dbl, "Istring#"=w1605:string)  [unwired: 5 in, 1 out]
                              n1103 = local read "overCurrent"() -> (w1601:bool)
                              n1104 = local write "IRun"(w1605) -> ()
                              n1105 = local read "stopR"() -> (w1602:bool)
                              n1106 = local write "RESISTANCE/CURRENT"(w1596) -> ()
                              n1107 = call "currentPeak.vi"("error in (no error)"=w1609, "Istring# change"=w1606, "Istring# scan"=w1605) -> ("Ipeak"=w1608:string, "Irun"=w1607:string)  [unwired: 6 in, 1 out]
                              n1108 = Equal?(x=w1600, y=500.0) -> (x = y?=w1599:bool)
                              n1109 = local write "IPeak"(w1608) -> ()
                              n1110 = Compound Arithmetic op=OR(w1599, w1602, w1601) -> (w1603:bool)
                              n1111 = Not(x=w1602) -> (.not. x?=w1611:bool)
                              n1112 = Not(x=w1601) -> (.not. x?=w1612:bool)
                              n1113 = Compound Arithmetic op=AND(w1599, w1612, w1611) -> (w1598:bool)
                            }
                            n1114 = local read "refnum out"() -> (w1595:refnum<file>)
                            n1115 = local write "Decrease"(w1594) -> ()
                            n1116 = call "Pass_Fail.vi"("OK"=w1594, "Byte Stream File in"=w1595) -> ()  [unwired: 8 in, 2 out]
                          }
                          frame #3 {
                            n1117 = local read "refnum out"() -> (w1613:refnum<file>)
                            n1118 = call "dataSampled.vi"("refnum in"=w1613) -> ()  [unwired: 9 in, 2 out]
                          }
                        }
                      }
                      frame True {
                        n1119 = flat-sequence {
                          tunnel: w1617 -> [w1621]
                          tunnel: w1616 -> [w1620]
                          tunnel: w1615 -> [w1619]
                          tunnel: [w1734] -> w1614
                          frame #0 {
                            w1618 = 0
                            n1120 = while {
                              tunnel: w1621 -> [w1624]
                              tunnel: w1620 -> [w1623]
                              tunnel: w1619 -> [w1625]
                              shift-right: [w1626] -> _
                              shift-left: w1618 -> [w1629]
                              shift-right: [w1627] -> _
                              shift-left: w1618 -> [w1628]
                              stop <- w1622 stop-if-true
                              n1121 = case shown="0, Default" w1629 {
                                tunnel: w1628 -> [w1640 w1650 w1674 w1682 w1705]
                                tunnel: [w1640 w1650 w1674 w1681 w1705] -> w1627
                                tunnel: [w1633 w1642 3 ("f") w1676 4 ("f")] -> w1626
                                tunnel: w1625 -> [w1632 w1644 _ _ _]
                                tunnel: w1624 -> [_ w1643 _ _ _]
                                tunnel: w1623 -> [_ _ w1669 _ w1698]
                                tunnel: [FALSE FALSE FALSE FALSE w1697] -> w1622
                                frame 0, Default {
                                n1122 = Random Number (0-1)() -> (number: 0 to 1=w1639:dbl)
                                n1123 = Multiply(x=w1639, y=w1632) -> (x*y=w1638:dbl)
                                n1124 = To Long Integer(number=w1638) -> (32bit integer=w1631:i32)
                                "random 2" <- w1631
                                n1125 = Greater?(x=w1631, y=3) -> (0:w1635:bool)
                                n1126 = Select(t=1, s=w1635, f=0) -> (s? t:f=w1633:i32)
                                }
                                frame 1 {
                                n1127 = Increment(x=w1644) -> (x+1=w1649:dbl)
                                n1128 = while {
                                tunnel: [w1655] -> w1648
                                tunnel: w1643 -> [w1654]
                                tunnel: w1649 -> [w1651]
                                i -> [w1655]
                                stop <- w1656 stop-if-true
                                n1129 = local read "random 2"() -> (w1653:i32)
                                n1130 = Equal?(x=w1651, y=w1655) -> (x = y?=w1657:bool)
                                n1131 = Index Array(array=w1654, index=w1655) -> (element=w1652:dbl)
                                n1132 = Equal?(x=w1652, y=w1653) -> (x = y?=w1658:bool)
                                n1133 = Or(x=w1658, y=w1657) -> (x .or. y?=w1656:bool)
                                }
                                "index 2" <- w1648
                                n1134 = Equal?(x=w1648, y=w1649) -> (x = y?=w1645:bool)
                                n1135 = Select(t=0, s=w1645, f=2) -> (s? t:f=w1642:i32)
                                }
                                frame 2 {
                                n1136 = local read "index 2"() -> (w1668:i32)
                                n1137 = Index Array(array=w1669, index (row)=w1668) -> (element=w1670:dbl[])  [unwired: 1 in]
                                n1138 = Index Array(array=w1670, index #1=0 ("index"), index #2=1 ("index"), index #3=2 ("index")) -> (element #1=w1665:dbl, element #2=w1661:dbl, element #3=w1660:dbl)
                                n1139 = local write "Press Next"(w1665) -> ()
                                n1140 = Subtract(x=w1661, y=40.0) -> (x-y=w1663:dbl)
                                n1141 = Add(x=w1660, y=110.0) -> (x+y=w1662:dbl)
                                n1142 = local write "max(x,y)"(w1662) -> ()
                                n1143 = local write "min(x,y)"(w1663) -> ()
                                }
                                frame 3 {
                                n1144 = while {
                                shift-right: [w1685] -> _
                                shift-left: _ -> [w1686]
                                stop <- w1694 stop-if-true
                                n1145 = local read "currentMaxResistance"() -> (w1683:string)
                                n1146 = local read "EQF1259 com port"() -> (w1693:refnum<visa-resource-name>)
                                n1147 = local read "min(x,y)"() -> (w1691:i16)
                                n1148 = local read "max(x,y)"() -> (w1692:i16)
                                n1149 = call "resistanceScan.vi"("Imax"=w1683, "VISA Refnum in"=w1693) -> ("RESISTANCE/CURRENT"=w1688:cluster{dbl, dbl}, "ADC value"=w1695:dbl, "overCurrent"=w1690:bool, "Istring#"=w1687:string)  [unwired: 5 in, 1 out]
                                n1150 = local write "RESISTANCE/CURRENT"(w1688) -> ()
                                n1151 = call "currentPeak.vi"("Istring# change"=w1686, "Istring# scan"=w1687) -> ("Ipeak"=w1684:string, "Irun"=w1685:string)  [unwired: 7 in, 1 out]
                                n1152 = local write "IRun"(w1687) -> ()
                                n1153 = local write "overCurrent"(w1690) -> ()
                                n1154 = In Range and Coerce(upper limit=w1692, x=w1695, lower limit=w1691) -> (In Range?=w1689:bool)  [unwired: 1 out]
                                n1155 = local write "IPeak"(w1684) -> ()
                                n1156 = Or(x=w1689, y=w1690) -> (x .or. y?=w1694:bool)
                                n1157 = local write "QuickResistance"(w1689) -> ()
                                }
                                n1158 = Increment(x=w1682) -> (x+1=w1681:i32)
                                n1159 = Equal?(x=w1681, y=2) -> (x = y?=w1679:bool)
                                n1160 = Select(t=4, s=w1679, f=0) -> (s? t:f=w1676:i32)
                                }
                                frame 4 {
                                n1161 = Index Array(array=w1698, index (row) #1=1 ("index (row)"), index (col) #1=2 ("disabled index (col)"), index (row) #2=0 ("disabled index (row)"), index (col) #2=1 ("disabled index (col)")) -> (element #1=w1704:dbl, element #2=w1703:dbl)
                                n1162 = while {
                                tunnel: w1704 -> [w1716]
                                tunnel: w1703 -> [w1715]
                                tunnel: [w1706] -> w1697
                                shift-right: [w1708] -> _
                                shift-left: _ -> [w1707]
                                stop <- w1706 stop-if-true
                                n1163 = local read "currentMaxResistance"() -> (w1710:string)
                                n1164 = local read "EQF1259 com port"() -> (w1714:refnum<visa-resource-name>)
                                n1165 = call "resistanceScan.vi"("Imax"=w1710, "VISA Refnum in"=w1714) -> ("RESISTANCE/CURRENT"=w1712:cluster{dbl, dbl}, "ADC value"=w1717:dbl, "overCurrent"=w1713:bool, "Istring#"=w1709:string)  [unwired: 5 in, 1 out]
                                n1166 = local write "IRun"(w1709) -> ()
                                n1167 = local write "RESISTANCE/CURRENT"(w1712) -> ()
                                n1168 = local write "overCurrent"(w1713) -> ()
                                n1169 = In Range and Coerce(upper limit=w1716, x=w1717, lower limit=w1715) -> (In Range?=w1706:bool)  [unwired: 1 out]
                                n1170 = call "currentPeak.vi"("Istring# change"=w1707, "Istring# scan"=w1709) -> ("Ipeak"=w1711:string, "Irun"=w1708:string)  [unwired: 7 in, 1 out]
                                n1171 = local write "IPeak"(w1711) -> ()
                                n1172 = local write "Least"(w1706) -> ()
                                }
                                }
                              }
                            }
                          }
                          frame #1 {
                            # "least"
                            # "current peak"
                            n1173 = local read "IPeak"() -> (w1726:string)
                            n1174 = local read "refnum out"() -> (w1725:refnum<file>)
                            n1175 = call "dataSampled.vi"("Data"=w1726, "refnum in"=w1725) -> ("error out"=w1723:errorcluster, "refnum out"=w1724:refnum<file>)  [unwired: 8 in]
                            n1176 = case shown="False" FALSE {
                              tunnel: w1723 -> [w1729 w1733]
                              tunnel: w1724 -> [w1728 w1732]
                              tunnel: [w1727 w1730] -> w1720
                              frame True {
                                n1177 = call "dataSampled.vi"("Error In"=w1729, "refnum in"=w1728) -> ("refnum out"=w1727:refnum<file>)  [unwired: 8 in, 1 out]
                              }
                              frame False {
                                n1178 = local read "QuickResistance"() -> (w1731:bool)
                                n1179 = call "Pass_Fail.vi"("error in (no error)"=w1733, "OK"=w1731, "Byte Stream File in"=w1732) -> ("Byte Stream File out"=w1730:refnum<file>)  [unwired: 7 in, 1 out]
                              }
                            }
                            n1180 = call "dataSampled.vi"("refnum in"=w1720) -> ("refnum out"=w1719:refnum<file>)  [unwired: 9 in, 1 out]
                            n1181 = call "dataSampled.vi"("refnum in"=w1719) -> ("refnum out"=w1718:refnum<file>)  [unwired: 9 in, 1 out]
                            n1182 = local read "Least"() -> (w1722:bool)
                            n1183 = call "Pass_Fail.vi"("OK"=w1722, "Byte Stream File in"=w1718) -> ()  [unwired: 8 in, 2 out]
                          }
                          frame #2 {
                            n1184 = local read "QuickResistance"() -> (w1737:bool)
                            n1185 = local read "Least"() -> (w1736:bool)
                            n1186 = Compound Arithmetic op=AND(w1737, TRUE, w1736) -> (w1734:bool)
                            n1187 = local write "RESISTANCE PASS"(w1734) -> ()
                          }
                        }
                      }
                    }
                  }
                }
              }
              frame False {
                # "standard"
                n1188 = global read "Global_1259.vi" "PartNumber"() -> (w1745:string)
                n1189 = global read "Global_1259.vi" "deviceType"() -> (w1742:string)
                n1190 = call "resistanceCalculator.vi"("VISA Refnum in"=w1750, "error in (no error)"=w1747) -> ("No Keys"=w1746:bool, "error out"=w1748:errorcluster)  [unwired: 5 in, 7 out]
                n1191 = Not Equal?(x=w1745, y="400659") -> (x != y?=w1743:bool)
                n1192 = case shown="True" w1743 {
                  tunnel: w1751 -> [_ w1760]
                  tunnel: [w1754 w1759] -> w1749
                  tunnel: w1748 -> [w1754 w1758]
                  tunnel: w1746 -> [_ w1757]
                  tunnel: w1742 -> [_ w1756]
                  frame False {
                    n1193 = local write "RESISTANCE-15"("(W§c6RðS\nN\fÿ\u0006\\\u001c >Pe¦^\u001d ¾n:N7\u0000\u0005ÿ\u00020\n\u0000(W§c6RðS\nN\fÿ\tc\u000bN\u0000Nek\tc®ôv0R1\u00008\u0000\u00020\n\u0000(W§c6RðS\nN\fÿ\u0006\\\u001c >Pe¦^\u001d ¾n:N0\u0000\u0005ÿ\u00020\n\u0000(W§c6RðS\nN\fÿ\tcÏQ;\tc®ôvó\u0007c:y\u00020\n\u0000(W§c6RðS\nN\fÿ\tcX R5u;\tc®ôv0R>f:yúQeg\u00020\n\u0000(W§c6RðS\nN\fÿ\tc\u0000gNOvQ\u0000u\u0000i\u0000c\u0000k\u0000 \u0000R\u0000e\u0000s\u0000i\u0000s\u0000t\u0000a\u0000n\u0000c\u0000e\u0000\tc®\u00020\n\u0000O\u0000n\u0000 \u0000t\u0000h\u0000e\u0000 \u0000c\u0000o\u0000n\u0000s\u0000o\u0000l\u0000e\u0000,\u0000 \u0000s\u0000e\u0000t\u0000 \u0000i\u0000n\u0000c\u0000l\u0000i\u0000n\u0000e\u0000 \u0000t\u0000o\u0000 \u00007\u0000%\u0000.\u0000\n\u0000O\u0000n\u0000 \u0000t\u0000h\u0000e\u0000 \u0000c\u0000o\u0000n\u0000s\u0000o\u0000l\u0000e\u0000,\u0000 \u0000p\u0000r\u0000e\u0000s\u0000s\u0000 \u0000t\u0000h\u0000e\u0000 \u0000n\u0000e\u0000x\u0000t\u0000 \u0000b\u0000u\u0000t\u0000t\u0000o\u0000n\u0000s\u0000 \u0000t\u0000i\u0000l\u0000l\u0000 \u00001\u00008\u0000.\u0000\n\u0000O\u0000n\u0000 \u0000t\u0000h\u0000e\u0000 \u0000c\u0000o\u0000n\u0000s\u0000o\u0000l\u0000e\u0000,\u0000 \u0000s\u0000e\u0000t\u0000 \u0000i\u0000n\u0000c\u0000l\u0000i\u0000n\u0000e\u0000 \u0000t\u0000o\u0000 \u00000\u0000%\u0000.\u0000\n\u0000O\u0000n\u0000 \u0000t\u0000h\u0000e\u0000 \u0000c\u0000o\u0000n\u0000s\u0000o\u0000l\u0000e\u0000,\u0000 \u0000p\u0000r\u0000e\u0000s\u0000s\u0000 \u0000d\u0000e\u0000c\u0000r\u0000e\u0000m\u0000e\u0000n\u0000t\u0000 \u0000r\u0000e\u0000s\u0000i\u0000s\u0000t\u0000a\u0000n\u0000c\u0000e\u0000 \u0000b\u0000u\u0000t\u0000t\u0000o\u0000n\u0000 \u0000t\u0000i\u0000l\u0000l\u0000 \u0000i\u0000n\u0000d\u0000...") -> ()
                  }
                  frame True {
                    n1194 = call "resistancePIP.vi"("error in (no error)"=w1758, "DeviceType"=w1756, "QUICK_KEYS"=w1757, "RESISTANCE"=w1760) -> ("error out"=w1759:errorcluster, "RESISTANCE-15"=→"RESISTANCE-15":string)  [unwired: 6 in]
                  }
                }
                n1195 = case shown="2" w1752 {
                  tunnel: [_ w1765 w1979] -> w1753
                  tunnel: w1749 -> [_ w1764 w1989]
                  tunnel: w1750 -> [_ w1763 w1990]
                  frame 1, Default {
                  }
                  frame 2 {
                    n1196 = flat-sequence {
                      tunnel: [w1781] -> w1773
                      tunnel: [w1774] -> w1772
                      tunnel: [w1777] -> w1771
                      tunnel: w1764 -> [w1776]
                      tunnel: w1763 -> [w1775]
                      tunnel: w1773 -> [w1834]
                      tunnel: [w1834] -> w1770
                      tunnel: w1772 -> [w1833]
                      tunnel: w1771 -> [w1831]
                      tunnel: [w1833] -> w1769
                      tunnel: w1770 -> [w1849]
                      tunnel: [w1849] -> w1768
                      tunnel: w1769 -> [w1848]
                      tunnel: [w1848] -> w1767
                      tunnel: w1768 -> [w1898]
                      tunnel: w1767 -> [w1897]
                      tunnel: [w1897] -> w1766
                      tunnel: w1766 -> [w1940]
                      tunnel: [w1940] -> w1762
                      tunnel: [w1966] -> w1765
                      tunnel: w1762 -> [w1965]
                      frame #0 {
                        n1197 = call "resistanceCalculator.vi"("VISA Refnum in"=w1775, "error in (no error)"=w1776) -> ("steps/button Array"=w1779:dbl[][], "cycle"=w1778:dbl, "No Keys"=w1774:bool)  [unwired: 5 in, 6 out]
                        n1198 = To Long Integer(number=w1778) -> (32bit integer=w1780:i32)
                        n1199 = for {
                          N: w1780 -> [_]
                          tunnel: w1779 -> [w1790]
                          tunnel: [w1785] -> w1782 mode=indexing
                          tunnel: [w1784] -> w1777
                          tunnel: w1774 -> [w1783]
                          i -> [w1789]
                          n1200 = Index Array(array=w1790, index (row)=w1789, index (col)=0 ("disabled index (col)")) -> (element=w1791:dbl)
                          n1201 = Not Equal To 0?(x=w1791) -> (x != 0?=w1787:bool)
                          n1202 = case shown="True" w1787 {
                            selector: w1787 -> [w1814 _]
                            tunnel: w1790 -> [_ w1825]
                            tunnel: w1789 -> [_ w1824]
                            tunnel: [w1814 TRUE] -> w1786
                            frame False {
                            }
                            frame True {
                              n1203 = for {
                                N: 3 -> [_]
                                tunnel: w1825 -> [w1830]
                                tunnel: [w1829] -> w1823 mode=indexing
                                tunnel: w1824 -> [w1828]
                                i -> [w1827]
                                n1204 = Index Array(array=w1830, index (row)=w1828, index (col)=w1827) -> (element=w1829:dbl)
                              }
                              n1205 = Wait (ms)(milliseconds to wait=u32 1250) -> ()  [unwired: 1 out]
                              n1206 = Index Array(array=w1823, index #1=0 ("index"), index #2=1 ("index"), index #3=2 ("index")) -> (element #1=→"Press Next":dbl, element #2=→"resLower":dbl, element #3=→"resUpper":dbl)
                            }
                          }
                          n1207 = case shown="True" w1786 {
                            tunnel: [_ w1794] -> w1785
                            tunnel: [_ w1793] -> w1784
                            tunnel: w1783 -> [w1792 _]
                            frame False {
                              n1208 = local write "QuickResistance"(w1792) -> ()
                            }
                            frame True {
                              n1209 = while {
                                shift-right: [w1803] -> _
                                shift-left: _ -> [w1813]
                                tunnel: [w1810] -> w1794
                                tunnel: [w1795] -> w1793
                                stop <- w1802 stop-if-true
                                n1210 = local read "currentMaxResistance"() -> (w1804:string)
                                n1211 = local read "EQF1259 com port"() -> (w1807:refnum<visa-resource-name>)
                                n1212 = local read "resUpper"() -> (w1798:dbl)
                                n1213 = local read "resLower"() -> (w1808:dbl)
                                n1214 = call "resistanceScan.vi"("Imax"=w1804, "VISA Refnum in"=w1807) -> ("RESISTANCE/CURRENT"=→"RESISTANCE/CURRENT":cluster{dbl, dbl}, "ADC value"=w1810:dbl, "overCurrent"=w1800:bool, "Istring#"=w1809:string)  [unwired: 5 in, 1 out]
                                "IRun" <- w1809
                                "overCurrent" <- w1800
                                n1215 = Subtract(x=w1808, y=40.0) -> (x-y=w1812:dbl)
                                n1216 = Add(x=w1798, y=110.0) -> (x+y=w1799:dbl)
                                n1217 = In Range and Coerce(upper limit=w1799, x=w1810, lower limit=w1812) -> (In Range?=w1796:bool)  [unwired: 1 out]
                                "QuickResistance" <- w1796
                                n1218 = call "currentPeak.vi"("Istring# change"=w1813, "Istring# scan"=w1809) -> ("error out"=w1795:errorcluster, "Ipeak"=→"IPeak":string, "Irun"=w1803:string)  [unwired: 7 in]
                                n1219 = Compound Arithmetic op=OR("stopR", w1800, w1796) -> (w1802:bool)
                              }
                            }
                          }
                        }
                        "resistanceArray" <- w1782
                        n1220 = Decrement(x=w1780) -> (x-1=w1781:i32)
                      }
                      frame #1 {
                        n1221 = local read "refnum out"() -> (w1832:refnum<file>)
                        n1222 = case shown="True" w1833 {
                          tunnel: w1832 -> [w1836 w1843]
                          tunnel: w1831 -> [w1835 w1839]
                          frame True {
                            n1223 = call "dataSampled.vi"("Error In"=w1835, "refnum in"=w1836) -> ("error out"=w1837:errorcluster, "refnum out"=w1838:refnum<file>)  [unwired: 8 in]
                            n1224 = call "dataSampled.vi"("Error In"=w1837, "refnum in"=w1838) -> ()  [unwired: 8 in, 2 out]
                          }
                          frame False {
                            n1225 = local read "IPeak"() -> (w1840:string)
                            n1226 = call "dataSampled.vi"("Error In"=w1839, "Data"=w1840, "refnum in"=w1843) -> ("error out"=w1842:errorcluster, "refnum out"=w1841:refnum<file>)  [unwired: 7 in]
                            n1227 = local read "QuickResistance"() -> (w1844:bool)
                            n1228 = call "Pass_Fail.vi"("error in (no error)"=w1842, "OK"=w1844, "Byte Stream File in"=w1841) -> ()  [unwired: 7 in, 2 out]
                          }
                        }
                      }
                      frame #2 {
                        n1229 = local read "EQF1259 com port"() -> (w1845:refnum<visa-resource-name>)
                        n1230 = case shown="True" w1848 {
                          tunnel: w1845 -> [w1852 w1876]
                          tunnel: [w1850 w1875] -> w1847
                          tunnel: w1849 -> [w1851 _]
                          frame False {
                            n1231 = while {
                              tunnel: w1852 -> [w1867]
                              tunnel: w1851 -> [w1866]
                              shift-right: [w1862] -> _
                              shift-left: _ -> [w1861]
                              tunnel: [w1857] -> w1850
                              stop <- w1858 stop-if-true
                              w1870 = 100.0 ("y")
                              n1232 = local read "resistanceArray"() -> (w1874:dbl[])
                              n1233 = local read "currentMaxResistance"() -> (w1864:string)
                              n1234 = Index Array(array=w1874, index=w1866) -> (element=w1871:dbl)
                              n1235 = Subtract(x=w1871, y=w1870) -> (x-y=w1869:dbl)
                              n1236 = call "resistanceScan.vi"("Imax"=w1864, "VISA Refnum in"=w1867) -> ("error out"=w1853:errorcluster, "RESISTANCE/CURRENT"=w1873:cluster{dbl, dbl}, "ADC value"=w1872:dbl, "Istring#"=w1865:string)  [unwired: 5 in, 1 out]
                              n1237 = local write "IRun"(w1865) -> ()
                              n1238 = local write "RESISTANCE/CURRENT"(w1873) -> ()
                              n1239 = Subtract(x=w1869, y=w1870) -> (x-y=w1868:dbl)
                              n1240 = call "currentPeak.vi"("error in (no error)"=w1853, "Istring# change"=w1861, "Istring# scan"=w1865) -> ("Ipeak"=w1863:string, "Irun"=w1862:string)  [unwired: 6 in, 1 out]
                              n1241 = local read "overCurrent"() -> (w1855:bool)
                              n1242 = local read "stopR"() -> (w1859:bool)
                              n1243 = local write "IPeak"(w1863) -> ()
                              n1244 = In Range and Coerce(upper limit=w1869, x=w1872, lower limit=w1868) -> (In Range?=w1856:bool)  [unwired: 1 out]
                              n1245 = Not(x=w1859) -> (.not. x?=w1860:bool)
                              n1246 = Not(x=w1855) -> (.not. x?=w1854:bool)
                              n1247 = Compound Arithmetic op=OR(w1856, w1855, w1859) -> (w1858:bool)
                              n1248 = Compound Arithmetic op=AND(w1856, w1860, w1854) -> (w1857:bool)
                            }
                            "Decrease" <- w1850
                          }
                          frame True {
                            n1249 = while {
                              tunnel: w1876 -> [w1890]
                              tunnel: [w1883] -> w1875
                              shift-right: [w1888] -> _
                              shift-left: _ -> [w1887]
                              stop <- w1889 stop-if-true
                              n1250 = local read "currentMaxResistance"() -> (w1886:string)
                              n1251 = call "resistanceScan.vi"("Imax"=w1886, "VISA Refnum in"=w1890) -> ("error out"=w1877:errorcluster, "RESISTANCE/CURRENT"=w1893:cluster{dbl, dbl}, "ADC value"=w1892:dbl, "Istring#"=w1885:string)  [unwired: 5 in, 1 out]
                              n1252 = local read "overCurrent"() -> (w1881:bool)
                              n1253 = local write "IRun"(w1885) -> ()
                              n1254 = local write "RESISTANCE/CURRENT"(w1893) -> ()
                              n1255 = local read "stopR"() -> (w1879:bool)
                              n1256 = call "currentPeak.vi"("error in (no error)"=w1877, "Istring# change"=w1887, "Istring# scan"=w1885) -> ("Ipeak"=w1884:string, "Irun"=w1888:string)  [unwired: 6 in, 1 out]
                              n1257 = Greater?(x=w1892, y=1500.0) -> (0:w1880:bool)
                              n1258 = local write "IPeak"(w1884) -> ()
                              n1259 = Compound Arithmetic op=OR(w1880, w1881, w1879) -> (w1889:bool)
                              n1260 = Not(x=w1881) -> (.not. x?=w1878:bool)
                              n1261 = Not(x=w1879) -> (.not. x?=w1882:bool)
                              n1262 = Compound Arithmetic op=AND(w1880, w1878, w1882) -> (w1883:bool)
                            }
                            n1263 = local write "Increase"(w1875) -> ()
                          }
                        }
                        n1264 = local read "refnum out"() -> (w1846:refnum<file>)
                        n1265 = call "Pass_Fail.vi"("OK"=w1847, "Byte Stream File in"=w1846) -> ()  [unwired: 8 in, 2 out]
                      }
                      frame #3 {
                        n1266 = local read "EQF1259 com port"() -> (w1895:refnum<visa-resource-name>)
                        n1267 = case shown="True" w1897 {
                          tunnel: w1898 -> [w1901 _]
                          tunnel: w1895 -> [w1900 w1923]
                          tunnel: [w1899 w1922] -> w1894
                          frame False {
                            n1268 = while {
                              tunnel: w1900 -> [w1917]
                              tunnel: [w1905] -> w1899
                              tunnel: w1901 -> [w1916]
                              shift-right: [w1911] -> _
                              shift-left: _ -> [w1910]
                              stop <- w1906 stop-if-true
                              n1269 = local read "resistanceArray"() -> (w1921:dbl[])
                              n1270 = local read "currentMaxResistance"() -> (w1913:string)
                              n1271 = Index Array(array=w1921, index=w1916) -> (element=w1918:dbl)
                              n1272 = call "resistanceScan.vi"("Imax"=w1913, "VISA Refnum in"=w1917) -> ("RESISTANCE/CURRENT"=w1920:cluster{dbl, dbl}, "ADC value"=w1919:dbl, "Istring#"=w1909:string)  [unwired: 5 in, 2 out]
                              n1273 = Subtract(x=w1918, y=100.0) -> (x-y=w1915:dbl)
                              n1274 = local read "overCurrent"() -> (w1904:bool)
                              n1275 = local write "IRun"(w1909) -> ()
                              n1276 = local read "stopR"() -> (w1907:bool)
                              n1277 = local write "RESISTANCE/CURRENT"(w1920) -> ()
                              n1278 = In Range and Coerce(upper limit=w1918, x=w1919, lower limit=w1915) -> (In Range?=w1903:bool)  [unwired: 1 out]
                              n1279 = call "currentPeak.vi"("Istring# change"=w1910, "Istring# scan"=w1909) -> ("Ipeak"=w1912:string, "Irun"=w1911:string)  [unwired: 7 in, 1 out]
                              n1280 = local write "IPeak"(w1912) -> ()
                              n1281 = Compound Arithmetic op=OR(w1904, w1903, w1907) -> (w1906:bool)
                              n1282 = Not(x=w1907) -> (.not. x?=w1908:bool)
                              n1283 = Not(x=w1904) -> (.not. x?=w1902:bool)
                              n1284 = Compound Arithmetic op=AND(w1903, w1908, w1902) -> (w1905:bool)
                            }
                            "Increase" <- w1899
                          }
                          frame True {
                            n1285 = while {
                              tunnel: w1923 -> [w1938]
                              tunnel: [w1929] -> w1922
                              shift-right: [w1935] -> _
                              shift-left: _ -> [w1934]
                              stop <- w1928 stop-if-true
                              n1286 = local read "currentMaxResistance"() -> (w1937:string)
                              n1287 = call "resistanceScan.vi"("Imax"=w1937, "VISA Refnum in"=w1938) -> ("RESISTANCE/CURRENT"=w1939:cluster{dbl, dbl}, "ADC value"=w1924:dbl, "Istring#"=w1936:string)  [unwired: 5 in, 2 out]
                              n1288 = local read "overCurrent"() -> (w1926:bool)
                              n1289 = local write "IRun"(w1936) -> ()
                              n1290 = local write "RESISTANCE/CURRENT"(w1939) -> ()
                              n1291 = local read "stopR"() -> (w1927:bool)
                              n1292 = call "currentPeak.vi"("Istring# change"=w1934, "Istring# scan"=w1936) -> ("Ipeak"=w1933:string, "Irun"=w1935:string)  [unwired: 7 in, 1 out]
                              n1293 = Less?(x=w1924, y=825.0 ("x")) -> (x < y?=w1930:bool)
                              n1294 = local write "IPeak"(w1933) -> ()
                              n1295 = Compound Arithmetic op=OR(w1926, w1930, w1927) -> (w1928:bool)
                              n1296 = Not(x=w1926) -> (.not. x?=w1932:bool)
                              n1297 = Not(x=w1927) -> (.not. x?=w1931:bool)
                              n1298 = Compound Arithmetic op=AND(w1930, w1932, w1931) -> (w1929:bool)
                            }
                            n1299 = local write "Decrease"(w1922) -> ()
                          }
                        }
                        n1300 = local read "refnum out"() -> (w1896:refnum<file>)
                        n1301 = call "Pass_Fail.vi"("OK"=w1894, "Byte Stream File in"=w1896) -> ()  [unwired: 8 in, 2 out]
                      }
                      frame #4 {
                        n1302 = local read "EQF1259 com port"() -> (w1941:refnum<visa-resource-name>)
                        n1303 = case shown="True" w1940 {
                          tunnel: [w1945 TRUE] -> w1942
                          tunnel: w1941 -> [w1944 _]
                          frame False {
                            n1304 = while {
                              tunnel: [w1954] -> w1945
                              tunnel: w1944 -> [w1960]
                              shift-right: [w1957] -> _
                              shift-left: _ -> [w1955]
                              stop <- w1953 stop-if-true
                              n1305 = local read "currentMaxResistance"() -> (w1959:string)
                              n1306 = call "resistanceScan.vi"("Imax"=w1959, "VISA Refnum in"=w1960) -> ("RESISTANCE/CURRENT"=w1962:cluster{dbl, dbl}, "ADC value"=w1961:dbl, "Istring#"=w1958:string)  [unwired: 5 in, 2 out]
                              n1307 = local write "IRun"(w1958) -> ()
                              n1308 = local write "RESISTANCE/CURRENT"(w1962) -> ()
                              n1309 = call "currentPeak.vi"("Istring# change"=w1955, "Istring# scan"=w1958) -> ("Ipeak"=w1956:string, "Irun"=w1957:string)  [unwired: 7 in, 1 out]
                              n1310 = local read "overCurrent"() -> (w1949:bool)
                              n1311 = In Range and Coerce(upper limit=600.0, x=w1961, lower limit=400.0) -> (In Range?=w1950:bool)  [unwired: 1 out]
                              n1312 = local read "stopR"() -> (w1951:bool)
                              n1313 = local write "IPeak"(w1956) -> ()
                              n1314 = Not(x=w1951) -> (.not. x?=w1952:bool)
                              n1315 = Not(x=w1949) -> (.not. x?=w1948:bool)
                              n1316 = Compound Arithmetic op=OR(w1950, w1949, w1951) -> (w1953:bool)
                              n1317 = Compound Arithmetic op=AND(w1950, w1952, w1948) -> (w1954:bool)
                            }
                            n1318 = local read "refnum out"() -> (w1943:refnum<file>)
                            n1319 = call "Pass_Fail.vi"("OK"=w1945, "Byte Stream File in"=w1943) -> ()  [unwired: 8 in, 2 out]
                          }
                          frame True {
                            n1320 = local read "refnum out"() -> (w1963:refnum<file>)
                            n1321 = call "dataSampled.vi"("refnum in"=w1963) -> ()  [unwired: 9 in, 2 out]
                          }
                        }
                        "Least" <- w1942
                      }
                      frame #5 {
                        n1322 = case shown="True" w1965 {
                          tunnel: [w1967 w1973] -> w1966
                          frame False {
                            n1323 = local read "QuickResistance"() -> (w1969:bool)
                            n1324 = local read "Decrease"() -> (w1970:bool)
                            n1325 = local read "Increase"() -> (w1971:bool)
                            n1326 = local read "Least"() -> (w1972:bool)
                            n1327 = Compound Arithmetic op=AND(TRUE, w1969, w1970, w1971, w1972) -> (w1967:bool)
                          }
                          frame True {
                            n1328 = local read "Decrease"() -> (w1975:bool)
                            n1329 = local read "Increase"() -> (w1976:bool)
                            n1330 = Compound Arithmetic op=AND(TRUE, w1975, w1976) -> (w1973:bool)
                          }
                        }
                        "RESISTANCE PASS" <- w1966
                      }
                    }
                  }
                  frame 3 {
                    n1331 = flat-sequence {
                      tunnel: w1990 -> [w1999]
                      tunnel: w1989 -> [w1998]
                      tunnel: [w1994] -> w1988
                      tunnel: [w1993] -> w1987
                      tunnel: [w1991] -> w1982
                      tunnel: w1988 -> [w2048]
                      tunnel: w1987 -> [w2047]
                      tunnel: [w2047] -> w1986
                      tunnel: [w2046] -> w1983
                      tunnel: w1982 -> [w2046]
                      tunnel: [w2043] -> w1978
                      tunnel: w1986 -> [w2060]
                      tunnel: [w2060] -> w1985
                      tunnel: w1983 -> [w2059]
                      tunnel: [w2059] -> w1981
                      tunnel: w1978 -> [w2058]
                      tunnel: [w2058] -> w1977
                      tunnel: w1985 -> [w2133]
                      tunnel: [w2133] -> w1984
                      tunnel: w1981 -> [w2132]
                      tunnel: w1977 -> [w2131]
                      tunnel: w1984 -> [w2200]
                      tunnel: [w2200] -> w1980
                      tunnel: w1980 -> [w2226]
                      tunnel: [w2225] -> w1979
                      frame #0 {
                        n1332 = call "gearCalculator.vi"("VISA Refnum in"=w1999, "error in (no error)"=w1998) -> ("steps/button Array"=w1996:dbl[][], "No Keys"=w1993:bool, "cycle"=w1997:dbl)  [unwired: 9 in, 2 out]
                        n1333 = To Long Integer(number=w1997) -> (32bit integer=w1992:i32)
                        n1334 = for {
                          N: w1992 -> [_]
                          tunnel: w1996 -> [w2003]
                          tunnel: [w2001] -> w1995 mode=indexing
                          tunnel: [w2000] -> w1994
                          i -> [w2004]
                          n1335 = Index Array(array=w2003, index (row)=w2004, index (col)=0 ("disabled index (col)")) -> (element=w2006:dbl)
                          n1336 = Not Equal To 0?(x=w2006) -> (x != 0?=w2005:bool)
                          n1337 = case shown="True" w2005 {
                            selector: w2005 -> [w2027 _]
                            tunnel: w2003 -> [_ w2036]
                            tunnel: w2004 -> [_ w2035]
                            tunnel: [w2027 TRUE] -> w2002
                            frame False {
                            }
                            frame True {
                              n1338 = for {
                                N: 2 -> [_]
                                tunnel: w2036 -> [w2041]
                                tunnel: w2035 -> [w2039]
                                tunnel: [w2038] -> w2034 mode=indexing
                                i -> [w2040]
                                n1339 = Index Array(array=w2041, index (row)=w2039, index (col)=w2040) -> (element=w2038:dbl)
                              }
                              n1340 = Wait (ms)(milliseconds to wait=u32 1250) -> ()  [unwired: 1 out]
                              n1341 = Index Array(array=w2034, index #1=0 ("index"), index #2=1 ("index")) -> (element #1=w2030:dbl, element #2=→"valueResistance":dbl)
                              n1342 = local write "Press Next"(w2030) -> ()
                            }
                          }
                          n1343 = case shown="True" w2002 {
                            tunnel: [_ w2009] -> w2001
                            tunnel: [_ w2008] -> w2000
                            frame False {
                            }
                            frame True {
                              n1344 = while {
                                shift-right: [w2019] -> _
                                shift-left: _ -> [w2018]
                                tunnel: [w2012] -> w2009
                                tunnel: [w2011] -> w2008
                                stop <- w2026 stop-if-true
                                w2023 = 10.0
                                n1345 = local read "currentMaxResistance"() -> (w2015:string)
                                n1346 = local read "EQF1259 com port"() -> (w2014:refnum<visa-resource-name>)
                                n1347 = local read "valueResistance"() -> (w2020:dbl)
                                n1348 = Add(x=w2020, y=w2023) -> (x+y=w2022:dbl)
                                n1349 = Subtract(x=w2020, y=w2023) -> (x-y=w2021:dbl)
                                n1350 = call "resistanceScan.vi"("Imax"=w2015, "VISA Refnum in"=w2014) -> ("error out"=w2011:errorcluster, "RESISTANCE/CURRENT"=w2017:cluster{dbl, dbl}, "ADC value"=w2012:dbl, "overCurrent"=w2016:bool, "Istring#"=w2013:string)  [unwired: 5 in]
                                n1351 = local read "stopR"() -> (w2025:bool)
                                n1352 = local write "IRun"(w2013) -> ()
                                n1353 = local write "RESISTANCE/CURRENT"(w2017) -> ()
                                n1354 = local write "overCurrent"(w2016) -> ()
                                n1355 = In Range and Coerce(upper limit=w2022, x=w2012, lower limit=w2021) -> (In Range?=w2024:bool)  [unwired: 1 out]
                                n1356 = call "currentPeak.vi"("Istring# change"=w2018, "Istring# scan"=w2013) -> ("Ipeak"=w2010:string, "Irun"=w2019:string)  [unwired: 7 in, 1 out]
                                n1357 = local write "QuickResistance"(w2024) -> ()
                                n1358 = local write "IPeak"(w2010) -> ()
                                n1359 = Compound Arithmetic op=OR(w2024, w2016, w2025) -> (w2026:bool)
                              }
                            }
                          }
                        }
                        n1360 = local write "resistanceArray"(w1995) -> ()
                        n1361 = Decrement(x=w1992) -> (x-1=w1991:i32)
                      }
                      frame #1 {
                        n1362 = local read "refnum out"() -> (w2051:refnum<file>)
                        n1363 = local read "IPeak"() -> (w2042:string)
                        n1364 = call "dataSampled.vi"("Error In"=w2048, "Data"=w2042, "refnum in"=w2051) -> ("error out"=w2049:errorcluster, "refnum out"=w2050:refnum<file>)  [unwired: 7 in]
                        n1365 = case shown="False" w2047 {
                          selector: w2047 -> [w2052 _]
                          tunnel: w2049 -> [w2054 w2057]
                          tunnel: w2050 -> [w2053 w2056]
                          frame True {
                            n1366 = call "dataSampled.vi"("Error In"=w2054, "refnum in"=w2053) -> ()  [unwired: 8 in, 2 out]
                            n1367 = local write "QuickResistance"(w2052) -> ()
                          }
                          frame False {
                            n1368 = local read "QuickResistance"() -> (w2055:bool)
                            n1369 = call "Pass_Fail.vi"("error in (no error)"=w2057, "OK"=w2055, "Byte Stream File in"=w2056) -> ()  [unwired: 7 in, 2 out]
                          }
                        }
                        n1370 = global read "Global_1259.vi" "PartNumber"() -> (w2045:string)
                        n1371 = Not Equal?(x=w2045, y="400659") -> (x != y?=w2043:bool)
                      }
                      frame #2 {
                        n1372 = case shown="False" w2058 {
                          tunnel: w2060 -> [_ w2083]
                          tunnel: w2059 -> [_ w2081]
                          frame False {
                            # "for EBNT71017V1 only"
                            n1373 = while {
                              shift-right: [w2074] -> _
                              shift-left: _ -> [w2075]
                              tunnel: [w2064] -> w2062
                              stop <- w2068 stop-if-true
                              n1374 = local read "currentMaxResistance"() -> (w2080:string)
                              n1375 = local read "EQF1259 com port"() -> (w2063:refnum<visa-resource-name>)
                              n1376 = call "resistanceScan.vi"("Imax"=w2080, "VISA Refnum in"=w2063) -> ("error out"=w2078:errorcluster, "RESISTANCE/CURRENT"=w2079:cluster{dbl, dbl}, "ADC value"=w2073:dbl, "Istring#"=w2076:string)  [unwired: 5 in, 1 out]
                              n1377 = local write "IRun"(w2076) -> ()
                              n1378 = local write "RESISTANCE/CURRENT"(w2079) -> ()
                              n1379 = call "currentPeak.vi"("error in (no error)"=w2078, "Istring# change"=w2075, "Istring# scan"=w2076) -> ("Ipeak"=w2077:string, "Irun"=w2074:string)  [unwired: 6 in, 1 out]
                              n1380 = local read "overCurrent"() -> (w2069:bool)
                              n1381 = local write "IPeak"(w2077) -> ()
                              n1382 = In Range and Coerce(upper limit=2070.0, x=w2073, lower limit=1734.0) -> (In Range?=w2065:bool)  [unwired: 1 out]
                              n1383 = local read "stopR"() -> (w2070:bool)
                              n1384 = Not(x=w2070) -> (.not. x?=w2067:bool)
                              n1385 = Not(x=w2069) -> (.not. x?=w2066:bool)
                              n1386 = Compound Arithmetic op=OR(w2065, w2069, w2070) -> (w2068:bool)
                              n1387 = Compound Arithmetic op=AND(w2065, w2067, w2066) -> (w2064:bool)
                            }
                            n1388 = local read "refnum out"() -> (w2061:refnum<file>)
                            n1389 = local write "Decrease"(w2062) -> ()
                            n1390 = call "Pass_Fail.vi"("OK"=w2062, "Byte Stream File in"=w2061) -> ()  [unwired: 8 in, 2 out]
                          }
                          frame True {
                            n1391 = local read "EQF1259 com port"() -> (w2082:refnum<visa-resource-name>)
                            n1392 = case shown="False" w2083 {
                              tunnel: [w2086 w2111] -> w2085
                              tunnel: w2082 -> [w2088 w2112]
                              tunnel: w2081 -> [w2087 w2113]
                              frame False {
                                n1393 = while {
                                tunnel: [w2105] -> w2086
                                shift-right: [w2095] -> _
                                shift-left: _ -> [w2094]
                                tunnel: w2088 -> [w2089]
                                tunnel: w2087 -> [w2090]
                                stop <- w2108 stop-if-true
                                w2099 = 100.0
                                n1394 = local read "resistanceArray"() -> (w2104:dbl[])
                                n1395 = local read "currentMaxResistance"() -> (w2092:string)
                                n1396 = Index Array(array=w2104, index=w2090) -> (element=w2103:dbl)
                                n1397 = Subtract(x=w2103, y=w2099) -> (x-y=w2100:dbl)
                                n1398 = call "resistanceScan.vi"("Imax"=w2092, "VISA Refnum in"=w2089) -> ("error out"=w2093:errorcluster, "RESISTANCE/CURRENT"=w2091:cluster{dbl, dbl}, "ADC value"=w2101:dbl, "Istring#"=w2096:string)  [unwired: 5 in, 1 out]
                                n1399 = local write "IRun"(w2096) -> ()
                                n1400 = local write "RESISTANCE/CURRENT"(w2091) -> ()
                                n1401 = Subtract(x=w2100, y=w2099) -> (x-y=w2102:dbl)
                                n1402 = call "currentPeak.vi"("error in (no error)"=w2093, "Istring# change"=w2094, "Istring# scan"=w2096) -> ("Ipeak"=w2097:string, "Irun"=w2095:string)  [unwired: 6 in, 1 out]
                                n1403 = local read "overCurrent"() -> (w2107:bool)
                                n1404 = local read "stopR"() -> (w2106:bool)
                                n1405 = local write "IPeak"(w2097) -> ()
                                n1406 = In Range and Coerce(upper limit=w2100, x=w2101, lower limit=w2102) -> (In Range?=w2098:bool)  [unwired: 1 out]
                                n1407 = Not(x=w2106) -> (.not. x?=w2109:bool)
                                n1408 = Not(x=w2107) -> (.not. x?=w2110:bool)
                                n1409 = Compound Arithmetic op=OR(w2098, w2107, w2106) -> (w2108:bool)
                                n1410 = Compound Arithmetic op=AND(w2098, w2109, w2110) -> (w2105:bool)
                                }
                                n1411 = local write "Decrease"(w2086) -> ()
                              }
                              frame True {
                                n1412 = while {
                                shift-right: [w2130] -> _
                                shift-left: _ -> [w2129]
                                tunnel: [w2124] -> w2111
                                tunnel: w2113 -> [_]
                                tunnel: w2112 -> [w2114]
                                stop <- w2119 stop-if-true
                                n1413 = local read "currentMaxResistance"() -> (w2115:string)
                                n1414 = call "resistanceScan.vi"("Imax"=w2115, "VISA Refnum in"=w2114) -> ("error out"=w2125:errorcluster, "RESISTANCE/CURRENT"=w2126:cluster{dbl, dbl}, "ADC value"=w2121:dbl, "Istring#"=w2128:string)  [unwired: 5 in, 1 out]
                                n1415 = local read "overCurrent"() -> (w2117:bool)
                                n1416 = local write "IRun"(w2128) -> ()
                                n1417 = local write "RESISTANCE/CURRENT"(w2126) -> ()
                                n1418 = local read "stopR"() -> (w2118:bool)
                                n1419 = call "currentPeak.vi"("error in (no error)"=w2125, "Istring# change"=w2129, "Istring# scan"=w2128) -> ("Ipeak"=w2127:string, "Irun"=w2130:string)  [unwired: 6 in, 1 out]
                                n1420 = Greater?(x=w2121, y=1000.0) -> (0:w2116:bool)
                                n1421 = local write "IPeak"(w2127) -> ()
                                n1422 = Compound Arithmetic op=OR(w2116, w2117, w2118) -> (w2119:bool)
                                n1423 = Not(x=w2117) -> (.not. x?=w2122:bool)
                                n1424 = Not(x=w2118) -> (.not. x?=w2123:bool)
                                n1425 = Compound Arithmetic op=AND(w2116, w2122, w2123) -> (w2124:bool)
                                }
                                n1426 = local write "Increase"(w2111) -> ()
                              }
                            }
                            n1427 = local read "refnum out"() -> (w2084:refnum<file>)
                            n1428 = call "Pass_Fail.vi"("OK"=w2085, "Byte Stream File in"=w2084) -> ()  [unwired: 8 in, 2 out]
                          }
                        }
                      }
                      frame #3 {
                        n1429 = case shown="False" w2131 {
                          tunnel: w2133 -> [_ w2156]
                          tunnel: w2132 -> [_ w2155]
                          frame False {
                            # "for EBNT71017V1 only"
                            n1430 = while {
                              shift-right: [w2147] -> _
                              shift-left: _ -> [w2148]
                              tunnel: [w2137] -> w2135
                              stop <- w2141 stop-if-true
                              n1431 = local read "currentMaxResistance"() -> (w2153:string)
                              n1432 = local read "EQF1259 com port"() -> (w2136:refnum<visa-resource-name>)
                              n1433 = call "resistanceScan.vi"("Imax"=w2153, "VISA Refnum in"=w2136) -> ("error out"=w2151:errorcluster, "RESISTANCE/CURRENT"=w2152:cluster{dbl, dbl}, "ADC value"=w2146:dbl, "Istring#"=w2149:string)  [unwired: 5 in, 1 out]
                              n1434 = local write "IRun"(w2149) -> ()
                              n1435 = local write "RESISTANCE/CURRENT"(w2152) -> ()
                              n1436 = call "currentPeak.vi"("error in (no error)"=w2151, "Istring# change"=w2148, "Istring# scan"=w2149) -> ("Ipeak"=w2150:string, "Irun"=w2147:string)  [unwired: 6 in, 1 out]
                              n1437 = local read "overCurrent"() -> (w2142:bool)
                              n1438 = local write "IPeak"(w2150) -> ()
                              n1439 = In Range and Coerce(upper limit=2458.0, x=w2146, lower limit=2251.0) -> (In Range?=w2138:bool)  [unwired: 1 out]
                              n1440 = local read "stopR"() -> (w2143:bool)
                              n1441 = Not(x=w2143) -> (.not. x?=w2140:bool)
                              n1442 = Not(x=w2142) -> (.not. x?=w2139:bool)
                              n1443 = Compound Arithmetic op=OR(w2138, w2142, w2143) -> (w2141:bool)
                              n1444 = Compound Arithmetic op=AND(w2138, w2140, w2139) -> (w2137:bool)
                            }
                            n1445 = local read "refnum out"() -> (w2134:refnum<file>)
                            n1446 = local write "Increase"(w2135) -> ()
                            n1447 = call "Pass_Fail.vi"("OK"=w2135, "Byte Stream File in"=w2134) -> ()  [unwired: 8 in, 2 out]
                          }
                          frame True {
                            n1448 = local read "EQF1259 com port"() -> (w2157:refnum<visa-resource-name>)
                            n1449 = case shown="True" w2156 {
                              tunnel: w2157 -> [w2161 w2183]
                              tunnel: [w2159 w2182] -> w2154
                              tunnel: w2155 -> [w2160 _]
                              frame False {
                                n1450 = while {
                                tunnel: w2161 -> [w2177]
                                tunnel: [w2166] -> w2159
                                shift-right: [w2172] -> _
                                shift-left: _ -> [w2171]
                                tunnel: w2160 -> [w2162]
                                stop <- w2167 stop-if-true
                                n1451 = local read "resistanceArray"() -> (w2181:dbl[])
                                n1452 = local read "currentMaxResistance"() -> (w2174:string)
                                n1453 = Index Array(array=w2181, index=w2162) -> (element=w2178:dbl)
                                n1454 = call "resistanceScan.vi"("Imax"=w2174, "VISA Refnum in"=w2177) -> ("RESISTANCE/CURRENT"=w2180:cluster{dbl, dbl}, "ADC value"=w2179:dbl, "Istring#"=w2170:string)  [unwired: 5 in, 2 out]
                                n1455 = Subtract(x=w2178, y=100.0) -> (x-y=w2176:dbl)
                                n1456 = local read "overCurrent"() -> (w2165:bool)
                                n1457 = local write "IRun"(w2170) -> ()
                                n1458 = local read "stopR"() -> (w2168:bool)
                                n1459 = local write "RESISTANCE/CURRENT"(w2180) -> ()
                                n1460 = In Range and Coerce(upper limit=w2178, x=w2179, lower limit=w2176) -> (In Range?=w2164:bool)  [unwired: 1 out]
                                n1461 = call "currentPeak.vi"("Istring# change"=w2171, "Istring# scan"=w2170) -> ("Ipeak"=w2173:string, "Irun"=w2172:string)  [unwired: 7 in, 1 out]
                                n1462 = local write "IPeak"(w2173) -> ()
                                n1463 = Compound Arithmetic op=OR(w2165, w2164, w2168) -> (w2167:bool)
                                n1464 = Not(x=w2168) -> (.not. x?=w2169:bool)
                                n1465 = Not(x=w2165) -> (.not. x?=w2163:bool)
                                n1466 = Compound Arithmetic op=AND(w2164, w2169, w2163) -> (w2166:bool)
                                }
                                n1467 = local write "Increase"(w2159) -> ()
                              }
                              frame True {
                                n1468 = while {
                                tunnel: w2183 -> [w2198]
                                tunnel: [w2189] -> w2182
                                shift-right: [w2195] -> _
                                shift-left: _ -> [w2194]
                                stop <- w2188 stop-if-true
                                n1469 = local read "currentMaxResistance"() -> (w2197:string)
                                n1470 = call "resistanceScan.vi"("Imax"=w2197, "VISA Refnum in"=w2198) -> ("RESISTANCE/CURRENT"=w2199:cluster{dbl, dbl}, "ADC value"=w2184:dbl, "Istring#"=w2196:string)  [unwired: 5 in, 2 out]
                                n1471 = local read "overCurrent"() -> (w2186:bool)
                                n1472 = local write "IRun"(w2196) -> ()
                                n1473 = local write "RESISTANCE/CURRENT"(w2199) -> ()
                                n1474 = local read "stopR"() -> (w2187:bool)
                                n1475 = call "currentPeak.vi"("Istring# change"=w2194, "Istring# scan"=w2196) -> ("Ipeak"=w2193:string, "Irun"=w2195:string)  [unwired: 7 in, 1 out]
                                n1476 = Less?(x=w2184, y=500.0 ("x")) -> (x < y?=w2190:bool)
                                n1477 = local write "IPeak"(w2193) -> ()
                                n1478 = Compound Arithmetic op=OR(w2186, w2190, w2187) -> (w2188:bool)
                                n1479 = Not(x=w2186) -> (.not. x?=w2192:bool)
                                n1480 = Not(x=w2187) -> (.not. x?=w2191:bool)
                                n1481 = Compound Arithmetic op=AND(w2190, w2192, w2191) -> (w2189:bool)
                                }
                                n1482 = local write "Decrease"(w2182) -> ()
                              }
                            }
                            n1483 = local read "refnum out"() -> (w2158:refnum<file>)
                            n1484 = call "Pass_Fail.vi"("OK"=w2154, "Byte Stream File in"=w2158) -> ()  [unwired: 8 in, 2 out]
                          }
                        }
                      }
                      frame #4 {
                        n1485 = local read "EQF1259 com port"() -> (w2201:refnum<visa-resource-name>)
                        n1486 = case shown="False" w2200 {
                          tunnel: [w2205 TRUE] -> w2202
                          tunnel: w2201 -> [w2204 _]
                          frame False {
                            n1487 = while {
                              tunnel: [w2214] -> w2205
                              tunnel: w2204 -> [w2220]
                              shift-right: [w2217] -> _
                              shift-left: _ -> [w2215]
                              stop <- w2213 stop-if-true
                              n1488 = local read "currentMaxResistance"() -> (w2219:string)
                              n1489 = call "resistanceScan.vi"("Imax"=w2219, "VISA Refnum in"=w2220) -> ("RESISTANCE/CURRENT"=w2222:cluster{dbl, dbl}, "ADC value"=w2221:dbl, "Istring#"=w2218:string)  [unwired: 5 in, 2 out]
                              n1490 = local write "IRun"(w2218) -> ()
                              n1491 = local write "RESISTANCE/CURRENT"(w2222) -> ()
                              n1492 = call "currentPeak.vi"("Istring# change"=w2215, "Istring# scan"=w2218) -> ("Ipeak"=w2216:string, "Irun"=w2217:string)  [unwired: 7 in, 1 out]
                              n1493 = local read "overCurrent"() -> (w2209:bool)
                              n1494 = In Range and Coerce(upper limit=310.0, x=w2221, lower limit=194.0) -> (In Range?=w2210:bool)  [unwired: 1 out]
                              n1495 = local read "stopR"() -> (w2211:bool)
                              n1496 = local write "IPeak"(w2216) -> ()
                              n1497 = Not(x=w2211) -> (.not. x?=w2212:bool)
                              n1498 = Not(x=w2209) -> (.not. x?=w2208:bool)
                              n1499 = Compound Arithmetic op=OR(w2210, w2209, w2211) -> (w2213:bool)
                              n1500 = Compound Arithmetic op=AND(w2210, w2212, w2208) -> (w2214:bool)
                            }
                            n1501 = local read "refnum out"() -> (w2203:refnum<file>)
                            n1502 = call "Pass_Fail.vi"("OK"=w2205, "Byte Stream File in"=w2203) -> ()  [unwired: 8 in, 2 out]
                          }
                          frame True {
                            n1503 = local read "refnum out"() -> (w2223:refnum<file>)
                            n1504 = call "dataSampled.vi"("refnum in"=w2223) -> ()  [unwired: 9 in, 2 out]
                          }
                        }
                        n1505 = local write "Least"(w2202) -> ()
                      }
                      frame #5 {
                        n1506 = case shown="False" w2226 {
                          tunnel: [w2227 w2233] -> w2225
                          frame False {
                            n1507 = local read "QuickResistance"() -> (w2229:bool)
                            n1508 = local read "Decrease"() -> (w2230:bool)
                            n1509 = local read "Increase"() -> (w2231:bool)
                            n1510 = local read "Least"() -> (w2232:bool)
                            n1511 = Compound Arithmetic op=AND(TRUE, w2229, w2230, w2231, w2232) -> (w2227:bool)
                          }
                          frame True {
                            n1512 = local read "Decrease"() -> (w2235:bool)
                            n1513 = local read "Increase"() -> (w2236:bool)
                            n1514 = Compound Arithmetic op=AND(TRUE, w2235, w2236) -> (w2233:bool)
                          }
                        }
                        n1515 = local write "RESISTANCE PASS"(w2225) -> ()
                      }
                    }
                  }
                }
              }
            }
          }
        }
        n1516 = Select(t=T3."Incline" ("Tab Control"), s=w1354, f=T3."Failed" ("Tab Control")) -> (s? t:f=w1357:T3)
      }
      frame "Pulse" {
        w2237 = FALSE
        n1517 = local write "BLE PULSE"(u32 0 ("Waveform Chart")) -> ()
        n1518 = local write "PUL0"(w2237) -> ()
        n1519 = local write "PUL1"(w2237) -> ()
        n1520 = property on="BLE PULSE" class="WFChart (strict)"("History Data"=u32[] []) -> ()  [unwired: 2 in, 2 out]
        n1521 = local write "Hand/Thumb Pass"(w2237) -> ()
        n1522 = local write "BLE_HRM Pass"(w2237) -> ()
        n1523 = local write "E-stopHRM"(w2237) -> ()
        n1524 = global read "Global_1259.vi" "pulseType"() -> (w2238:string)
        n1525 = Not Equal?(x=w2238, y="1") -> (x != y?=w2245:bool)
        n1526 = case shown="True" w2245 {
          tunnel: [TRUE w2251] -> w2244
          frame False {
            n1527 = local read "refnum out"() -> (w2250:refnum<file>)
            n1528 = call "dataSampled.vi"("refnum in"=w2250) -> ()  [unwired: 9 in, 2 out]
          }
          frame True {
            n1529 = local read "EQF1259 com port"() -> (w2258:refnum<visa-resource-name>)
            n1530 = call "1259_usbCommand.vi"("write buffer"="'\u0001", "VISA resource name in"=w2258) -> ("error out"=w2261:errorcluster)  [unwired: 8 in, 1 out]
            n1531 = call "pulsePIP.vi"("error in (no error)"=w2261) -> ("error out"=w2257:errorcluster, "PULSE-17"=→"PULSE-17":string)  [unwired: 9 in]
            n1532 = while {
              shift-right: [w2270] -> _
              shift-left: T6."verifyHand_Thumb" -> [w2271]
              tunnel: w2258 -> [w2268]
              tunnel: w2257 -> [w2267]
              tunnel: [w2267] -> w2256
              tunnel: [w2266] -> w2255
              tunnel: [w2265] -> w2254
              stop <- w2269 stop-if-true
              n1533 = case shown="\"statusBLE_HRM\"" w2271 {
                tunnel: [w2279 T6."readBLE_HRM" T6."statusBLE_HRM" w2326] -> w2270
                tunnel: [w2278 FALSE FALSE w2323] -> w2269
                tunnel: w2268 -> [w2277 w2306 w2312 w2320]
                tunnel: [FALSE w2305 w2311 w2319] -> w2266
                tunnel: [w2275 w2305 w2311 w2318] -> w2265
                frame "verifyHand_Thumb", Default {
                  n1534 = global read "Global_1259.vi" "pulseType"() -> (w2272:string)
                  n1535 = Not Equal?(x=w2272, y="32") -> (x != y?=w2274:bool)
                  n1536 = case shown="False" w2274 {
                    tunnel: [T6."startBLE_HRM" w2291] -> w2279
                    tunnel: [FALSE w2290] -> w2278
                    tunnel: w2277 -> [w2285 w2289]
                    tunnel: [w2283 w2288] -> w2275
                    frame False {
                      w2283 = TRUE
                      n1537 = call "1259_usbUart.vi"("VISA resource name"=w2285, "write buffer"="\u0002\u0001", "sdFeature"=FALSE) -> ("number[0]"=w2281:u32)  [unwired: 1 in, 15 out]
                      n1538 = local write "BLE Status"(w2281) -> ()
                      n1539 = local write "Hand/Thumb Pass"(w2283) -> ()
                      n1540 = local write "PUL1"(w2283) -> ()
                      n1541 = Wait (ms)(milliseconds to wait=u32 250) -> ()  [unwired: 1 out]
                    }
                    frame True {
                      n1542 = while {
                        tunnel: [w2302] -> w2291
                        tunnel: [w2293] -> w2290
                        tunnel: w2289 -> [w2297]
                        tunnel: [w2292] -> w2288
                        stop <- w2295 stop-if-true
                        w2301 = T6."startBLE_HRM"
                        n1543 = call "1259_usbUart.vi"("VISA resource name"=w2297, "write buffer"="\u0002\u0001", "sdFeature"=FALSE) -> ("number[0]"=w2298:u32)  [unwired: 1 in, 15 out]
                        n1544 = local write "BLE Status"(w2298) -> ()
                        n1545 = Not(x="PUL0") -> (.not. x?=w2303:bool)
                        n1546 = Or(x="PUL0", y="PUL1") -> (x .or. y?=w2295:bool)
                        n1547 = Compound Arithmetic op=AND(TRUE ("value"), "PUL1", w2303) -> (w2292:bool)
                        "Hand/Thumb Pass" <- w2292
                        n1548 = Select(t=w2301, s=w2292, f=w2301) -> (s? t:f=w2302:T6)
                        n1549 = Not(x=w2292) -> (.not. x?=w2293:bool)
                      }
                    }
                  }
                }
                frame "startBLE_HRM" {
                  w2305 = FALSE ("Hand/Thumb Pass")
                  n1550 = call "1259_usbCommand.vi"("write buffer"="\u000b\u0001", "VISA resource name in"=w2306) -> ()  [unwired: 8 in, 2 out]
                  n1551 = Wait (ms)(milliseconds to wait=u32 250) -> ()  [unwired: 1 out]
                }
                frame "readBLE_HRM" {
                  w2311 = FALSE ("Hand/Thumb Pass")
                  n1552 = call "1259_usbUart.vi"("VISA resource name"=w2312, "write buffer"="F\u0001", "sdFeature"=FALSE) -> ("number[0]"=→"BLE_BPM" →"BLE PULSE":u32)  [unwired: 1 in, 15 out]
                }
                frame "statusBLE_HRM" {
                  n1553 = call "1259_usbUart.vi"("VISA resource name"=w2320, "write buffer"="\u0002\u0001", "sdFeature"=FALSE) -> ("number[0]"=w2330:u32)  [unwired: 1 in, 15 out]
                  "BLE Status" <- w2330
                  n1554 = case shown="True" "E-stopHRM" {
                    selector: "E-stopHRM" -> [w2331 w2333]
                    tunnel: [w2331 w2333] -> w2321
                    tunnel: w2320 -> [_ w2332]
                    frame False {
                    }
                    frame True {
                      n1555 = call "1259_usbCommand.vi"("write buffer"="\u000b\u0000", "VISA resource name in"=w2332) -> ()  [unwired: 8 in, 2 out]
                    }
                  }
                  n1556 = Equal?(x=u32 2, y=w2330) -> (x = y?=w2319:bool)
                  "BLE_HRM Pass" <- w2319
                  n1557 = Or(x=w2321, y=w2319) -> (x .or. y?=w2323:bool)
                  n1558 = Select(t=T6."statusBLE_HRM", s=w2319, f=T6."readBLE_HRM") -> (s? t:f=w2326:T6)
                  n1559 = local read "Hand/Thumb Pass"() -> (w2318:bool)
                }
              }
            }
            n1560 = Equal?(x=w2255, y=w2254) -> (x = y?=w2252:bool)
            n1561 = case shown="True" w2252 {
              selector: w2252 -> [w2335 w2341]
              tunnel: [w2336 w2342] -> w2260
              tunnel: w2256 -> [w2336 w2343]
              tunnel: [w2335 w2341] -> w2251
              frame False {
              }
              frame True {
                # "This is 1 second / per 10 samples"
                n1562 = while {
                  tunnel: [w2349] -> w2338 mode=indexing
                  i -> [w2347]
                  stop <- w2348 stop-if-true
                  n1563 = local read "EQF1259 com port"() -> (w2345:refnum<visa-resource-name>)
                  n1564 = Equal?(x=25, y=w2347) -> (x = y?=w2348:bool)
                  n1565 = call "currentScan.vi"("VISA resource name"=w2345) -> ("Ichart"=w2349:dbl)  [unwired: 7 in, 3 out]
                }
                n1566 = local read "refnum out"() -> (w2344:refnum<file>)
                n1567 = call-poly <vilib>:"Mean.vi"("X"=w2338) -> ("mean"=w2339:dbl)  [unwired: 1 out]
                n1568 = call "Pass_Fail.vi"("error in (no error)"=w2343, "OK"=w2341, "Byte Stream File in"=w2344) -> ("error out"=w2342:errorcluster)  [unwired: 7 in, 1 out]
                n1569 = Number To Fractional String(number=w2339, precision (6)=i16 2) -> (F-format string=w2340:string)  [unwired: 2 in]
                n1570 = global write "Global_1259.vi" "BaseCurrent"(w2340) -> ()
              }
            }
            n1571 = local read "EQF1259 com port"() -> (w2253:refnum<visa-resource-name>)
            n1572 = call "1259_usbCommand.vi"("error in (no error)"=w2260, "write buffer"="'\u0000", "VISA resource name in"=w2253) -> ()  [unwired: 7 in, 2 out]
          }
        }
        n1573 = Select(t=T3."Fan" ("Tab Control"), s=w2244, f=T3."Failed" ("Tab Control")) -> (s? t:f=w2246:T3)
      }
      frame "Fan" {
        w2350 = "0.00" ("runCurrent")
        w2362 = FALSE
        n1574 = local write "FanCurrent"(0.0 ("CURRENT")) -> ()
        n1575 = local write "Ifan"(w2350) -> ()
        n1576 = property on="FanCurrent" class="WFChart (strict)"("History Data"=dbl[] []) -> ()  [unwired: 2 in, 2 out]
        n1577 = local write "FAN1"(w2362) -> ()
        n1578 = local write "FAN0"(w2362) -> ()
        n1579 = local write "fanIPeak"(w2350) -> ()
        n1580 = global write "Global_1259.vi" "runCurrent"(w2350) -> ()
        n1581 = local write "limitFan"(w2362) -> ()
        n1582 = flat-sequence {
          tunnel: [w2367] -> w2353
          tunnel: [w2374] -> w2355
          tunnel: [w2373] -> w2354
          tunnel: w2353 -> [w2373]
          tunnel: w2355 -> [w2384]
          tunnel: [w2384] -> w2357
          tunnel: [w2381] -> w2356
          tunnel: w2354 -> [w2379]
          tunnel: w2357 -> [w2387]
          tunnel: [w2388] -> w2359
          tunnel: [w2389] -> w2358
          tunnel: w2356 -> [w2389]
          frame #0 {
            n1583 = global read "Global_1259.vi" "FAN"() -> (w2369:string)
            "FAN" <- w2369
            n1584 = Not Equal?(x=w2369, y="0") -> (x != y?=w2367:bool)
          }
          frame #1 {
            # "% multiplier"
            n1585 = local read "EQF1259 com port"() -> (w2372:refnum<visa-resource-name>)
            n1586 = call "1259_usbUart.vi"("VISA resource name"=w2372, "write buffer"="b\u0001", "sdFeature"=FALSE) -> ("byte[0]"=w2370:string, "error out"=w2374:errorcluster)  [unwired: 1 in, 14 out]
            n1587 = global write "Global_1259.vi" "fanType"(w2370) -> ()
            n1588 = case shown="\"01\", Default" w2370 {
              frame "01", Default {
                # "2-pin"
                n1589 = global write "Global_1259.vi" "tempNumeric"(0.25) -> ()
              }
              frame "02" {
                # "3-pin"
                n1590 = global write "Global_1259.vi" "tempNumeric"(0.6) -> ()
              }
              frame "04" {
                # "2 and 3-pin"
                n1591 = global write "Global_1259.vi" "tempNumeric"(0.7) -> ()
              }
            }
          }
          frame #2 {
            # "Verifies that config is correct"
            n1592 = global read "Global_1259.vi" "fanType"() -> (w2383:string)
            "fanType" <- w2383
            n1593 = Not Equal?(x=w2383, y="0") -> (x != y?=w2380:bool)
            n1594 = And(x=w2380, y=w2379) -> (x .and. y?=w2381:bool)
          }
          frame #3 {
            n1595 = global read "Global_1259.vi" "maxCurrent"() -> (w2386:string)
            "currentMaxFan" <- w2386
            n1596 = Fract/Exp String To Number(string=w2386) -> (number=w2385:dbl)  [unwired: 3 in, 1 out]
            n1597 = property on="FanCurrent" class="WFChart (strict)"(error in=w2387, "YScale.Maximum"=w2385) -> (error out=w2388:errorcluster)  [unwired: 1 in, 1 out]
          }
        }
        n1598 = case shown="True" w2358 {
          tunnel: [TRUE w2400] -> w2366
          tunnel: w2359 -> [w2390 w2398]
          frame False {
            n1599 = local read "refnum out"() -> (w2392:refnum<file>)
            n1600 = call "dataSampled.vi"("Error In"=w2390, "refnum in"=w2392) -> ()  [unwired: 8 in, 2 out]
          }
          frame True {
            n1601 = call "fanPIP.vi"() -> ("FAN-18"=→"FAN-18":string)  [unwired: 10 in, 1 out]
            n1602 = while {
              tunnel: [w2406] -> w2400
              tunnel: w2398 -> [w2405]
              tunnel: [w2404] -> w2397
              shift-right: [w2402] -> _
              shift-left: enum16{"High", "Low"}."High" -> [w2403]
              stop <- w2401 stop-if-true
              n1603 = case shown="\"High\", Default" w2403 {
                tunnel: [w2409 w2440] -> w2406
                tunnel: w2405 -> [_ w2439]
                tunnel: [w2408 w2436] -> w2404
                tunnel: [enum16{"High", "Low"}."Low" enum16{"High", "Low"}."Low"] -> w2402
                tunnel: [FALSE TRUE] -> w2401
                frame "High", Default {
                  n1604 = while {
                    tunnel: [w2423] -> w2409
                    shift-right: [w2413] -> _
                    shift-left: _ -> [w2420]
                    tunnel: [w2411] -> w2408
                    stop <- w2424 stop-if-true
                    n1605 = local read "EQF1259 com port"() -> (w2417:refnum<visa-resource-name>)
                    n1606 = local read "currentMaxFan"() -> (w2416:string)
                    n1607 = global read "Global_1259.vi" "PowerMode"() -> (w2419:string)
                    n1608 = local read "FAN0"() -> (w2415:bool)
                    n1609 = call "currentScan.vi"("Imax"=w2416, "VISA resource name"=w2417) -> ("max"=w2412:bool, "Istring"=w2413:string, "Ichart"=w2414:dbl)  [unwired: 6 in, 1 out]
                    n1610 = local write "FanCurrent"(w2414) -> ()
                    n1611 = local write "Ifan"(w2413) -> ()
                    n1612 = local write "limitFan"(w2412) -> ()
                    n1613 = case shown="\"On\"" w2419 {
                      tunnel: [FALSE w2433 w2435] -> w2418
                      tunnel: w2413 -> [_ w2432 _]
                      frame "Off", Default {
                        # "Why would I be Off"
                      }
                      frame "On" {
                        w2431 = 1.0 ("default (0 DBL)")
                        # "Lower limit control"
                        n1614 = global read "Global_1259.vi" "BaseCurrent"() -> (w2430:string)
                        n1615 = Fract/Exp String To Number(string=w2432, default (0 dbl)=w2431) -> (number=w2434:dbl)  [unwired: 2 in, 1 out]
                        n1616 = global read "Global_1259.vi" "tempNumeric"() -> (w2426:dbl)
                        n1617 = Fract/Exp String To Number(string=w2430, default (0 dbl)=w2431) -> (number=w2428:dbl)  [unwired: 2 in, 1 out]
                        n1618 = Multiply(x=w2428, y=w2426) -> (x*y=w2429:dbl)
                        n1619 = Add(x=w2428, y=w2429) -> (x+y=w2427:dbl)
                        n1620 = Greater Or Equal?(x=w2434, y=w2427) -> (x >= y?=w2433:bool)
                      }
                      frame "Battery" {
                        n1621 = local read "FAN1"() -> (w2435:bool)
                      }
                    }
                    n1622 = call "currentPeak.vi"("Istring# change"=w2420, "Istring# scan"=w2413) -> ("Ipeak"=w2411:string)  [unwired: 7 in, 2 out]
                    n1623 = Not(x=w2415) -> (.not. x?=w2422:bool)
                    n1624 = Not(x=w2412) -> (.not. x?=w2421:bool)
                    n1625 = local write "fanIPeak"(w2411) -> ()
                    n1626 = Compound Arithmetic op=OR(w2418, w2415, w2412) -> (w2424:bool)
                    n1627 = Compound Arithmetic op=AND(w2418, w2422, w2421) -> (w2423:bool)
                  }
                }
                frame "Low" {
                  n1628 = while {
                    tunnel: [w2449] -> w2440
                    tunnel: w2439 -> [_]
                    shift-right: [w2443] -> _
                    shift-left: _ -> [w2446]
                    tunnel: [w2441] -> w2436
                    stop <- w2454 stop-if-true
                    n1629 = local read "EQF1259 com port"() -> (w2452:refnum<visa-resource-name>)
                    n1630 = local read "currentMaxFan"() -> (w2451:string)
                    n1631 = global read "Global_1259.vi" "PowerMode"() -> (w2444:string)
                    n1632 = call "currentScan.vi"("Imax"=w2451, "VISA resource name"=w2452) -> ("max"=w2450:bool, "Istring"=w2443:string, "Ichart"=→"FanCurrent":dbl)  [unwired: 6 in, 1 out]
                    "Ifan" <- w2443
                    "limitFan" <- w2450
                    n1633 = case shown="\"On\"" w2444 {
                      tunnel: [FALSE w2463 "FAN1"] -> w2442
                      tunnel: w2443 -> [_ w2462 _]
                      frame "Off", Default {
                        # "Why would I be Off"
                      }
                      frame "On" {
                        w2461 = 1.0 ("default (0 DBL)")
                        # "Lower limit control"
                        n1634 = global read "Global_1259.vi" "BaseCurrent"() -> (w2460:string)
                        n1635 = Fract/Exp String To Number(string=w2460, default (0 dbl)=w2461) -> (number=w2457:dbl)  [unwired: 2 in, 1 out]
                        n1636 = Multiply(x=w2457, y=0.05) -> (x*y=w2458:dbl)
                        n1637 = Add(x=w2457, y=w2458) -> (x+y=w2456:dbl)
                        n1638 = Fract/Exp String To Number(string=w2462, default (0 dbl)=w2461) -> (number=w2464:dbl)  [unwired: 2 in, 1 out]
                        n1639 = Less Or Equal?(x=w2464, y=w2456) -> (x <= y?=w2463:bool)
                      }
                      frame "Battery" {
                      }
                    }
                    n1640 = Not(x=w2450) -> (.not. x?=w2447:bool)
                    n1641 = Not(x="FAN0") -> (.not. x?=w2448:bool)
                    n1642 = call "currentPeak.vi"("Istring# change"=w2446, "Istring# scan"=w2443) -> ("Ipeak"=w2441:string)  [unwired: 7 in, 2 out]
                    "fanIPeak" <- w2441
                    n1643 = Compound Arithmetic op=OR(w2442, "FAN0", w2450) -> (w2454:bool)
                    n1644 = Compound Arithmetic op=AND(w2442, w2448, w2447) -> (w2449:bool)
                    n1645 = local write "FAN1"(w2442) -> ()
                  }
                }
              }
            }
            n1646 = local read "refnum out"() -> (w2399:refnum<file>)
            n1647 = call "dataSampled.vi"("Data"=w2397, "refnum in"=w2399) -> ("error out"=w2394:errorcluster)  [unwired: 8 in, 1 out]
            n1648 = call "Wait.vi"("error in (no error)"=w2394, "milliseconds to wait"=u32 1500) -> ()  [unwired: 8 in, 2 out]
          }
        }
        n1649 = Select(t=T3."Audio" ("Tab Control"), s=w2366, f=T3."Failed" ("Tab Control")) -> (s? t:f=w2365:T3)
      }
      frame "Audio" {
        w2468 = FALSE
        n1650 = local write "limitAudio"(w2468) -> ()
        n1651 = local write "AUD1 2"(w2468) -> ()
        n1652 = local write "AUD0 2"(w2468) -> ()
        n1653 = local write "AUD0"(w2468) -> ()
        n1654 = local write "AUD1"(w2468) -> ()
        n1655 = stacked-sequence {
          tunnel: [_ w2476] -> w2466
          frame #0 {
            # "clear values"
            n1656 = disable-structure shown="Enabled" {
              frame Disabled {
              }
              frame Enabled {
                w2475 = "0.00" ("Ipeak")
                n1657 = property on="AudioCurrent" class="WFChart (strict)"("History Data"=dbl[] []) -> ()  [unwired: 2 in, 2 out]
                n1658 = local write "audioIPeak"(w2475) -> ()
                n1659 = global write "Global_1259.vi" "runCurrent"(w2475) -> ()
                n1660 = local write "Iaudio"(w2475) -> ()
              }
            }
          }
          frame #1 {
            n1661 = case shown="True" TRUE {
              tunnel: [TRUE w2479] -> w2476
              frame False {
                # "This is for debugging"
              }
              frame True {
                # "Protocol Check"
                # "Feature Check"
                n1662 = global read "Global_1259.vi" "maxCurrent"() -> (w2492:string)
                "currentMaxAudio" <- w2492
                n1663 = local read "EQF1259 com port"() -> (w2490:refnum<visa-resource-name>)
                n1664 = Fract/Exp String To Number(string=w2492) -> (number=w2488:dbl)  [unwired: 3 in, 1 out]
                n1665 = property on="AudioCurrent" class="WFChart (strict)"("YScale.Maximum"=w2488) -> ()  [unwired: 2 in, 2 out]
                n1666 = call "1259_usbUart.vi"("VISA resource name"=w2490, "write buffer"="`\u0002", "sdFeature"=FALSE) -> ("number[0]"=w2491:u32)  [unwired: 1 in, 15 out]
                n1667 = global read "Global_1259.vi" "AUDIO"() -> (w2487:string)
                n1668 = Number To Decimal String(number=w2491) -> (decimal integer string=w2489:string)  [unwired: 1 in]
                n1669 = global write "Global_1259.vi" "audioType"(w2489) -> ()
                n1670 = Not Equal?(x=w2489, y="1") -> (x != y?=w2486:bool)
                n1671 = Not Equal?(x=w2487, y="0") -> (x != y?=w2485:bool)
                n1672 = Compound Arithmetic op=AND(w2486, w2485, TRUE ("value")) -> (w2479:bool)
                n1673 = global write "Global_1259.vi" "tempBoolean"(w2479) -> ()
              }
            }
          }
        }
        n1674 = case shown="True" w2466 {
          tunnel: [TRUE w2496] -> w2467
          frame False {
            n1675 = local read "refnum out"() -> (w2494:refnum<file>)
            n1676 = call "dataSampled.vi"("refnum in"=w2494) -> ()  [unwired: 9 in, 2 out]
          }
          frame True {
            n1677 = stacked-sequence {
              tunnel: [_ _ w2549] -> w2495
              frame #0 {
                n1678 = call "audio_tvPIP.vi"() -> ("AUDIO-19"=→"AUDIO-19":string)  [unwired: 9 in, 2 out]
                n1679 = disable-structure shown="Disabled" {
                  frame Disabled {
                    # "Scan for current to \nreturn to run state"
                    n1680 = while {
                      shift-right: [w2506] -> _
                      shift-left: _ -> [w2504]
                      stop <- w2503 stop-if-true
                      n1681 = Fract/Exp String To Number(string=w2504) -> (number=w2502:dbl)  [unwired: 3 in, 1 out]
                      n1682 = global read "Global_1259.vi" "BaseCurrent"() -> (w2505:string)
                      n1683 = Fract/Exp String To Number(string=w2505) -> (number=w2501:dbl)  [unwired: 3 in, 1 out]
                      n1684 = global read "Global_1259.vi" "maxCurrent"() -> (w2498:string)
                      n1685 = local read "EQF1259 com port"() -> (w2507:refnum<visa-resource-name>)
                      n1686 = Multiply(x=1.01, y=w2501) -> (x*y=w2500:dbl)
                      n1687 = In Range and Coerce(upper limit=w2500, x=w2502, lower limit=w2501) -> (In Range?=w2503:bool)  [unwired: 1 out]
                      n1688 = call "currentScan.vi"("Imax"=w2498, "VISA resource name"=w2507) -> ("Istring"=w2506:string)  [unwired: 6 in, 3 out]
                    }
                  }
                  frame Enabled {
                  }
                }
              }
              frame #1 {
                n1689 = flat-sequence {
                  tunnel: [w2509] -> w2508
                  tunnel: w2508 -> [w2519]
                  frame #0 {
                    # "BLE Audio feature"
                    n1690 = while {
                      tunnel: [w2513] -> w2509
                      i -> [w2511]
                      stop <- w2514 stop-if-true
                      n1691 = global read "Global_1259.vi" "audioType"() -> (w2515:string)
                      n1692 = Index Array(array=string[] ["68", "100", "228"], index=w2511) -> (element=w2516:string)
                      n1693 = Equal?(x=w2516, y=w2515) -> (x = y?=w2513:bool)
                      n1694 = Equal?(x=3, y=w2511) -> (x = y?=w2512:bool)
                      n1695 = Or(x=w2513, y=w2512) -> (x .or. y?=w2514:bool)
                    }
                  }
                  frame #1 {
                    n1696 = global read "Global_1259.vi" "tempBoolean"() -> (w2518:bool)
                    n1697 = And(x=w2519, y=w2518) -> (x .and. y?=w2520:bool)
                    n1698 = case shown="True" w2520 {
                      frame False {
                        # "No BLE Audio feature"
                        n1699 = local write "AUD1 2"(TRUE ("AUD1 2")) -> ()
                      }
                      frame True {
                        n1700 = stacked-sequence {
                          frame #0 {
                            n1701 = while {
                              shift-right: [w2534] -> _
                              shift-left: _ -> [w2535]
                              tunnel: [w2527] -> w2522
                              stop <- w2526 stop-if-true
                              n1702 = local read "EQF1259 com port"() -> (w2533:refnum<visa-resource-name>)
                              n1703 = local read "currentMaxAudio"() -> (w2532:string)
                              n1704 = call "currentScan.vi"("Imax"=w2532, "VISA resource name"=w2533) -> ("max"=w2529:bool, "Istring"=w2534:string, "Ichart"=w2531:dbl)  [unwired: 6 in, 1 out]
                              n1705 = local write "AudioCurrent"(w2531) -> ()
                              n1706 = local write "limitAudio"(w2529) -> ()
                              n1707 = call "currentPeak.vi"("Istring# change"=w2535, "Istring# scan"=w2534) -> ("Ipeak"=w2530:string)  [unwired: 7 in, 2 out]
                              n1708 = local write "Iaudio"(w2530) -> ()
                              n1709 = local write "audioIPeak"(w2530) -> ()
                              n1710 = Or(x="AUD1 2", y="AUD0 2") -> (x .or. y?=w2526:bool)
                              n1711 = Not(x="AUD1 2") -> (.not. x?=w2523:bool)
                              n1712 = Compound Arithmetic op=AND(TRUE ("value"), w2523, "AUD0 2") -> (w2527:bool)
                            }
                            n1713 = local write "AUD0"(w2522) -> ()
                          }
                          frame #1 {
                            # "This may be the issue"
                            n1714 = disable-structure shown="Disabled" {
                              frame Disabled {
                                # "Scan for current to \nreturn to run state"
                                n1715 = while {
                                shift-right: [w2544] -> _
                                shift-left: _ -> [w2542]
                                stop <- w2541 stop-if-true
                                n1716 = Fract/Exp String To Number(string=w2542) -> (number=w2540:dbl)  [unwired: 3 in, 1 out]
                                n1717 = global read "Global_1259.vi" "BaseCurrent"() -> (w2543:string)
                                n1718 = Fract/Exp String To Number(string=w2543) -> (number=w2539:dbl)  [unwired: 3 in, 1 out]
                                n1719 = global read "Global_1259.vi" "maxCurrent"() -> (w2536:string)
                                n1720 = local read "EQF1259 com port"() -> (w2545:refnum<visa-resource-name>)
                                n1721 = Multiply(x=1.01, y=w2539) -> (x*y=w2538:dbl)
                                n1722 = In Range and Coerce(upper limit=w2538, x=w2540, lower limit=w2539) -> (In Range?=w2541:bool)  [unwired: 1 out]
                                n1723 = call "currentScan.vi"("Imax"=w2536, "VISA resource name"=w2545) -> ("Istring"=w2544:string)  [unwired: 6 in, 3 out]
                                }
                              }
                              frame Enabled {
                              }
                            }
                          }
                        }
                      }
                    }
                  }
                }
              }
              frame #2 {
                n1724 = case shown="False" FALSE {
                  tunnel: [w2551 w2568] -> w2547
                  tunnel: [w2550 w2567] -> w2549
                  frame False {
                    # "Changed to PASS instead of BATTERY due to lack of audio current draw data"
                    n1725 = disable-structure shown="Disabled" {
                      frame Disabled {
                        # "if (!Battery)\n{\n   current();\n}\nelse\n{\n   manual();\n}"
                        n1726 = global read "Global_1259.vi" "PowerMode"() -> (w2553:string)
                        n1727 = Not Equal?(x=w2553, y="Battery") -> ()  [unwired: 1 out]
                      }
                      frame Enabled {
                      }
                    }
                    n1728 = while {
                      shift-right: [w2565] -> _
                      shift-left: _ -> [w2566]
                      tunnel: [w2561] -> w2551
                      tunnel: [w2555] -> w2550
                      stop <- w2554 stop-if-true
                      n1729 = local read "EQF1259 com port"() -> (w2564:refnum<visa-resource-name>)
                      n1730 = local read "currentMaxAudio"() -> (w2563:string)
                      n1731 = call "currentScan.vi"("Imax"=w2563, "VISA resource name"=w2564) -> ("max"=w2560:bool, "Istring"=w2565:string, "Ichart"=w2562:dbl)  [unwired: 6 in, 1 out]
                      n1732 = local read "AUD0"() -> (w2557:bool)
                      n1733 = local write "AudioCurrent"(w2562) -> ()
                      n1734 = local write "limitAudio"(w2560) -> ()
                      n1735 = local read "AUD1"() -> (w2559:bool)
                      n1736 = call "currentPeak.vi"("Istring# change"=w2566, "Istring# scan"=w2565) -> ("Ipeak"=w2561:string)  [unwired: 7 in, 2 out]
                      n1737 = local write "Iaudio"(w2561) -> ()
                      n1738 = local write "audioIPeak"(w2561) -> ()
                      n1739 = Or(x=w2559, y=w2557) -> (x .or. y?=w2554:bool)
                      n1740 = Not(x=w2557) -> (.not. x?=w2558:bool)
                      n1741 = Compound Arithmetic op=AND(TRUE ("value"), w2559, w2558) -> (w2555:bool)
                    }
                  }
                  frame True {
                    n1742 = while {
                      tunnel: [w2574] -> w2567
                      tunnel: [w2573] -> w2568
                      shift-right: [w2571] -> _
                      shift-left: enum16{"High", "Low"}."High" -> [w2572]
                      stop <- w2570 stop-if-true
                      n1743 = case shown="\"High\", Default" w2572 {
                        tunnel: [w2577 w2609] -> w2574
                        tunnel: [w2576 w2606] -> w2573
                        tunnel: [enum16{"High", "Low"}."Low" enum16{"High", "Low"}."Low"] -> w2571
                        tunnel: [FALSE TRUE] -> w2570
                        frame "High", Default {
                          n1744 = while {
                            tunnel: [w2593] -> w2577
                            shift-right: [w2585] -> _
                            shift-left: _ -> [w2590]
                            tunnel: [w2583] -> w2576
                            stop <- w2594 stop-if-true
                            n1745 = local read "EQF1259 com port"() -> (w2581:refnum<visa-resource-name>)
                            n1746 = local read "currentMaxAudio"() -> (w2582:string)
                            n1747 = global read "Global_1259.vi" "PowerMode"() -> (w2589:string)
                            n1748 = local read "AUD0"() -> (w2587:bool)
                            n1749 = call "currentScan.vi"("Imax"=w2582, "VISA resource name"=w2581) -> ("error out"=w2579:errorcluster, "max"=w2584:bool, "Istring"=w2585:string, "Ichart"=w2586:dbl)  [unwired: 6 in]
                            n1750 = local write "AudioCurrent"(w2586) -> ()
                            n1751 = case shown="\"On\"" w2589 {
                              tunnel: [FALSE w2603 w2605] -> w2588
                              tunnel: w2585 -> [_ w2602 _]
                              frame "Off", Default {
                                # "Why would I be Off"
                              }
                              frame "On" {
                                w2601 = 1.0 ("default (0 DBL)")
                                # "Lower limit control"
                                n1752 = global read "Global_1259.vi" "BaseCurrent"() -> (w2600:string)
                                n1753 = Fract/Exp String To Number(string=w2600, default (0 dbl)=w2601) -> (number=w2597:dbl)  [unwired: 2 in, 1 out]
                                n1754 = Multiply(x=w2597, y=0.5) -> (x*y=w2598:dbl)
                                n1755 = Add(x=w2597, y=w2598) -> (x+y=w2596:dbl)
                                n1756 = Fract/Exp String To Number(string=w2602, default (0 dbl)=w2601) -> (number=w2604:dbl)  [unwired: 2 in, 1 out]
                                n1757 = Greater Or Equal?(x=w2604, y=w2596) -> (x >= y?=w2603:bool)
                              }
                              frame "Battery" {
                                n1758 = local read "AUD1"() -> (w2605:bool)
                              }
                            }
                            n1759 = local write "limitAudio"(w2584) -> ()
                            n1760 = Not(x=w2587) -> (.not. x?=w2592:bool)
                            n1761 = Not(x=w2584) -> (.not. x?=w2591:bool)
                            n1762 = call "currentPeak.vi"("error in (no error)"=w2579, "Istring# change"=w2590, "Istring# scan"=w2585) -> ("Ipeak"=w2583:string, "Irun"=w2580:string)  [unwired: 6 in, 1 out]
                            n1763 = local write "Iaudio"(w2580) -> ()
                            n1764 = local write "audioIPeak"(w2583) -> ()
                            n1765 = Compound Arithmetic op=OR(w2588, w2587, w2584) -> (w2594:bool)
                            n1766 = Compound Arithmetic op=AND(w2588, w2592, w2591) -> (w2593:bool)
                          }
                        }
                        frame "Low" {
                          n1767 = while {
                            tunnel: [w2622] -> w2609
                            shift-right: [w2617] -> _
                            shift-left: _ -> [w2619]
                            tunnel: [w2610] -> w2606
                            stop <- w2624 stop-if-true
                            n1768 = local read "EQF1259 com port"() -> (w2615:refnum<visa-resource-name>)
                            n1769 = local read "currentMaxAudio"() -> (w2614:string)
                            n1770 = global read "Global_1259.vi" "PowerMode"() -> (w2618:string)
                            n1771 = call "currentScan.vi"("Imax"=w2614, "VISA resource name"=w2615) -> ("max"=w2623:bool, "Istring"=w2617:string, "Ichart"=→"AudioCurrent":dbl)  [unwired: 6 in, 1 out]
                            "limitAudio" <- w2623
                            n1772 = case shown="\"On\"" w2618 {
                              tunnel: [FALSE w2633 "AUD1"] -> w2611
                              tunnel: w2617 -> [_ w2632 _]
                              frame "Off", Default {
                                # "Why would I be Off"
                              }
                              frame "On" {
                                w2631 = 1.0 ("default (0 DBL)")
                                # "Lower limit control"
                                n1773 = global read "Global_1259.vi" "BaseCurrent"() -> (w2630:string)
                                n1774 = Fract/Exp String To Number(string=w2630, default (0 dbl)=w2631) -> (number=w2627:dbl)  [unwired: 2 in, 1 out]
                                n1775 = Multiply(x=w2627, y=0.05) -> (x*y=w2628:dbl)
                                n1776 = Add(x=w2627, y=w2628) -> (x+y=w2626:dbl)
                                n1777 = Fract/Exp String To Number(string=w2632, default (0 dbl)=w2631) -> (number=w2634:dbl)  [unwired: 2 in, 1 out]
                                n1778 = Less Or Equal?(x=w2634, y=w2626) -> (x <= y?=w2633:bool)
                              }
                              frame "Battery" {
                              }
                            }
                            n1779 = Not(x=w2623) -> (.not. x?=w2620:bool)
                            n1780 = Not(x="AUD0") -> (.not. x?=w2621:bool)
                            n1781 = call "currentPeak.vi"("Istring# change"=w2619, "Istring# scan"=w2617) -> ("Ipeak"=w2610:string, "Irun"=→"Iaudio":string)  [unwired: 7 in, 1 out]
                            "audioIPeak" <- w2610
                            n1782 = Compound Arithmetic op=OR(w2611, "AUD0", w2623) -> (w2624:bool)
                            n1783 = Compound Arithmetic op=AND(w2611, w2621, w2620) -> (w2622:bool)
                            n1784 = local write "AUD1"(w2611) -> ()
                          }
                        }
                      }
                    }
                  }
                }
                n1785 = local read "refnum out"() -> (w2548:refnum<file>)
                n1786 = call "dataSampled.vi"("Data"=w2547, "refnum in"=w2548) -> ()  [unwired: 8 in, 2 out]
              }
            }
            n1787 = case shown="True" w2495 {
              selector: w2495 -> [w2636 w2637]
              tunnel: [w2636 w2637] -> w2496
              frame False {
                # "Do nothing"
              }
              frame True {
                n1788 = disable-structure shown="Disabled" {
                  frame Disabled {
                    # "Scan for current to \nreturn to run state"
                    n1789 = while {
                      shift-right: [w2646] -> _
                      shift-left: _ -> [w2644]
                      stop <- w2643 stop-if-true
                      n1790 = Fract/Exp String To Number(string=w2644) -> (number=w2642:dbl)  [unwired: 3 in, 1 out]
                      n1791 = global read "Global_1259.vi" "BaseCurrent"() -> (w2645:string)
                      n1792 = Fract/Exp String To Number(string=w2645) -> (number=w2641:dbl)  [unwired: 3 in, 1 out]
                      n1793 = global read "Global_1259.vi" "maxCurrent"() -> (w2638:string)
                      n1794 = local read "EQF1259 com port"() -> (w2647:refnum<visa-resource-name>)
                      n1795 = Multiply(x=1.05, y=w2641) -> (x*y=w2640:dbl)
                      n1796 = In Range and Coerce(upper limit=w2640, x=w2642, lower limit=w2641) -> (In Range?=w2643:bool)  [unwired: 1 out]
                      n1797 = call "currentScan.vi"("Imax"=w2638, "VISA resource name"=w2647) -> ("Istring"=w2646:string)  [unwired: 6 in, 3 out]
                    }
                  }
                  frame Enabled {
                  }
                }
              }
            }
          }
        }
        n1798 = Select(t=T3."TV" ("Tab Control"), s=w2467, f=T3."Failed" ("Tab Control")) -> (s? t:f=w2473:T3)
      }
      frame "TV" {
        w2648 = "0.00" ("USB")
        w2656 = FALSE
        n1799 = local write "Itv"(w2648) -> ()
        n1800 = local write "TV1"(w2656) -> ()
        n1801 = local write "TV0"(w2656) -> ()
        n1802 = property on="TVCurrent" class="WFChart (strict)"("History Data"=dbl[] []) -> ()  [unwired: 2 in, 2 out]
        n1803 = local write "tvIPeak"(w2648) -> ()
        n1804 = global write "Global_1259.vi" "runCurrent"(w2648) -> ()
        n1805 = local write "limitTV"(w2656) -> ()
        n1806 = while {
          shift-right: [w2661] -> _
          shift-left: 0 -> [w2662]
          tunnel: [w2660] -> w2651
          stop <- w2659 stop-if-true
          n1807 = case shown="0, Default" w2662 {
            tunnel: [1 _] -> w2661
            tunnel: [FALSE w2672] -> w2660
            tunnel: [FALSE TRUE] -> w2659
            frame 0, Default {
              n1808 = global read "Global_1259.vi" "maxCurrent"() -> (w2664:string)
              "currentMaxTV" <- w2664
              n1809 = Fract/Exp String To Number(string=w2664) -> (number=w2663:dbl)  [unwired: 3 in, 1 out]
              n1810 = property on="TVCurrent" class="WFChart (strict)"("YScale.Maximum"=w2663) -> ()  [unwired: 2 in, 2 out]
            }
            frame 1 {
              w2675 = 128
              n1811 = global read "Global_1259.vi" "audioType"() -> (w2678:string)
              n1812 = global read "Global_1259.vi" "TV"() -> (w2668:string)
              n1813 = Decimal String To Number(string=w2678) -> (number=w2676:i32)  [unwired: 2 in, 1 out]
              n1814 = Decimal String To Number(string=w2668) -> (number=w2677:i32)  [unwired: 2 in, 1 out]
              n1815 = global read "Global_1259.vi" "tabletType"() -> (w2669:string)
              n1816 = Greater Or Equal?(x=w2677, y=w2675) -> (x >= y?=w2680:bool)
              n1817 = Greater Or Equal?(x=w2676, y=w2675) -> (x >= y?=w2679:bool)
              n1818 = Compound Arithmetic op=OR(w2680, w2679) -> (w2674:bool)
              n1819 = Equal?(x="1", y=w2669) -> (x = y?=w2670:bool)
              n1820 = Or(x=w2670, y=w2674) -> (x .or. y?=w2672:bool)
            }
          }
        }
        n1821 = case shown="True" w2651 {
          tunnel: [TRUE w2685] -> w2658
          frame False {
            n1822 = local read "refnum out"() -> (w2681:refnum<file>)
            n1823 = call "dataSampled.vi"("refnum in"=w2681) -> ()  [unwired: 9 in, 2 out]
          }
          frame True {
            n1824 = while {
              tunnel: [w2703] -> w2685
              shift-right: [w2691] -> _
              shift-left: _ -> [w2689]
              tunnel: [w2690] -> w2683
              stop <- w2704 stop-if-true
              n1825 = global read "Global_1259.vi" "tabletType"() -> (w2688:string)
              n1826 = Equal?(x=w2688, y="1") -> (x = y?=w2694:bool)
              n1827 = case shown="True" w2694 {
                tunnel: [w2706 w2708] -> w2696
                tunnel: [w2705 _] -> w2693
                frame False {
                  n1828 = call "audio_tvPIP.vi"() -> ("error out"=w2705:errorcluster, "TV-20"=w2706:string)  [unwired: 9 in, 1 out]
                }
                frame True {
                  n1829 = global read "Global_1259.vi" "PIP_Instruction"() -> (w2707:string[][])
                  n1830 = Index Array(array=w2707, index (row)=1 ("disabled index (row)"), index (col)=20 ("disabled index (col)")) -> (element=w2708:string)
                }
              }
              "TV-20" <- w2696
              n1831 = local read "EQF1259 com port"() -> (w2700:refnum<visa-resource-name>)
              n1832 = local read "currentMaxTV"() -> (w2699:string)
              n1833 = call "currentScan.vi"("error in (no error)"=w2693, "Imax"=w2699, "VISA resource name"=w2700) -> ("max"=w2697:bool, "Istring"=w2691:string, "Ichart"=→"TVCurrent":dbl)  [unwired: 5 in, 1 out]
              "limitTV" <- w2697
              n1834 = Compound Arithmetic op=OR("TV0", "TV1", w2697) -> (w2704:bool)
              n1835 = Not(x="TV0") -> (.not. x?=w2692:bool)
              n1836 = Not(x=w2697) -> (.not. x?=w2698:bool)
              n1837 = call "currentPeak.vi"("Istring# change"=w2689, "Istring# scan"=w2691) -> ("Ipeak"=w2690:string, "Irun"=→"Itv":string)  [unwired: 7 in, 1 out]
              "tvIPeak" <- w2690
              n1838 = Compound Arithmetic op=AND(w2692, "TV1", w2698) -> (w2703:bool)
            }
            n1839 = local read "refnum out"() -> (w2684:refnum<file>)
            n1840 = call "dataSampled.vi"("Data"=w2683, "refnum in"=w2684) -> ()  [unwired: 8 in, 2 out]
          }
        }
        n1841 = Select(t=T3."USB" ("Tab Control"), s=w2658, f=T3."Failed" ("Tab Control")) -> (s? t:f=w2657:T3)
      }
      frame "USB" {
        w2711 = "0.00" ("USB")
        w2717 = FALSE
        n1842 = local write "FanCurrent"(0.0 ("CURRENT")) -> ()
        n1843 = local write "Iusb"(w2711) -> ()
        n1844 = property on="USBCurrent" class="WFChart (strict)"("History Data"=dbl[] []) -> ()  [unwired: 2 in, 2 out]
        n1845 = local write "USB0"(w2717) -> ()
        n1846 = local write "USB1"(w2717) -> ()
        n1847 = local write "usbIPeak"(w2711) -> ()
        n1848 = global write "Global_1259.vi" "runCurrent"(w2711) -> ()
        n1849 = local write "limitUSB"(w2717) -> ()
        n1850 = flat-sequence {
          tunnel: [w2729] -> w2716
          frame #0 {
            n1851 = global read "Global_1259.vi" "maxCurrent"() -> (w2722:string)
            "currentMaxUSB" <- w2722
            n1852 = local read "EQF1259 com port"() -> (w2723:refnum<visa-resource-name>)
            n1853 = Fract/Exp String To Number(string=w2722) -> (number=w2721:dbl)  [unwired: 3 in, 1 out]
            n1854 = property on="USBCurrent" class="WFChart (strict)"("YScale.Maximum"=w2721) -> ()  [unwired: 2 in, 2 out]
            n1855 = call "1259_usbUart.vi"("VISA resource name"=w2723, "write buffer"="c\u0001") -> ("number[0]"=w2725:u32)  [unwired: 2 in, 15 out]
            n1856 = Number To Decimal String(number=w2725) -> (decimal integer string=w2726:string)  [unwired: 1 in]
            n1857 = global write "Global_1259.vi" "usbType"(w2726) -> ()
          }
          frame #1 {
            n1858 = call "usbPIP.vi"() -> ("Boolean"=w2728:bool, "USB-16"=→"USB-16":string)  [unwired: 9 in, 1 out]
            n1859 = case shown="True" w2728 {
              tunnel: [TRUE w2734] -> w2729
              frame False {
                n1860 = local read "refnum out"() -> (w2730:refnum<file>)
                n1861 = call "dataSampled.vi"("refnum in"=w2730) -> ()  [unwired: 9 in, 2 out]
              }
              frame True {
                n1862 = while {
                  tunnel: [w2744] -> w2734
                  shift-right: [w2737] -> _
                  shift-left: _ -> [w2736]
                  tunnel: [w2735] -> w2732
                  stop <- w2747 stop-if-true
                  n1863 = local read "EQF1259 com port"() -> (w2742:refnum<visa-resource-name>)
                  n1864 = local read "currentMaxUSB"() -> (w2741:string)
                  n1865 = call "currentScan.vi"("Imax"=w2741, "VISA resource name"=w2742) -> ("max"=w2738:bool, "Istring"=w2737:string, "Ichart"=→"USBCurrent":dbl)  [unwired: 6 in, 1 out]
                  "limitUSB" <- w2738
                  n1866 = Compound Arithmetic op=OR("USB0", "USB1", w2738) -> (w2747:bool)
                  n1867 = Not(x="USB1") -> (.not. x?=w2748:bool)
                  n1868 = Not(x=w2738) -> (.not. x?=w2743:bool)
                  n1869 = call "currentPeak.vi"("Istring# change"=w2736, "Istring# scan"=w2737) -> ("Ipeak"=w2735:string, "Irun"=→"Iusb":string)  [unwired: 7 in, 1 out]
                  "usbIPeak" <- w2735
                  n1870 = Compound Arithmetic op=AND("USB0", w2748, w2743) -> (w2744:bool)
                }
                n1871 = local read "refnum out"() -> (w2733:refnum<file>)
                n1872 = call "dataSampled.vi"("Data"=w2732, "refnum in"=w2733) -> ()  [unwired: 8 in, 2 out]
              }
            }
          }
        }
        n1873 = Select(t=T3."Resistance" ("Tab Control"), s=w2716, f=T3."Failed" ("Tab Control")) -> (s? t:f=w2719:T3)
      }
      frame "CSafe" {
        w2756 = "0.00" ("runCurrent")
        w2762 = FALSE
        n1874 = local write "FanCurrent"(0.0 ("CURRENT")) -> ()
        n1875 = property on="CSafeCurrent" class="WFChart (strict)"("History Data"=dbl[] []) -> ()  [unwired: 2 in, 2 out]
        n1876 = local write "Icsafe"(w2756) -> ()
        n1877 = local write "CSA0"(w2762) -> ()
        n1878 = local write "CSA1"(w2762) -> ()
        n1879 = local read "EQF1259 com port"() -> (w2757:refnum<visa-resource-name>)
        n1880 = local write "csafeIPeak"(w2756) -> ()
        n1881 = global write "Global_1259.vi" "runCurrent"(w2756) -> ()
        n1882 = local write "limitCSafe"(w2762) -> ()
        n1883 = call "currentMax.vi"("VISA Refnum in"=w2757) -> ("stringCurrentMax"=→"currentMaxCSafe":string, "numberCurrentMax"=w2759:dbl)  [unwired: 8 in, 1 out]
        n1884 = property on="CSafeCurrent" class="WFChart (strict)"("YScale.Maximum"=w2759) -> ()  [unwired: 2 in, 2 out]
        n1885 = global read "Global_1259.vi" "CSAFE"() -> (w2761:string)
        n1886 = Not Equal?(x=w2761, y="0") -> (x != y?=w2765:bool)
        n1887 = case shown="False" w2765 {
          tunnel: [TRUE w2775] -> w2768
          frame False {
            n1888 = local read "refnum out"() -> (w2770:refnum<file>)
            n1889 = Write to Text File(file (use dialog)=w2770, text="NULL" ("Data")) -> ()  [unwired: 2 in, 3 out]
          }
          frame True {
            n1890 = call "csafePIP.vi"() -> ("CSAFE-21"=→"CSAFE-21":string)  [unwired: 10 in, 1 out]
            n1891 = while {
              tunnel: [w2786] -> w2775
              shift-right: [w2781] -> _
              shift-left: _ -> [w2779]
              tunnel: [w2778] -> w2772
              stop <- w2789 stop-if-true
              n1892 = local read "EQF1259 com port"() -> (w2784:refnum<visa-resource-name>)
              n1893 = local read "currentMaxCSafe"() -> (w2783:string)
              n1894 = call "currentScan.vi"("Imax"=w2783, "VISA resource name"=w2784) -> ("error out"=w2782:errorcluster, "max"=w2780:bool, "Istring"=w2777:string, "Ichart"=→"CSafeCurrent":dbl)  [unwired: 6 in]
              "limitCSafe" <- w2780
              "Icsafe" <- w2777
              n1895 = Not(x="CSA1") -> (.not. x?=w2790:bool)
              n1896 = Not(x=w2780) -> (.not. x?=w2776:bool)
              n1897 = call "currentPeak.vi"("error in (no error)"=w2782, "Istring# change"=w2779, "Istring# scan"=w2777) -> ("Ipeak"=w2778:string, "Irun"=w2781:string)  [unwired: 6 in, 1 out]
              "csafeIPeak" <- w2778
              n1898 = Compound Arithmetic op=OR("CSA0", "CSA1", w2780) -> (w2789:bool)
              n1899 = Compound Arithmetic op=AND("CSA0", w2790, w2776) -> (w2786:bool)
            }
            n1900 = local read "refnum out"() -> (w2774:refnum<file>)
            n1901 = Write to Text File(file (use dialog)=w2774, text=w2772) -> ()  [unwired: 2 in, 3 out]
          }
        }
        n1902 = Greater?(x=w2753, y=1) -> (0:w2754:bool)
        n1903 = Select(t=T1."Another" ("Tab Control"), s=w2754, f=T1."Finish" ("Tab Control")) -> (s? t:f=w2750:T1)
        n1904 = Select(t=w2750, s=w2768, f=T1."Failed" ("Tab Control")) -> (s? t:f=w2764:T1)
      }
      frame "Wahoo" {
        w2793 = "0.00" ("runCurrent")
        w2801 = FALSE
        # "This is tested as a BLE connection and HRM test"
        n1905 = local write "FanCurrent"(0.0 ("CURRENT")) -> ()
        n1906 = global write "Global_1259.vi" "runCurrent"(w2793) -> ()
        n1907 = local write "Iwahoo"(w2793) -> ()
        n1908 = local write "wahooIPeak"(w2793) -> ()
        n1909 = property on="WahooCurrent" class="WFChart (strict)"("History Data"=dbl[] []) -> ()  [unwired: 2 in, 2 out]
        n1910 = local write "WAH0"(w2801) -> ()
        n1911 = local write "WAH1"(w2801) -> ()
        n1912 = local read "EQF1259 com port"() -> (w2796:refnum<visa-resource-name>)
        n1913 = local write "limitWahoo"(w2801) -> ()
        n1914 = call "currentMax.vi"("VISA Refnum in"=w2796) -> ("stringCurrentMax"=→"currentMaxWahoo":string, "numberCurrentMax"=w2795:dbl)  [unwired: 8 in, 1 out]
        n1915 = property on="WahooCurrent" class="WFChart (strict)"("YScale.Maximum"=w2795) -> ()  [unwired: 2 in, 2 out]
        n1916 = global read "Global_1259.vi" "WAHOO"() -> (w2800:string)
        n1917 = Not Equal?(x=w2800, y="0" ("WAHOO")) -> (x != y?=w2803:bool)
        n1918 = case shown="True" w2803 {
          tunnel: [TRUE w2812] -> w2799
          frame False {
            n1919 = local read "refnum out"() -> (w2807:refnum<file>)
            n1920 = call "dataSampled.vi"("refnum in"=w2807) -> ()  [unwired: 9 in, 2 out]
          }
          frame True {
            n1921 = call "wahooPIP.vi"() -> ("WAHOO-22"=→"WAHOO-22":string)  [unwired: 10 in, 1 out]
            n1922 = while {
              tunnel: [w2823] -> w2812
              tunnel: [w2817] -> w2809
              shift-right: [w2816] -> _
              shift-left: _ -> [w2815]
              stop <- w2826 stop-if-true
              n1923 = local read "currentMaxWahoo"() -> (w2821:string)
              n1924 = local read "EQF1259 com port"() -> (w2820:refnum<visa-resource-name>)
              n1925 = call "currentScan.vi"("Imax"=w2821, "VISA resource name"=w2820) -> ("error out"=w2822:errorcluster, "max"=w2818:bool, "Istring"=w2814:string, "Ichart"=→"WahooCurrent":dbl)  [unwired: 6 in]
              "Iwahoo" <- w2814
              "limitWahoo" <- w2818
              n1926 = Not(x="WAH1") -> (.not. x?=w2827:bool)
              n1927 = Not(x=w2818) -> (.not. x?=w2813:bool)
              n1928 = Compound Arithmetic op=OR("WAH0", "WAH1", w2818) -> (w2826:bool)
              n1929 = call "currentPeak.vi"("error in (no error)"=w2822, "Istring# change"=w2815, "Istring# scan"=w2814) -> ("Ipeak"=w2817:string, "Irun"=w2816:string)  [unwired: 6 in, 1 out]
              "wahooIPeak" <- w2817
              n1930 = Compound Arithmetic op=AND("WAH0", w2827, w2813) -> (w2823:bool)
            }
            n1931 = local read "refnum out"() -> (w2811:refnum<file>)
            n1932 = call "dataSampled.vi"("Data"=w2809, "refnum in"=w2811) -> ()  [unwired: 8 in, 2 out]
          }
        }
        n1933 = Select(t=T1."Finish" ("Tab Control"), s=w2799, f=T1."Failed" ("Tab Control")) -> (s? t:f=w2805:T1)
      }
      frame "Another" {
        w2841 = FALSE
        n1934 = Subtract(x=w2833, y=w2832) -> (x-y=→"# of Passed Samples":i32)
        n1935 = local write "ANO0"(w2841) -> ()
        n1936 = local write "ANO1"(w2841) -> ()
        n1937 = global read "Global_1259.vi" "PIC_ARRAY"() -> (w2836:picture[])
        n1938 = local read "refnum out"() -> (w2840:refnum<file>)
        n1939 = Index Array(array=w2836, index=3) -> (element=→"Another":picture)
        n1940 = Write to Text File(file (use dialog)=w2840, text="\r") -> ()  [unwired: 2 in, 3 out]
        n1941 = local read "EQF1259 com port"() -> (w2829:refnum<visa-resource-name>)
        n1942 = call "1259_usbCommand.vi"("write buffer"="\u0005\u0004", "VISA resource name in"=w2829) -> ("error out"=w2828:errorcluster)  [unwired: 8 in, 1 out]
        n1943 = while {
          tunnel: [w2844] -> w2843
          tunnel: w2828 -> [_]
          stop <- w2847 stop-if-true
          n1944 = Not(x="ANO0") -> (.not. x?=w2848:bool)
          n1945 = Compound Arithmetic op=OR("ANO1", "ANO0") -> (w2847:bool)
          n1946 = Compound Arithmetic op=AND("ANO1", w2848) -> (w2844:bool)
        }
        n1947 = Select(t=T3."Scan DUT" ("Tab Control"), s=w2843, f=T3."end" ("Tab Control")) -> (s? t:f=w2842:T3)
      }
      frame "Failed" {
        n1948 = call "Display Message to User6"() -> ()  [unwired: 10 in, 2 out]
        n1949 = Increment(x=w2856) -> (x+1=w2855:i32)
        "# of Failed Samples" <- w2855
        n1950 = global read "Global_1259.vi" "PIC_ARRAY"() -> (w2851:picture[])
        n1951 = local read "refnum out"() -> (w2860:refnum<file>)
        n1952 = local read "EQF1259 com port"() -> (w2857:refnum<visa-resource-name>)
        n1953 = Index Array(array=w2851, index=4) -> (element=→"Failed":picture)
        n1954 = call "dataSampled.vi"("Data"="FAILED" ("string"), "refnum in"=w2860) -> ()  [unwired: 8 in, 2 out]
        n1955 = call "1259_usbUart.vi"("VISA resource name"=w2857, "write buffer"="(\u0001", "sdFeature"=FALSE) -> ()  [unwired: 1 in, 16 out]
      }
      frame "end" {
        n1956 = while {
          shift-right: [w2866] -> _
          shift-left: 0 -> [w2868]
          stop <- w2867 stop-if-true
          n1957 = case shown="2" w2868 {
            tunnel: [FALSE _ _ TRUE] -> w2867
            tunnel: [1 2 3 _] -> w2866
            frame 0, Default {
              n1958 = global read "Global_1259.vi" "PIC_ARRAY"() -> (w2874:picture[])
              n1959 = Index Array(array=w2874, index=0) -> (element=→"Goodbye!":picture)
              n1960 = local write "Test Log"("") -> ()
            }
            frame 1 {
              n1961 = local read "refnum out"() -> (w2879:refnum<file>)
              n1962 = call "Close Data File and open.vi"("File Refnum In"=w2879) -> ("path"=w2878:path)  [unwired: 9 in, 1 out]
              n1963 = Path To String(path=w2878) -> (string=→"Test Log":string)
              n1964 = Wait (ms)(milliseconds to wait=u32 250) -> ()  [unwired: 1 out]
            }
            frame 2 {
              w2883 = "\""
              n1965 = Wait (ms)(milliseconds to wait=u32 250) -> ()  [unwired: 1 out]
              n1966 = local read "Test Log"() -> (w2882:string)
              n1967 = call <vilib>:"Space Constant.vi"() -> ("String"=w2888:string)
              n1968 = Concatenate Strings("cmd /c C:\\specsheetsConsole\\build\\exe.win-amd64-3.6\\labviewdbupload.exe ", w2888, w2883, w2882, w2883) -> (w2881:string)
              n1969 = call "exeCLI.vi"("Tab Control"=T2."Built-in command line utilities", "command line (built-in)"=w2881) -> ("standard error"=→"standard notepad":string)  [unwired: 11 in, 2 out]
            }
            frame 3 {
              w2890 = "\""
              n1970 = local read "Test Log"() -> (w2891:string)
              n1971 = call <vilib>:"Space Constant.vi"() -> ("String"=w2895:string)
              n1972 = Concatenate Strings("C:\\Windows\\System32\\notepad.exe" ("Command"), w2895, w2890, w2891, w2890) -> (w2896:string)
              n1973 = call "exeCLI.vi"("Tab Control"=T2."Interactive applications", "command line (interactive)"=w2896) -> ("standard error"=→"standard labviewdbupload":string)  [unwired: 11 in, 2 out]
            }
          }
        }
      }
      frame "Finish" {
        n1974 = local write "FIN0"(FALSE ("FIN0")) -> ()
        n1975 = local read "EQF1259 com port"() -> (w2900:refnum<visa-resource-name>)
        n1976 = call "1259_usbUart.vi"("VISA resource name"=w2900, "write buffer"="Y\u0001", "sdFeature"=FALSE) -> ("number[0]"=w2901:u32)  [unwired: 1 in, 15 out]
        n1977 = case shown="4" w2901 {
          tunnel: [_ w2909 w2910 w2914 w2918] -> w2898
          frame 0, Default {
          }
          frame 1 {
            n1978 = global read "Global_1259.vi" "PIP_Instruction"() -> (w2908:string[][])
            n1979 = Index Array(array=w2908, index (row)=1, index (col)=25 ("disabled index (col)")) -> (element=w2909:string)
            n1980 = global write "Global_1259.vi" "FINISH-25"(w2909) -> ()
          }
          frame 2 {
            n1981 = global read "Global_1259.vi" "PIP_Instruction"() -> (w2913:string[][])
            n1982 = Index Array(array=w2913, index (row)=4, index (col)=25 ("disabled index (col)")) -> (element=w2910:string)
            n1983 = global write "Global_1259.vi" "FINISH-25"(w2910) -> ()
          }
          frame 3 {
            n1984 = global read "Global_1259.vi" "PIP_Instruction"() -> (w2917:string[][])
            n1985 = Index Array(array=w2917, index (row)=3, index (col)=25 ("disabled index (col)")) -> (element=w2914:string)
            n1986 = global write "Global_1259.vi" "FINISH-25"(w2914) -> ()
          }
          frame 4 {
            n1987 = global read "Global_1259.vi" "PIP_Instruction"() -> (w2921:string[][])
            n1988 = Index Array(array=w2921, index (row)=1, index (col)=25 ("disabled index (col)")) -> (element=w2918:string)
            n1989 = global write "Global_1259.vi" "FINISH-25"(w2918) -> ()
          }
        }
        "FINISH-25" <- w2898
        n1990 = while {
          tunnel: [T1."Another" ("Tab Control")] -> w2903
          stop <- "FIN0" stop-if-true
        }
      }
    }
  }
